vi "myRIO_BRig_RT_v0,61__PortC.vi"() -> ()   [LabVIEW 2014]
uses:
  myRIO_BRig_RT__Case_Exp_stateList.ctl
  myRIO_BRig_RT__Case_NonExp_stateList.ctl
  <vilib>/Platform/TimedLoop/XDataNode/timing_clust.ctl
  <vilib>/Platform/TimedLoop/XDataNode/nitl_modes.ctl
  <vilib>/Platform/TimedLoop/XDataNode/wakeup.ctl
  <vilib>/WebDAVClient/Advanced/SessionHandle.ctl
  <vilib>/myRIO/Common/Instrument Driver Framework/myRIO v1.0/UART/vis/myRIO v1.0 Close UART.vi
  <vilib>/FPGAPlugInAG/myRIO-1900/niLvFpga_Open_myRIO-1900.vi
  <vilib>/rvi/interface/common/dynamic/niFpgaDynamicAddResources.vi
  <vilib>/Utility/error.llb/Error Cluster From Error Code.vi
  <vilib>/rvi/errors/niLvFpgaAdjustHostInterfaceError.vi
  <vilib>/FPGAPlugInAG/Dynamic/niLvFpga_Close_Dynamic.vi
  <vilib>/myRIO/Common/Instrument Driver Framework/Utilities/vis/FPGA Ref Manager.vi
  <vilib>/myRIO/Common/Instrument Driver Framework/myRIO v1.0/myRIO v1.0 Reset FPGA.vi
  <vilib>/myRIO/Common/Instrument Driver Framework/myRIO v1.0/IRQ/vis/myRIO v1.0 IRQ Info FGV.vi
  <vilib>/myRIO/Common/Instrument Driver Framework/myRIO v1.0/IRQ/vis/myRIO v1.0 Timer IRQ Info FGV.vi
  <vilib>/myRIO/Common/Instrument Driver Framework/myRIO v1.0/IRQ/vis/myRIO v1.0 ISR Agent.vi
  <vilib>/rvi/interface/nirviOpenFPGA/nirviOpenFPGA.xnode
  FPGA Bitfiles/myRIOBRig_FPGATarget_myRIOBRigFPGAv3,_rBLkV1r30v0.lvbitx
  myRIO_BRig_FPGA_v3,51__PortC__testSinwave.vi
  <vilib>/rvi/interface/nirviReadWriteControl/nirviReadWriteControl.xnode
  <vilib>/Platform/TimedLoop/XDataNode/XDataNode.xnode
  <vilib>/rvi/interface/nirviCloseFPGA/nirviCloseFPGA.xnode
  <vilib>/Platform/TimedLoop/XDataNode/XDNodeRunTimeDep.lvlib
  <vilib>/rvi/interface/Simulation/niFpgaSimulationCallBeginRW.vi
  <vilib>/myRIO/Instrument Drivers/Utilities/Utilities.lvlib
  <vilib>/WebDAVClient/NI_WebDAV.lvlib
  NiFpgaLv.dll
panel:
  out "error out 5":errorcluster
  in  "get_countPerMS":bool
  in  "count_warmup_R_reset":bool
  in  "count_warmup_L_reset":bool
  out "count_warmup_R":u16
  out "count_warmup_L":u16
  out "SolenoidReward":bool
  in  "SolenoidProbability_L":u16=50 caption="Reward Time [ms]" min=1 max=1000 step=1
  in  "SolenoidProbability_R":u16=50 caption="Reward Time [ms]" min=1 max=1000 step=1
  out "output_PortA":dbl
  out "error out 4":errorcluster
  in  "laser_power_step":dbl
  in  "laser_power_max":dbl
  in  "Recording_p2":bool
  in  "Recording":bool
  out "error out 3":errorcluster
  out "error out 2":errorcluster
  in  "laser_power_min":dbl
  in  "f_millisec2count":dbl=159.0
  in  "laser_Tshutter":dbl=2.0
  in  "laser_Freq":dbl=10.0
  in  "laser_Tpeak":dbl=2.0
  in  "laser_duration":u16
  out "error out":errorcluster
  in  "LC_Cue1_All_Count":u16
  in  "LC_Cue1_First_Count":u16
  in  "LC_Cue1_All_delayOpt":bool
  in  "LC_ENL1_All_delayOpt":bool
  in  "LC_ENL1_All_Count":u16
  in  "LC_ENL1_First_Count":u16
  in  "LC_Cue1_First_delayOpt":bool
  in  "LC_ENL1_First_delayOpt":bool
  in  "Tcycle_Cue_max":u16=1000 caption="Max" min=5 max=5000 step=5
  in  "Tcycle_Cue_min":u16=1000 caption="Min" min=5 max=5000 step=5
  in  "SendData":bool
  out "cSpout":enum16{"Left", "Right"}(ring) caption="Left or Right Spout"
  out "A4":u32 caption="LickCounter_Right"
  out "A2":u32 caption="LickCounter_Left"
  in  "laserResponse_wrong_LED":bool
  out "error_initTrial":errorcluster
  out "error_Selection_pre":errorcluster
  out "error_Selection":errorcluster
  out "SelectWrong":bool
  out "SelectReward":bool
  in  "Left(F)_or_Right(T)":bool
  in  "ignoreWrong":bool
  in  "SelectionState":bool
  in  "laserResponse_wrong":bool
  in  "laserResponse_reward":bool
  in  "laserResponse_reward_LED":bool
  out "nRewards_Right":u16 caption="# Rewards Total (Right)"
  out "nRewards_Left":u16 caption="# Rewards Total (Left)"
  out "nRewards_cur":u16 caption="# Rewards in Current Block"
  out "TpB_target":u16 caption="Target Trials Per Block"
  out "cState_NonExp":T1 caption="WarmUp State"
  out "iBlock":u16 caption="Current Block"
  out "cState":T2 caption="Experimental State"
  out "iTrial":u16 caption="Current Trial"
  in  "warmupType":u8(slide) max=2 step=1 scale=0.0..2.0
  in  "TestConnection":bool
  in  "warmup":bool caption="WarmUp"
  in  "Data Set Prefix":string="Exp1_TM2"
  out "Connected To Host?":bool
  in  "Host Password":string="sabalab"
  in  "Host UserName":string="Test2"
  in  "sp_RightSpout":u16(slide)=2 max=2 step=1 scale=0.0..2.0
  in  "sp_LeftSpout":u16(slide)=2 max=2 step=1 scale=0.0..2.0
  in  "BUR_max":u16 caption="Count Reward Structure  (0 = off)"
  in  "LC_Wrong_Probability":u16
  in  "LC_Wrong_Trial":u16(slide) max=2 step=1 scale=0.0..2.0
  in  "LC_Wrong_Block":u16(slide) max=2 step=1 scale=0.0..2.0
  in  "LC_Wrong_OnOff":bool
  in  "LC_Reward_Probability":u16
  in  "LC_Reward_Trial":u16(slide) max=2 step=1 scale=0.0..2.0
  in  "LC_Reward_Block":u16(slide) max=2 step=1 scale=0.0..2.0
  in  "LC_Reward_OnOff":bool
  in  "LC_Cue1_All_Probability":u16
  in  "LC_Cue1_All_Block":u16(slide) max=2 step=1 scale=0.0..2.0
  in  "LC_Cue1_All_OnOff":bool
  in  "LC_Cue1_First_Probability":u16
  in  "LC_Cue1_First_Block":u16(slide) max=2 step=1 scale=0.0..2.0
  in  "LC_Cue1_First_OnOff":bool
  in  "LC_ENL1_All_Probability":u16 max=100 step=1
  in  "LC_ENL1_All_Block":u16(slide) max=2 step=1 scale=0.0..2.0
  in  "LC_ENL1_All_OnOff":bool
  in  "LC_ENL1_First_Probability":u16 max=100 step=1
  in  "LC_ENL1_First_Block":u16(slide) max=2 step=1 scale=0.0..2.0
  in  "Tcycle_Timeout":u16=1000 caption="Timeout Time [ms]" min=10 max=10000 step=1
  in  "Tcycle_Wrong":u16=1000 caption="Wrong Time [ms]" min=10 max=10000 step=1
  in  "Tcycle_Selection":u16=1000 caption="Answer Time [ms]" min=1 max=10000 step=1
  in  "Tcycle_RewardPost":u16=1000 caption="Consumption Time [ms]" min=250 max=10000 step=250
  in  "Tcycle_Reward_L":u16=500 caption="Reward Time [ms]" min=1 max=1000 step=1
  in  "Tcycle_Reward_R":u16=500 caption="Reward Time [ms]" min=1 max=1000 step=1
  in  "TpB_Max_R":u16=4 caption="Max TrialsPerBlock" min=1 max=12 step=1
  in  "TpB_Min_R":u16=4 caption="Min TrialsPerBlock" min=1 max=12 step=1
  in  "TpB_Max_L":u16=4 caption="Max TrialsPerBlock" min=1 max=12 step=1
  in  "TpB_Min_L":u16=4 caption="Min TrialsPerBlock" min=1 max=12 step=1
  in  "BUR_min":u16 caption="Count Reward Structure  (0 = off)"
  in  "TrialUntilReward":bool caption="Ignore Wrong Selection"
  in  "CueCycles":u16=1 caption="Cue Structure" min=1 max=1 step=1
  in  "MTrig_Laser_Tcycle":u16=10 caption="Time [ms]"
  in  "MTrig_Laser_trig":bool
  in  "MTrig_Audio_trig__R":bool caption="Trigger Audio"
  in  "MTrig_Audio_trig__L":bool caption="Trigger Audio"
  in  "RewCalib_Trig_R":bool caption="Calibrate_R"
  in  "RewCalib_Trig_L":bool caption="Calibrate_L"
  in  "MTrig_Solenoid_Tcycle__R":u16=300 caption="Time [ms]"
  in  "MTrig_Solenoid_Tcycle__L":u16=300 caption="Time [ms]"
  in  "MTrig_Solenoid_trig__R":bool caption="Solenoid"
  in  "MTrig_Solenoid_trig__L":bool caption="Solenoid"
  in  "STOP_abort":bool caption="Stop LabView\n(Stops myRio and FPGA)"
  in  "STOP_endBlock":bool caption="Stop Experiment\n@ End of Block"
  in  "STOP_endTrial":bool caption="Stop Experiment\n@ End of Trial"
  in  "START":bool caption="Start Experiment"
  in  "Tcycle_CuePenalty":u16=1000 caption="Penalty" min=1 max=10000 step=1
  in  "Audio_Amp__R":u16=100 caption="Amp"
  in  "Audio_Freq__R":u8=5 caption="Freq [kHz]" max=14 step=1
  in  "Audio_Amp__L":u16=100 caption="Amp"
  in  "Audio_Freq__L":u8=5 caption="Freq [kHz]" max=14 step=1
  in  "LC_Wrong_Tdelay":u16
  in  "LC_Cue1_All_Tdelay":u16
  in  "LC_ENL1_All_Tdelay":u16
  in  "LC_Reward_Tdelay":u16
  in  "LC_Cue1_First_Tdelay":u16
  in  "LC_ENL1_First_Tdelay":u16
  in  "LC_ENL1_First_OnOff":bool
  in  "Tcycle_ENLPenalty":u16=100 caption="Penalty" min=10 max=10000 step=10
  in  "Tcycle_ENL_max":u16=1000 caption="Max" min=250 max=10000 step=250
  in  "Tcycle_ENL_min":u16=1000 caption="Min" min=250 max=10000 step=250
  # "Communication (Host PC)"
  # "WarmUp"
  # "Experimental Run"
  # "Current State"
  # "Laser Control\n\n                               On/Off      Block        Probability [%]   Delay [ms]                              Count"
  # "Cue then reward (no lick)\n \nLeft                    Right"
  # "Recording Rig"
  # "FPGA Conv."
  # "Enforced\nNonLick\n      1"
  # "from end"
  # "Switch\nTrial"
  # "FPGA count per ms"
  # "from start"
  # "from end"
  # "NonSwitch\nTrials"
  # "from start"
  # "Manual Control"
  # "Cue 1"
  # "Solenoid\n \nLeft                    Right"
  # "Speaker\n \nLeft                    Right"
  # "Laser"
  # "from end"
  # "Switch\nTrial"
  # "from start"
  # "from end"
  # "NonSwitch\nTrials"
  # "from start"
  # "Time = Cue Min"
  # "Selection Reward"
  # "Task Timing [ms]"
  # "Speaker Settings"
  # "Laser Settings"
  # "Selection Wrong"
  # "Left                  Right"
  # "Enforced NonLick"
  # "Frequency\n[kHz]"
  # "Duration         Frequency       Peak Width           Shutter\n    [ms]                   [Hz]                    [ms]                    [ms]"
  # "Task Structure"
  # "Spout Selection Control"
  # "Amp\n(0 - 32,000)"
  # "Master Structure"
  # "Cue"
  # "Answer Time\n         [ms]\n\n  \nWrong Choice Penalty\n         [ms]\n \n \nChoice Timeout Penalty\n         [ms]"
  # "Min\n \n  \nMax"
  # "Laser Power [V]\n      Min                   Max                   Step                 Current"
  # "Speaker\nPattern\nDuring Cue"
  # "(1) = Switching\n(2) = Two Choice"
  # "Reward Control\n                 Left              Right"
  # "Min"
  # "Max"
  # "Trial Per Block Structure\n       Left                    Right"
  # "Reward Time\n         [ms]\n\nWater Prob"
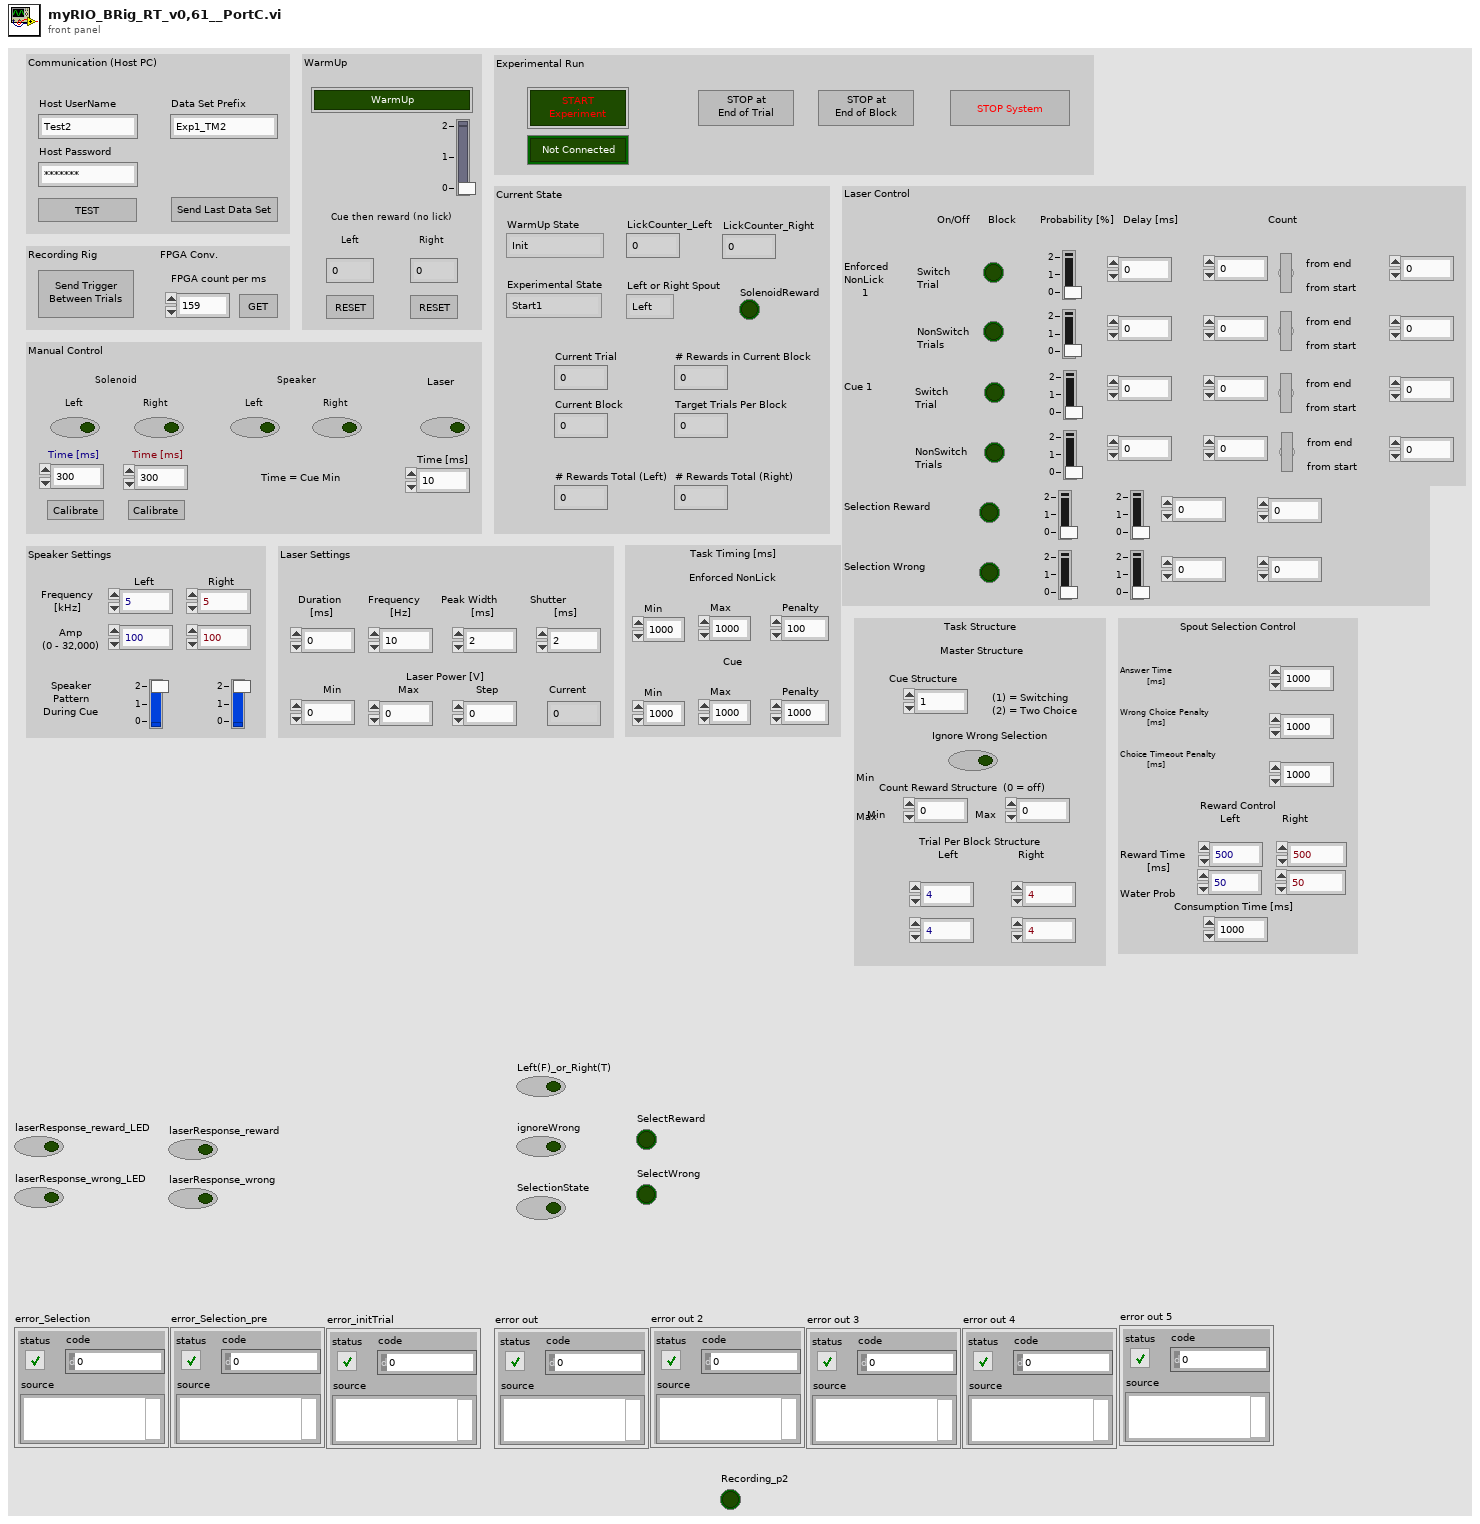
[diagram p1: front panel]
types:
  T1 = typedef "myRIO_BRig_RT__Case_NonExp_stateList.ctl" = enum16{"Init", "UploadSettings_pre", "UploadSettings_Read_dataExp", "UploadSettings_dataExp_1", "UploadSettings_Read_dataLC", "UploadSettings_dataLC_1", "UploadSettings_dataLC_2", "UploadSettings_Read_dataMTrig", "UploadSettings_dataMTrig_1", "UploadSettings_post", "Idle_pre", "IdleEmpty", "IdleEmpty2", "IdleEmpty3", "IdleEmpty4", "Idle", "Idle_2", "Idle_3", "Idle_4", "Idle_post", "Cue_pre__pre", "Cue_pre", "Cue", "Cue_post", "RewardCalibration_pre", "DispenseWater_pre__pre", "DispenseWater_pre", "DispenseWater", "DispenseWater_post", "TestConnection", "SendData", "Get_FPGA_count_per_ms", "End"}
  T2 = typedef "myRIO_BRig_RT__Case_Exp_stateList.ctl" = enum16{"Start1", "Start2", "Start3", "saveSettings1", "saveSettings2", "saveSettings3", "saveSettings4_LC_ENL", "saveSettings5_LC_Cue", "saveSettings6_LC_Other", "setSettings_Audio", "setSettings_Laser", "initBlock_pre", "initBlock", "initBlock2", "initBlock_post", "initTrial_pre", "initTrial", "initTrial2", "initTrial3", "initTrial4", "initTrial_LC_ENL1", "initTrial_LC_Cue1", "initTrial_post", "ENL1_pre", "ENL1", "ENL1_post", "ENL1Penalty_pre", "ENL1Penalty", "ENL2_pre", "ENL2", "ENL2Penalty_pre", "ENL2Penalty", "Cue1_pre", "Cue1", "Cue1_post", "Cue1Penalty_pre", "Cue1Penalty", "Cue2_pre", "Cue2", "Cue2Penalty_pre", "Cue2Penalty", "Selection_pre", "Selection", "Select_post", "SelectReward_pre", "SelectReward", "SelectRewardPost_pre", "SelectRewardPost", "SelectWrong_pre", "SelectWrong", "SelectWrong_post", "SelectTimeout_pre", "SelectTimeout", "SelectTimeout_post", "endTrial_pre", "endTrial1", "endTrial2", "endTrial3", "endTrial_post", "endBlock_pre", "endBlock", "endBlock_post", "endExp", "commConnect", "commUpload_pre", "commUpload_dataBlock", "commUpload_dataCurrent", "commUpload_dataExp", "commUpload_dataLC", "commUpload_dataTrial", "commUpload_post", "saveData_pre", "saveData_dataBlock", "saveData_dataCurrent", "saveData_dataExp", "saveData_dataLC", "saveData_dataTrial", "saveData_post", "empty_endBlock1", "empty_endBlock2", "empty_endTrial1", "empty_endTrial2", "empty_endTrial3", "empty_endTrial4", "empty_endTrial5"}
  T3 = typedef "XDNodeRunTimeDep.lvlib/timing_clust.ctl" = cluster{"Expected End [f-1]":u64, "Actual End [f-1]":u64, "Finished Late? [f-1]":bool, "Expected End [i-1]":u64, "Actual End [i-1]":u64, "Finished Late? [i-1]":bool, "Expected Start [i]":u64, "Actual Start [i]":u64, "Expected Start [f]":u64, "Actual Start [f]":u64, "Source Name":string, "Structure Name":string, "Period":i64, "Deadline":i64, "Offset":i64, "Start":i64, "Priority":i32, "Timeout":i32, "Mode":T4, "Wakeup Reason":T5, "Error":errorcluster, "Source Type":string, "Secondary Source Type":string, "Global End Time":u64, "Global Start Time":u64, "Frame Duration":u64, "Iteration Duration":u64, "Assigned CPU":i32, "I/O Scan Engine Mode":u32}
  T4 = typedef "XDNodeRunTimeDep.lvlib/nitl_modes.ctl" = enum32{"No Change", "Process missed periods, maintain original phase", "Discard missed periods, maintain original phase", "Process missed periods, ignore original phase", "Discard missed periods, ignore original phase"}
  T5 = typedef "XDNodeRunTimeDep.lvlib/wakeup.ctl" = enum32{"Normal", "Aborted", "Asynchronous wakeup", "Timing source error", "Timed loop error", "Timeout"}
  T6 = typedef "NI_WebDAV.lvlib/SessionHandle.ctl" = refnum<k1>
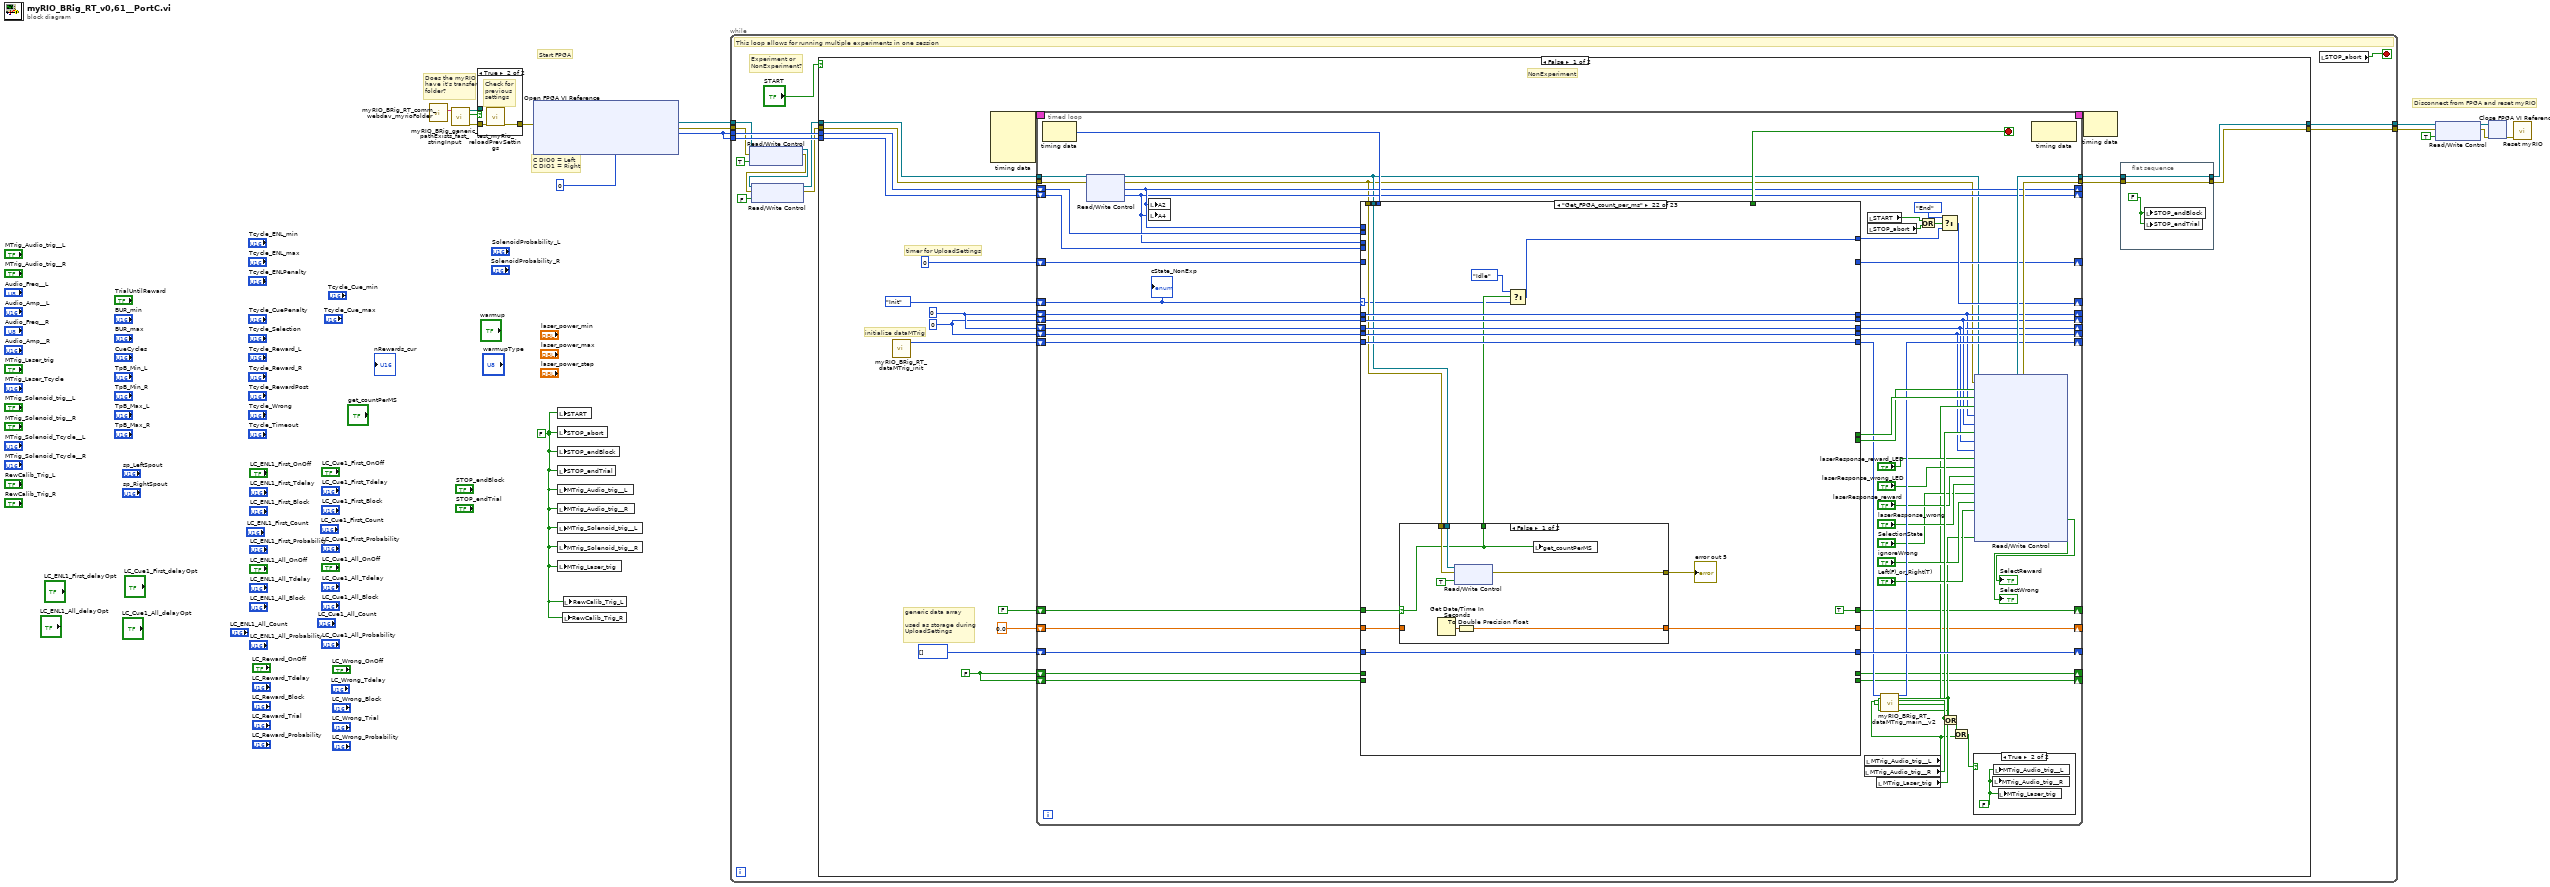
[diagram p0: block diagram]
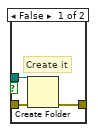
[diagram p2: hidden frame]
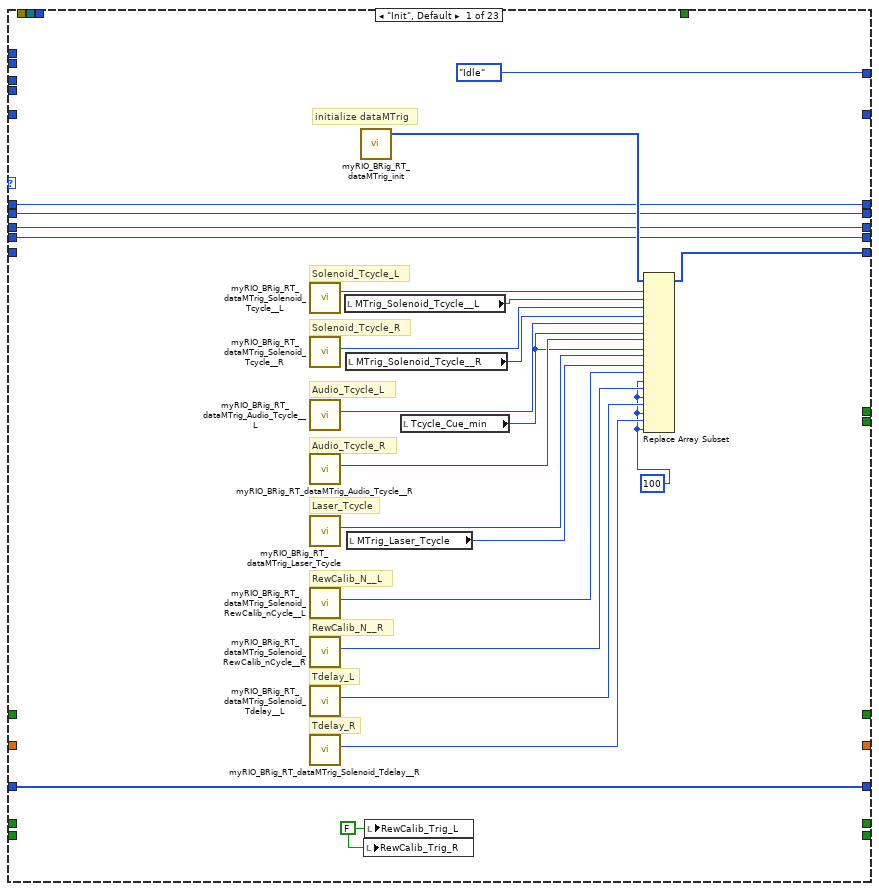
[diagram p4: hidden frame]
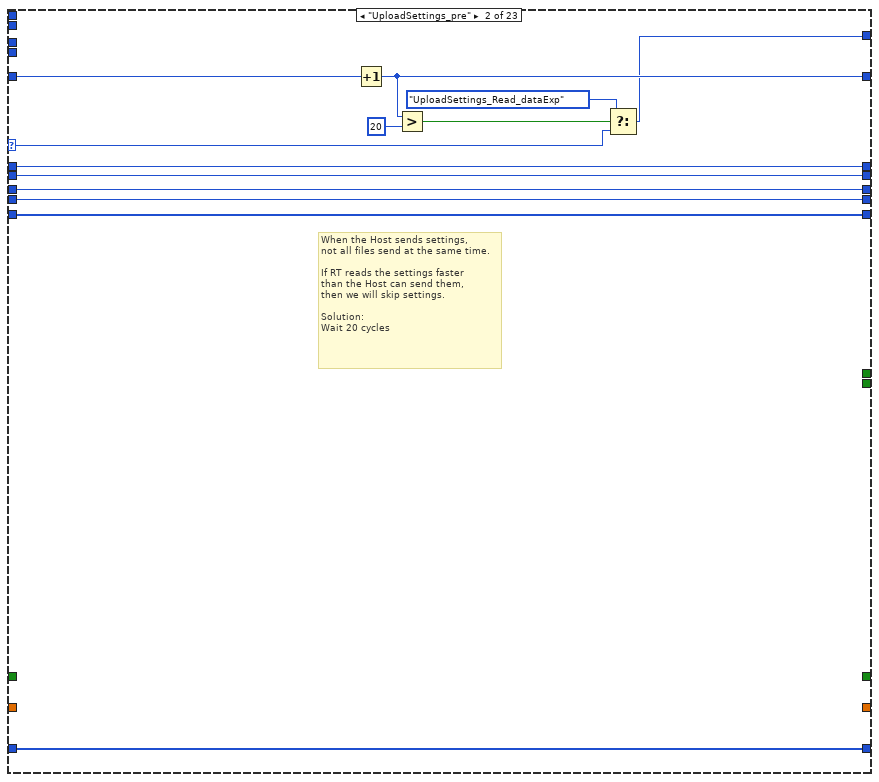
[diagram p5: hidden frame]
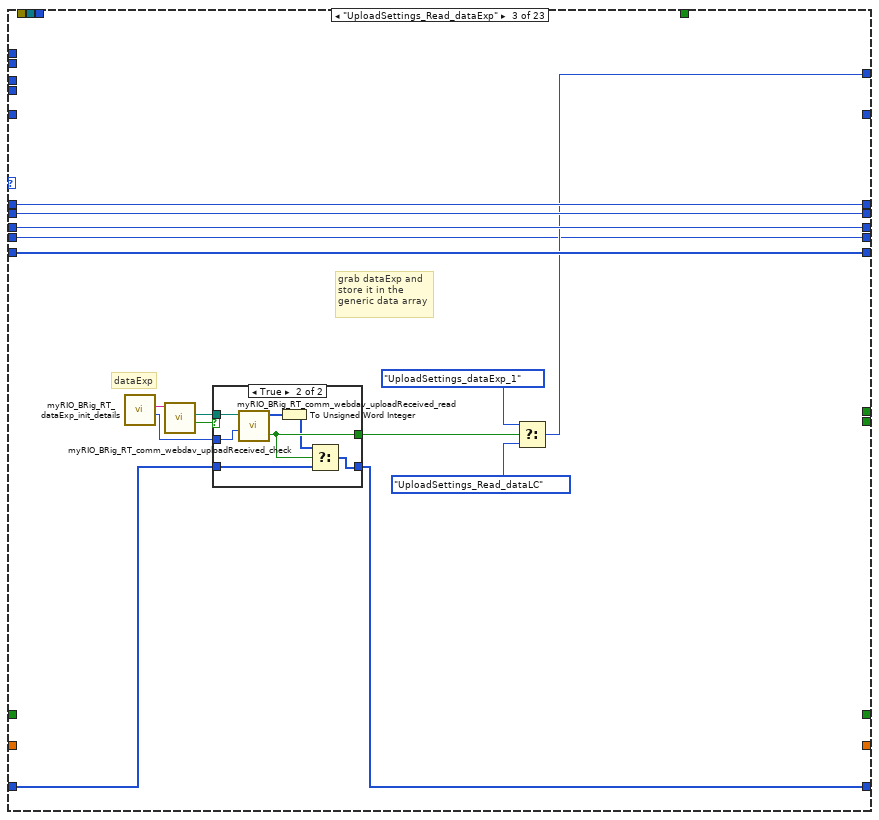
[diagram p6: hidden frame]
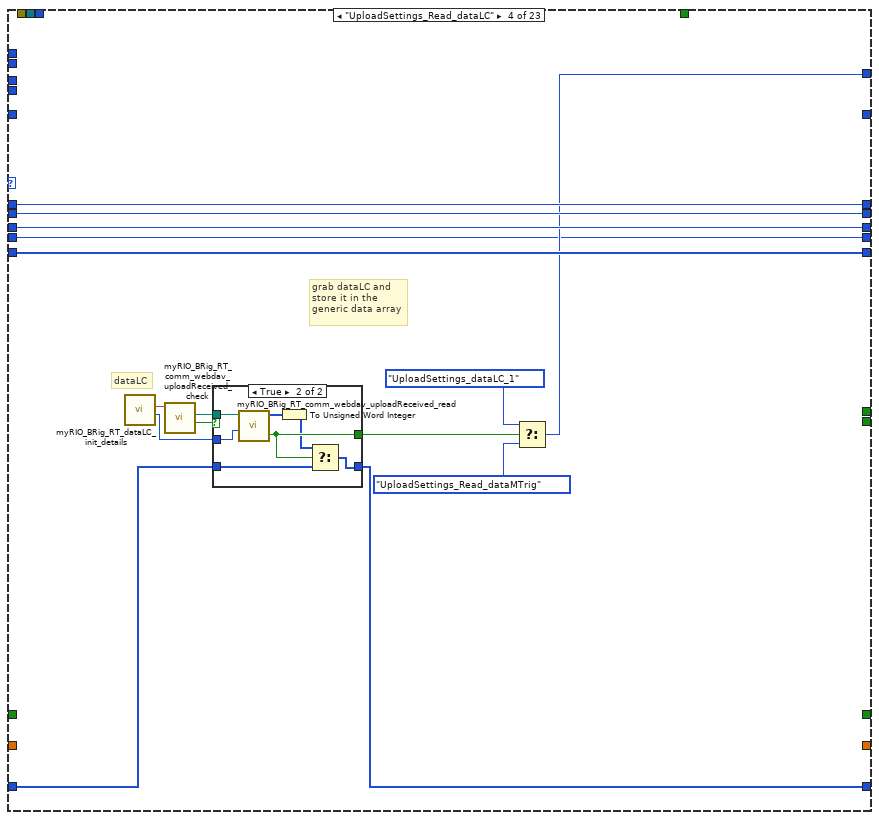
[diagram p8: hidden frame]
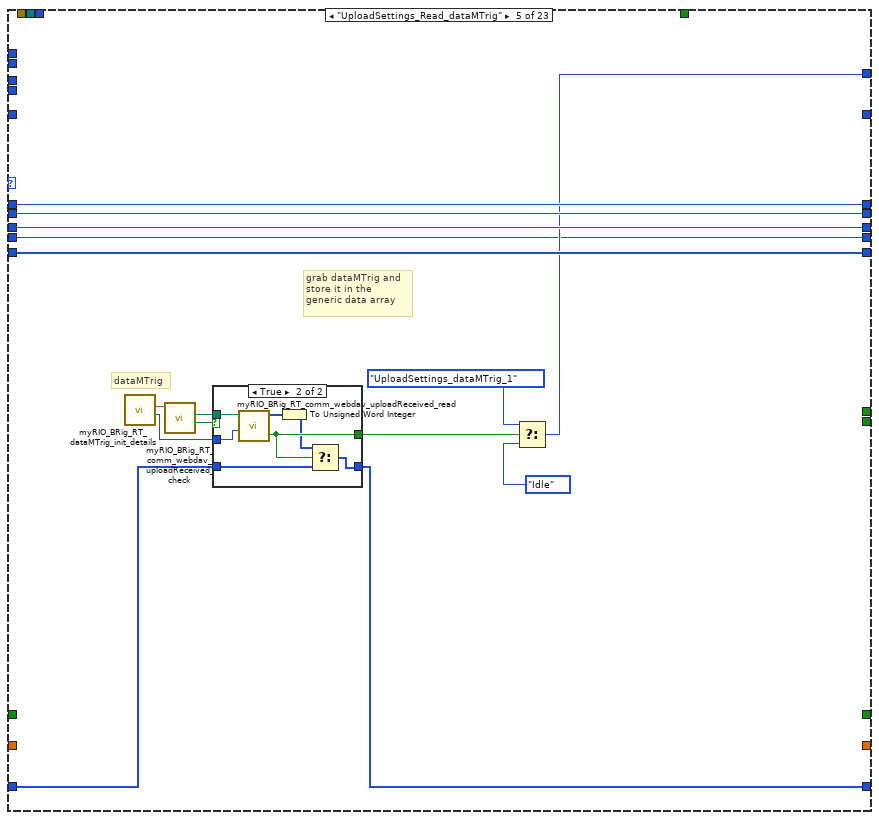
[diagram p10: hidden frame]
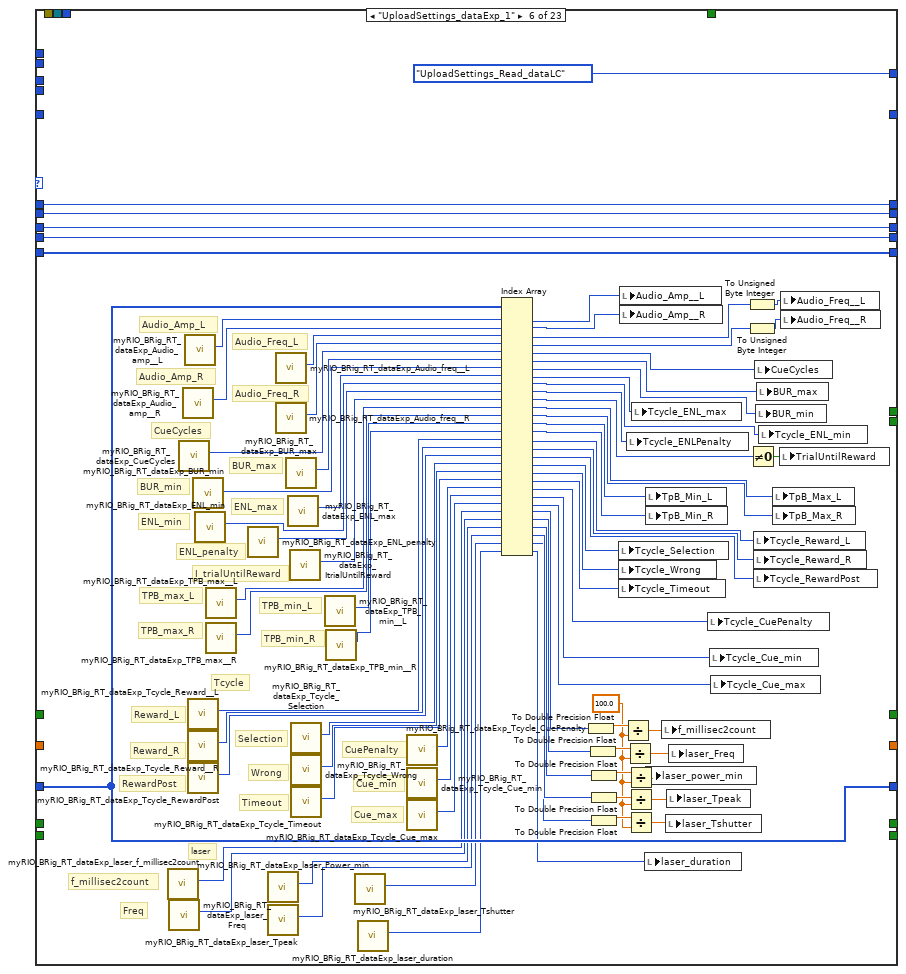
[diagram p12: hidden frame]
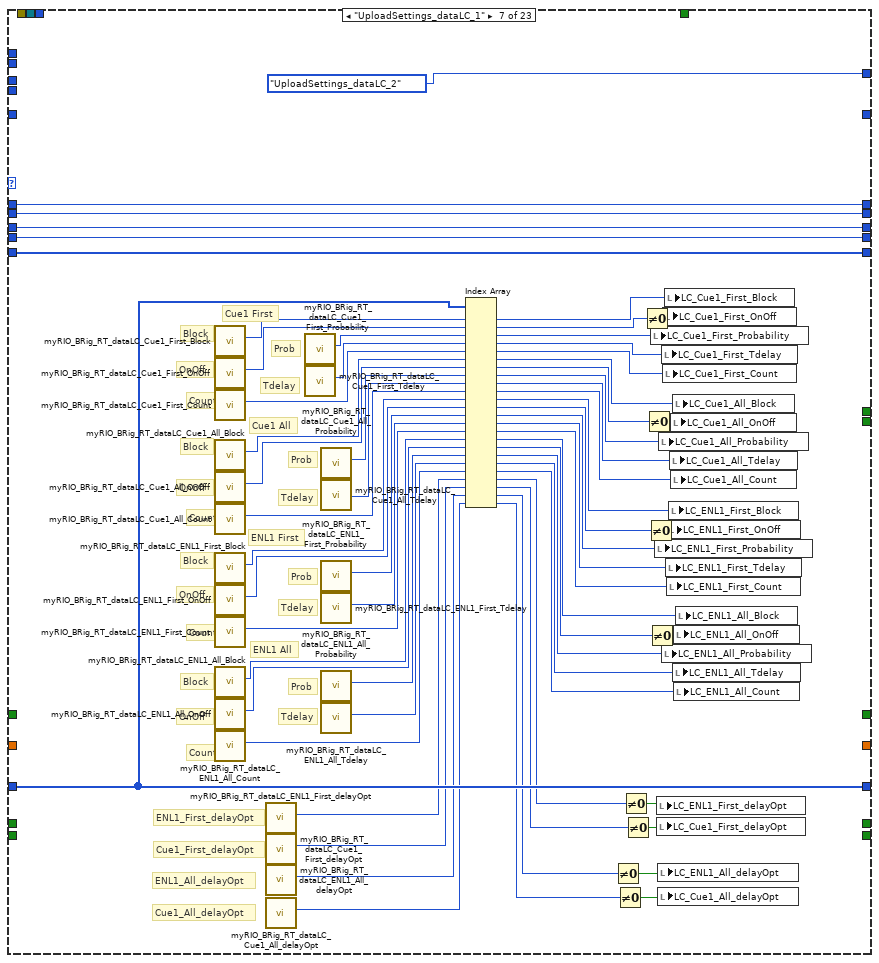
[diagram p13: hidden frame]
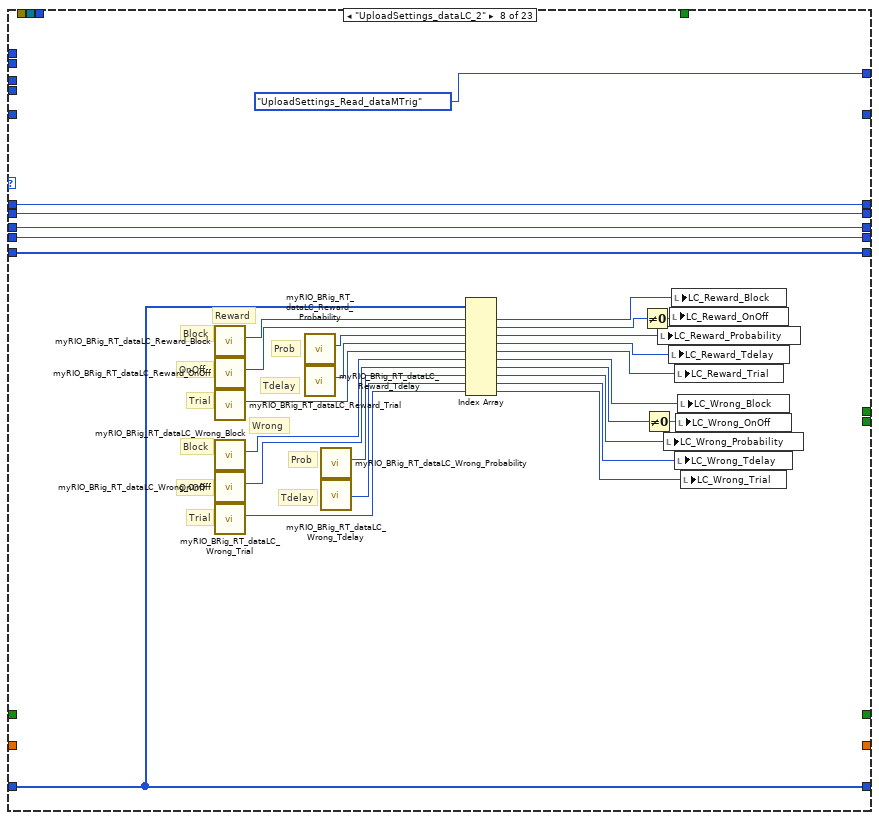
[diagram p14: hidden frame]
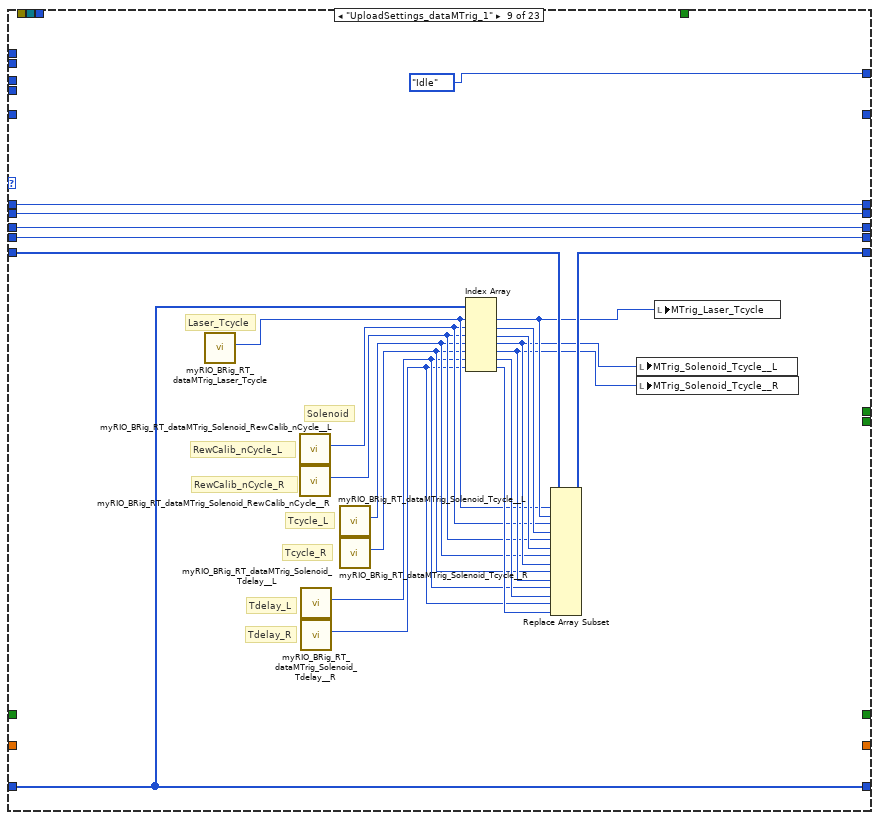
[diagram p15: hidden frame]
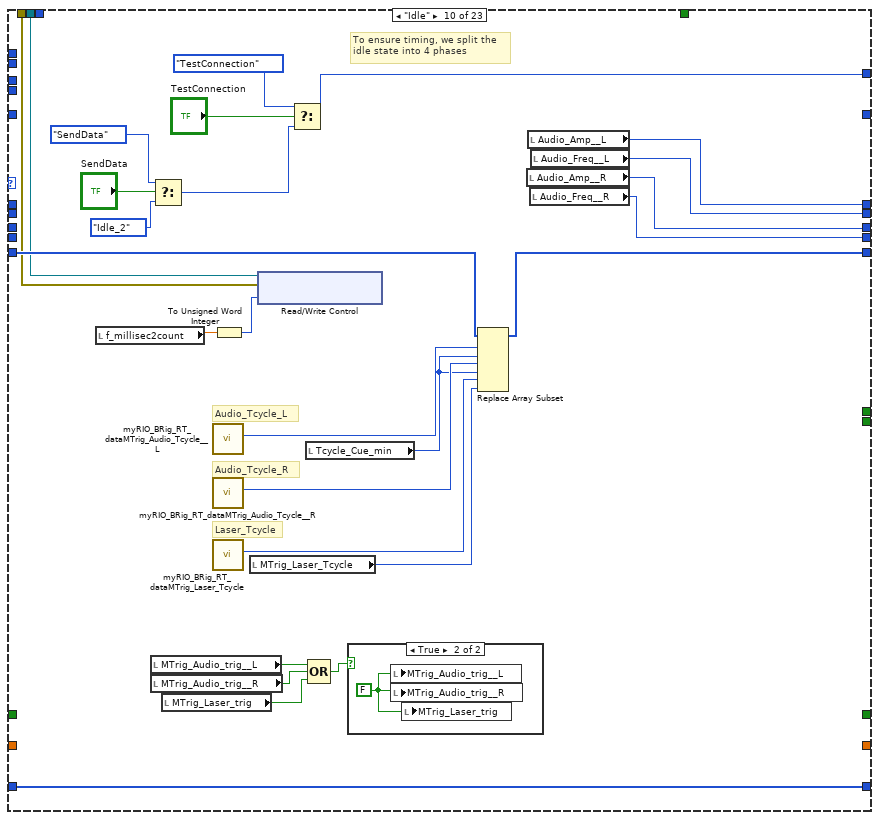
[diagram p16: hidden frame]
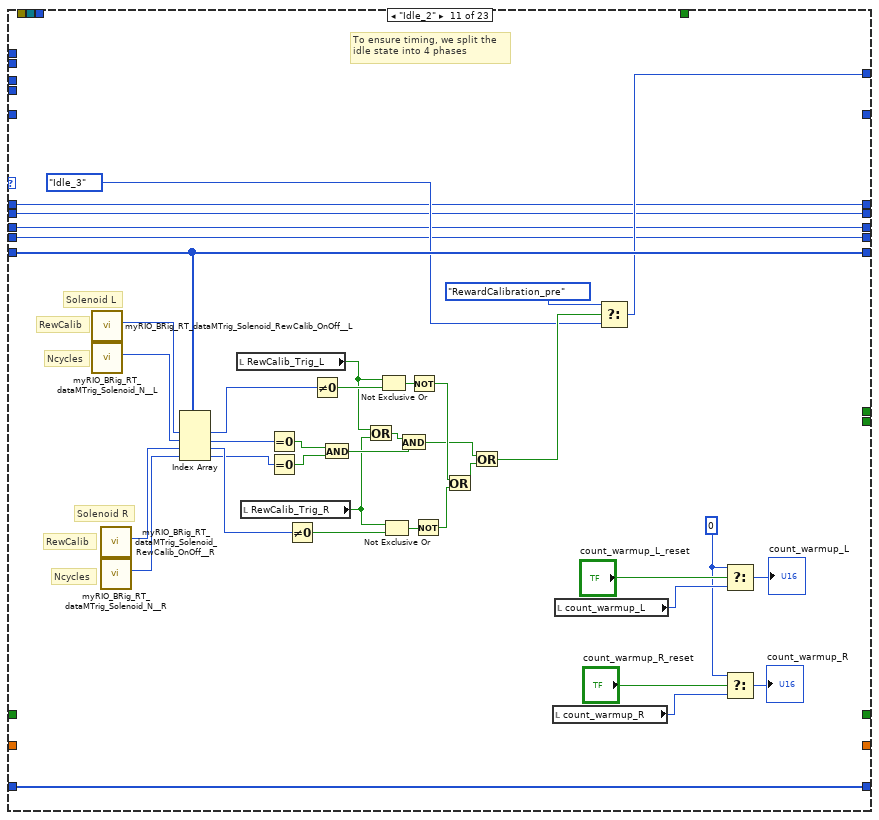
[diagram p18: hidden frame]
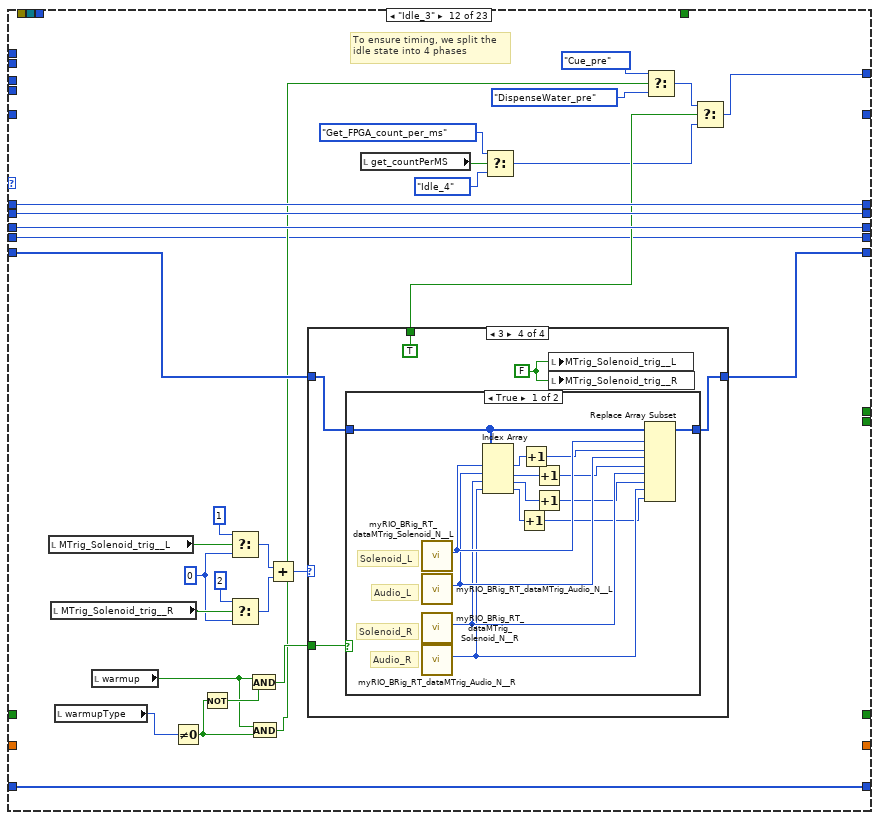
[diagram p19: hidden frame]
diagram:
  w9 = u32 0
  w6 = FALSE
  # "Does the myRIO\nhave it's transfer\nfolder?"
  # "C DIO0 = Left\nC DIO1 = Right"
  # "Start FPGA"
  # "Disconnect from FPGA and reset myRIO"
  n1 = call "myRIO_BRig_RT_comm_webdav_myrioFolder.vi"() -> ("output_myrioFolder"=w4:string)  [unwired: 11 in]
  n2 = call "myRIO_BRig_generic_pathExists_fast_stringInput.vi"("input_filePath"=w4) -> ("output_error"=w3:errorcluster, "output_Iexist"=w2:bool, "output_filePath"=w1:path)  [unwired: 8 in]
  n3 = case shown="True" w2 {
    tunnel: w1 -> [w18 _]
    tunnel: w3 -> [w17 w20]
    tunnel: [w16 w19] -> w5
    frame False {
      # "Create it"
      n4 = Create Folder(path (use dialog)=w18, error in=w17) -> (error out=w16:errorcluster)  [unwired: 1 in, 2 out]
    }
    frame True {
      # "Check for\nprevious\nsettings"
      n5 = call "test_myRio_reloadPrevSettings.vi"("input_error"=w20) -> ("output_error"=w19:errorcluster)  [unwired: 10 in]
    }
  }
  n6 = xnode "Open FPGA VI Reference"("error in"=w5) -> ("FPGA VI Reference Out"=w11:refnum<k20>, "error out"=w10:errorcluster)  [unwired: 1 in]
  n7 = local write "START"(w6) -> ()
  n8 = local write "STOP_abort"(w6) -> ()
  n9 = local write "STOP_endBlock"(w6) -> ()
  n10 = local write "STOP_endTrial"(w6) -> ()
  n11 = local write "MTrig_Audio_trig__L"(w6) -> ()
  n12 = local write "MTrig_Audio_trig__R"(w6) -> ()
  n13 = local write "MTrig_Solenoid_trig__L"(w6) -> ()
  n14 = local write "MTrig_Solenoid_trig__R"(w6) -> ()
  n15 = local write "MTrig_Laser_trig"(w6) -> ()
  n16 = local write "RewCalib_Trig_R"(w6) -> ()
  n17 = local write "RewCalib_Trig_L"(w6) -> ()
  n18 = while {
    tunnel: w11 -> [w24]
    tunnel: w10 -> [w29]
    tunnel: w9 -> [w32]
    tunnel: w9 -> [w31]
    tunnel: [w22] -> w8
    tunnel: [w21] -> w7
    stop <- w30 stop-if-true
    # "Experiment or\nNonExperiment?"
    # "This loop allows for running multiple experiments in one session"
    n19 = xnode "Read/Write Control"("FPGA VI Reference In"=w24, "error in"=w29, "Counts_Reset"=TRUE) -> ("FPGA VI Reference Out"=w26:refnum<k20>, "error out"=w27:errorcluster)
    n20 = xnode "Read/Write Control"("FPGA VI Reference In"=w26, "error in"=w27, "Counts_Reset"=FALSE) -> ("FPGA VI Reference Out"=w23:refnum<k20>, "error out"=w25:errorcluster)
    n21 = case shown="False" "START" {
      tunnel: w32 -> [w49 w1046]
      tunnel: w31 -> [w48 w1045]
      tunnel: w25 -> [w46 w996]
      tunnel: w23 -> [w47 w995]
      tunnel: [w44 w1042] -> w22
      tunnel: [w42 w1037] -> w21
      frame False {
        w37 = FALSE
        w38 = u8 0 ("Audio_Amp__L")
        w41 = u16 0 ("Audio_Amp__L")
        # "generic data array\n\nused as storage during\nUploadSettings"
        # "timer for UploadSettings"
        # "initialize dataMTrig"
        # "NonExperiment"
        n22 = call "myRIO_BRig_RT_dataMTrig_init.vi"() -> ("output_dataMTrig"=w50:u16[])  [unwired: 5 in]
        n23 = node-c288() -> (w53:T3)  [unwired: 4 in]
        n24 = timed-loop {
          timing: w53 -> [_]
          timing-out: [_] -> w52
          shift-right: [w101] -> _
          shift-left: w50 -> [w116]
          shift-right: [w90] -> _
          shift-left: myRIO_BRig_RT__Case_NonExp_stateList."Init" ("Enum") -> [w110]
          shift-right: [w69] -> _
          shift-left: w49 -> [w70]
          shift-right: [w67] -> _
          shift-left: w48 -> [w68]
          tunnel: [w112] -> w45
          tunnel: [w111] -> w43
          tunnel: w46 -> [w114]
          tunnel: w47 -> [w113]
          shift-right: [w109] -> _
          shift-left: u16[] [] ("output_data") -> [w108]
          shift-right: [w71] -> _
          shift-left: w41 -> [w107]
          shift-right: [w73] -> _
          shift-left: w38 -> [w106]
          shift-right: [w72] -> _
          shift-left: w41 -> [w105]
          shift-right: [w74] -> _
          shift-left: w38 -> [w75]
          shift-right: [w76] -> _
          shift-left: u16 0 ("Audio_Amp__L") -> [w77]
          shift-right: [w64] -> _
          shift-left: w37 -> [w66]
          shift-right: [w63] -> _
          shift-left: w37 -> [w65]
          shift-right: [w59] -> _
          shift-left: FALSE -> [w60]
          shift-right: [w57] -> _
          shift-left: 0.0 -> [w58]
          stop <- w117 stop-if-true
          n25 = node-c288() -> (w115:i64)  [unwired: 1 in]
          n26 = xnode "Read/Write Control"("FPGA VI Reference In"=w113, "error in"=w114) -> ("FPGA VI Reference Out"=w62:refnum<k20>, "error out"=w61:errorcluster, "A2_LickL"=w69:u32, "A4_LickR"=w67:u32)
          n27 = local write "A2"(w69) -> ()
          n28 = local write "A4"(w67) -> ()
          n29 = case shown="\"Get_FPGA_count_per_ms\"" w110 {
            selector: w110 -> [_ w150 _ _ _ _ _ _ _ _ _ _ _ _ w623 _ _ w844 _ _ _ w934 w986]
            tunnel: [myRIO_BRig_RT__Case_NonExp_stateList."Idle" ("Enum") w148 w156 w179 w202 myRIO_BRig_RT__Case_NonExp_stateList."UploadSettings_Read_dataLC" ("Enum") myRIO_BRig_RT__Case_NonExp_stateList."UploadSettings_dataLC_2" ("Enum") myRIO_BRig_RT__Case_NonExp_stateList."UploadSettings_Read_dataMTrig" ("f") myRIO_BRig_RT__Case_NonExp_stateList."Idle" ("Enum") w436 w459 w499 w587 myRIO_BRig_RT__Case_NonExp_stateList."Cue" ("t") w618 myRIO_BRig_RT__Case_NonExp_stateList."DispenseWater_pre" ("Enum") w785 w842 w869 myRIO_BRig_RT__Case_NonExp_stateList."Idle" ("Enum") myRIO_BRig_RT__Case_NonExp_stateList."Idle" ("Enum") w933 w986] -> w91
            tunnel: [w133 w144 w166 w189 w212 w304 w367 w396 w416 w442 w474 w507 w585 w604 w624 w694 w822 w849 w880 w922 w932 w949 w984] -> w102
            tunnel: [_ _ _ _ _ _ _ _ _ _ _ _ _ _ _ _ _ _ _ _ _ _ TRUE] -> w117
            tunnel: w116 -> [_ w144 w166 w189 w212 w304 w367 w396 w417 w441 w474 w508 w585 w605 w625 w680 w818 w850 w881 w922 w932 w949 w984]
            tunnel: w115 -> [_ _ _ _ _ _ _ _ _ _ _ _ _ _ _ _ _ w854 _ _ _ _ _]
            tunnel: [w123 w143 w157 w180 w203 w250 w320 w369 w398 w431 w455 w493 w581 w594 w633 w672 w770 w827 w862 w911 w927 w945 w980] -> w109
            tunnel: w108 -> [w123 w143 w158 w181 w204 w250 w320 w369 w398 w431 w455 w493 w581 w594 w633 w672 w770 w827 w862 w911 w927 w945 w980]
            tunnel: [w126 w146 w168 w191 w214 w301 w365 w371 w414 w424 w457 w502 w583 w611 w637 w674 w824 w859 w886 w913 w929 w947 w982] -> w73
            tunnel: [w127 w147 w169 w192 w215 w302 w366 w372 w415 w438 w458 w501 w582 w613 w636 w675 w825 w860 w887 w914 w930 w948 w983] -> w71
            tunnel: [w125 w145 w167 w190 w213 w300 w364 w370 w413 w437 w456 w503 w584 w610 w638 w673 w823 w858 w885 w912 w928 w946 w981] -> w72
            tunnel: w107 -> [w127 w147 w169 w192 w215 w302 w366 w372 w415 _ w458 w501 w582 w613 w636 w675 w825 w860 w887 w914 w930 w948 w983]
            tunnel: w106 -> [w126 w146 w168 w191 w214 w301 w365 w371 w414 _ w457 w502 w583 w611 w637 w674 w824 w859 w886 w913 w929 w947 w982]
            tunnel: w105 -> [w125 w145 w167 w190 w213 w300 w364 w370 w413 _ w456 w503 w584 w610 w638 w673 w823 w858 w885 w912 w928 w946 w981]
            tunnel: [_ _ _ _ _ _ _ _ _ _ _ _ _ _ _ _ _ w851 _ _ _ _ _] -> w104
            tunnel: [_ _ _ _ _ _ _ _ _ _ _ _ _ _ _ _ _ w833 _ _ _ _ _] -> w103
            tunnel: w77 -> [_ w154 _ _ _ _ _ _ _ _ _ _ _ _ _ _ _ _ _ _ _ _ _]
            tunnel: [_ w153 _ _ _ _ _ _ _ _ _ _ _ _ _ _ _ _ _ _ _ _ _] -> w76
            tunnel: w75 -> [w119 w142 w155 w178 w201 w224 w305 w368 w397 _ w454 w492 w580 w593 w632 w671 w769 w826 w861 w910 w923 w944 w979]
            tunnel: [w119 w142 w155 w178 w201 w224 w305 w368 w397 w423 w454 w492 w580 w593 w632 w671 w769 w826 w861 w910 w923 w944 w979] -> w74
            tunnel: w70 -> [_ _ _ _ _ _ _ _ _ _ _ _ _ _ w629 _ _ _ _ _ _ _ _]
            tunnel: w69 -> [_ _ _ _ _ _ _ _ _ _ _ _ _ _ w630 _ _ _ _ _ _ _ _]
            tunnel: w68 -> [_ _ _ _ _ _ _ _ _ _ _ _ _ _ w627 _ _ _ _ _ _ _ _]
            tunnel: w67 -> [_ _ _ _ _ _ _ _ _ _ _ _ _ _ w628 _ _ _ _ _ _ _ _]
            tunnel: w66 -> [_ _ _ _ _ _ _ _ _ _ _ _ _ _ w615 _ _ _ _ _ _ _ _]
            tunnel: w65 -> [_ _ _ _ _ _ _ _ _ _ _ _ _ _ w614 _ _ _ _ _ _ _ _]
            tunnel: [_ _ _ _ _ _ _ _ _ _ _ _ _ w592 w615 _ _ _ _ _ _ _ _] -> w64
            tunnel: [_ _ _ _ _ _ _ _ _ _ _ _ _ w591 w614 _ _ _ _ _ _ _ _] -> w63
            tunnel: w62 -> [_ _ _ _ _ _ _ _ _ w420 _ _ _ _ _ _ _ _ _ _ _ w939 _]
            tunnel: w61 -> [_ _ _ _ _ _ _ _ _ w419 _ _ _ _ _ _ _ _ _ _ _ w938 _]
            tunnel: w60 -> [_ _ _ _ _ _ _ _ _ _ _ _ _ _ _ _ _ _ _ _ _ w943 _]
            tunnel: [_ _ _ _ _ _ _ _ _ _ _ _ _ _ _ _ _ _ _ _ _ TRUE _] -> w59
            tunnel: w58 -> [_ _ _ _ _ _ _ _ _ _ _ _ _ _ _ _ _ _ _ _ _ w941 _]
            tunnel: [_ _ _ _ _ _ _ _ _ _ _ _ _ _ _ _ _ _ _ _ _ w940 _] -> w57
            frame "Init", Default {
              w124 = FALSE ("RewCalib_Trig_L")
              w120 = u16 100 ("new element/subarray")
              # "Tdelay_R"
              # "Tdelay_L"
              # "RewCalib_N__R"
              # "RewCalib_N__L"
              # "Solenoid_Tcycle_R"
              # "Solenoid_Tcycle_L"
              # "Laser_Tcycle"
              # "Audio_Tcycle_R"
              # "Audio_Tcycle_L"
              # "initialize dataMTrig"
              n30 = call "myRIO_BRig_RT_dataMTrig_Solenoid_Tcycle__L.vi"() -> ("output_Solenoid_Tcycle__L"=w135:i32)  [unwired: 11 in]
              n31 = call "myRIO_BRig_RT_dataMTrig_Solenoid_Tcycle__R.vi"() -> ("output_Solenoid_Tcycle__R"=w136:i32)  [unwired: 11 in]
              n32 = call "myRIO_BRig_RT_dataMTrig_Audio_Tcycle__L.vi"() -> ("output_Audio_Tcycle__L"=w137:i32)  [unwired: 11 in]
              n33 = call "myRIO_BRig_RT_dataMTrig_Audio_Tcycle__R.vi"() -> ("output_Audio_Tcycle__R"=w138:i32)  [unwired: 11 in]
              n34 = call "myRIO_BRig_RT_dataMTrig_Laser_Tcycle.vi"() -> ("output_Laser_Tcycle"=w139:i32)  [unwired: 11 in]
              n35 = call "myRIO_BRig_RT_dataMTrig_Solenoid_RewCalib_nCycle__L.vi"() -> ("output_Solenoid_RewCalib_nCycle__L"=w131:i32)  [unwired: 11 in]
              n36 = call "myRIO_BRig_RT_dataMTrig_Solenoid_RewCalib_nCycle__R.vi"() -> ("output_Solenoid_RewCalib_nCycle__R"=w130:i32)  [unwired: 11 in]
              n37 = call "myRIO_BRig_RT_dataMTrig_Solenoid_Tdelay__L.vi"() -> ("output_Solenoid_Tdelay__L"=w129:i32)  [unwired: 11 in]
              n38 = call "myRIO_BRig_RT_dataMTrig_Solenoid_Tdelay__R.vi"() -> ("output_Solenoid_Tdelay__R"=w128:i32)  [unwired: 11 in]
              n39 = local read "MTrig_Solenoid_Tcycle__L"() -> (w140:u16)
              n40 = local read "MTrig_Solenoid_Tcycle__R"() -> (w141:u16)
              n41 = local read "MTrig_Laser_Tcycle"() -> (w121:u16)
              n42 = call "myRIO_BRig_RT_dataMTrig_init.vi"() -> ("output_dataMTrig"=w134:u16[])  [unwired: 5 in]
              n43 = local write "RewCalib_Trig_R"(w124) -> ()
              n44 = local write "RewCalib_Trig_L"(w124) -> ()
              n45 = local read "Tcycle_Cue_min"() -> (w122:u16)
              n46 = Replace Array Subset(array=w134, new element #1=w140, index #1=w135, new element #2=w141, index #2=w136, new element #3=w122, index #3=w137, new element #4=w122, index #4=w138, new element #5=w121, index #5=w139, new element #6=w120, index #6=w131, new element #7=w120, index #7=w130, new element #8=w120, index #8=w129, new element #9=w120, index #9=w128) -> (w133:u16[])
            }
            frame "UploadSettings_pre" {
              # "When the Host sends settings,\nnot all files send at the same time.\n\nIf RT reads the settings faster\nthan the Host can send them,\nthen we will skip settings.\n\nSolution:\nWait 20 cycles"
              n47 = Increment(x=w154) -> (x+1=w153:u16)
              n48 = Greater?(x=w153, y=u16 20) -> (0:w151:bool)
              n49 = Select(t=myRIO_BRig_RT__Case_NonExp_stateList."UploadSettings_Read_dataExp", s=w151, f=w150) -> (s? t:f=w148:T1)
            }
            frame "UploadSettings_Read_dataExp" {
              # "grab dataExp and\nstore it in the\ngeneric data array"
              # "dataExp"
              n50 = call "myRIO_BRig_RT_dataExp_init_details.vi"() -> ("output_dataSize"=w162:i32, "output_dataName"=w165:string)  [unwired: 10 in]
              n51 = call "myRIO_BRig_RT_comm_webdav_uploadReceived_check.vi"("input_dataName"=w165) -> ("output_Iexist"=w164:bool, "output_dataPath"=w163:path)  [unwired: 9 in]
              n52 = case shown="True" w164 {
                tunnel: w163 -> [_ w177]
                tunnel: w162 -> [_ w176]
                tunnel: [_ w175] -> w161
                tunnel: w158 -> [w170 w174]
                tunnel: [w170 w171] -> w157
                frame False {
                }
                frame True {
                  n53 = call "myRIO_BRig_RT_comm_webdav_uploadReceived_read.vi"("input_dataSize"=w176, "input_filePath"=w177) -> ("output_Ivalid"=w175:bool, "output_data"=w173:i64[])  [unwired: 8 in]
                  n54 = To Unsigned Word Integer(number=w173) -> (unsigned 16bit integer=w172:u16[])
                  n55 = Select(t=w172, s=w175, f=w174) -> (s? t:f=w171:u16[])
                }
              }
              n56 = Select(t=myRIO_BRig_RT__Case_NonExp_stateList."UploadSettings_dataExp_1", s=w161, f=myRIO_BRig_RT__Case_NonExp_stateList."UploadSettings_Read_dataLC" ("t")) -> (s? t:f=w156:T1)
            }
            frame "UploadSettings_Read_dataLC" {
              # "grab dataLC and\nstore it in the\ngeneric data array"
              # "dataLC"
              n57 = call "myRIO_BRig_RT_dataLC_init_details.vi"() -> ("output_dataSize"=w185:i32, "output_dataName"=w188:string)  [unwired: 10 in]
              n58 = call "myRIO_BRig_RT_comm_webdav_uploadReceived_check.vi"("input_dataName"=w188) -> ("output_Iexist"=w187:bool, "output_dataPath"=w186:path)  [unwired: 9 in]
              n59 = case shown="True" w187 {
                tunnel: w186 -> [_ w200]
                tunnel: w185 -> [_ w199]
                tunnel: [_ w198] -> w184
                tunnel: w181 -> [w193 w197]
                tunnel: [w193 w194] -> w180
                frame False {
                }
                frame True {
                  n60 = call "myRIO_BRig_RT_comm_webdav_uploadReceived_read.vi"("input_dataSize"=w199, "input_filePath"=w200) -> ("output_Ivalid"=w198:bool, "output_data"=w196:i64[])  [unwired: 8 in]
                  n61 = To Unsigned Word Integer(number=w196) -> (unsigned 16bit integer=w195:u16[])
                  n62 = Select(t=w195, s=w198, f=w197) -> (s? t:f=w194:u16[])
                }
              }
              n63 = Select(t=myRIO_BRig_RT__Case_NonExp_stateList."UploadSettings_dataLC_1", s=w184, f=myRIO_BRig_RT__Case_NonExp_stateList."UploadSettings_Read_dataMTrig" ("t")) -> (s? t:f=w179:T1)
            }
            frame "UploadSettings_Read_dataMTrig" {
              # "grab dataMTrig and\nstore it in the\ngeneric data array"
              # "dataMTrig"
              n64 = call "myRIO_BRig_RT_dataMTrig_init_details.vi"() -> ("output_dataSize"=w208:i32, "output_dataName"=w211:string)  [unwired: 10 in]
              n65 = call "myRIO_BRig_RT_comm_webdav_uploadReceived_check.vi"("input_dataName"=w211) -> ("output_Iexist"=w210:bool, "output_dataPath"=w209:path)  [unwired: 9 in]
              n66 = case shown="True" w210 {
                tunnel: w209 -> [_ w223]
                tunnel: w208 -> [_ w222]
                tunnel: [_ w221] -> w207
                tunnel: w204 -> [w216 w220]
                tunnel: [w216 w217] -> w203
                frame False {
                }
                frame True {
                  n67 = call "myRIO_BRig_RT_comm_webdav_uploadReceived_read.vi"("input_dataSize"=w222, "input_filePath"=w223) -> ("output_Ivalid"=w221:bool, "output_data"=w219:i64[])  [unwired: 8 in]
                  n68 = To Unsigned Word Integer(number=w219) -> (unsigned 16bit integer=w218:u16[])
                  n69 = Select(t=w218, s=w221, f=w220) -> (s? t:f=w217:u16[])
                }
              }
              n70 = Select(t=myRIO_BRig_RT__Case_NonExp_stateList."UploadSettings_dataMTrig_1", s=w207, f=myRIO_BRig_RT__Case_NonExp_stateList."Idle" ("t")) -> (s? t:f=w202:T1)
            }
            frame "UploadSettings_dataExp_1" {
              w233 = 100.0 ("y")
              # "Freq"
              # "f_millisec2count"
              # "laser"
              # "Cue_max"
              # "Cue_min"
              # "CuePenalty"
              # "Timeout"
              # "Wrong"
              # "Selection"
              # "RewardPost"
              # "Reward_R"
              # "Reward_L"
              # "Tcycle"
              # "TPB_min_R"
              # "TPB_min_L"
              # "TPB_max_R"
              # "TPB_max_L"
              # "I_trialUntilReward"
              # "ENL_penalty"
              # "ENL_min"
              # "ENL_max"
              # "BUR_max"
              # "BUR_min"
              # "CueCycles"
              # "Audio_Freq_R"
              # "Audio_Freq_L"
              # "Audio_Amp_R"
              # "Audio_Amp_L"
              n71 = call "myRIO_BRig_RT_dataExp_laser_f_millisec2count.vi"() -> ("output_laser_f_millisec2count"=w247:i32)  [unwired: 11 in]
              n72 = call "myRIO_BRig_RT_dataExp_laser_Freq.vi"() -> ("output_laser_Freq"=w246:i32)  [unwired: 11 in]
              n73 = call "myRIO_BRig_RT_dataExp_CueCycles.vi"() -> ("output_CueCycles"=w293:i32)  [unwired: 11 in]
              n74 = call "myRIO_BRig_RT_dataExp_Audio_amp__R.vi"() -> ("output_Audio_amp__R"=w297:i32)  [unwired: 11 in]
              n75 = call "myRIO_BRig_RT_dataExp_Audio_amp__L.vi"() -> ("output_Audio_amp__L"=w299:i32)  [unwired: 11 in]
              n76 = call "myRIO_BRig_RT_dataExp_Tcycle_Reward__L.vi"() -> ("output_Tcycle_Reward__L"=w270:i32)  [unwired: 11 in]
              n77 = call "myRIO_BRig_RT_dataExp_Tcycle_Reward__R.vi"() -> ("output_Tcycle_Reward__R"=w269:i32)  [unwired: 11 in]
              n78 = call "myRIO_BRig_RT_dataExp_Tcycle_RewardPost.vi"() -> ("output_Tcycle_RewardPost"=w268:i32)  [unwired: 11 in]
              n79 = call "myRIO_BRig_RT_dataExp_BUR_min.vi"() -> ("output_BUR_min"=w290:i32)  [unwired: 11 in]
              n80 = call "myRIO_BRig_RT_dataExp_ENL_min.vi"() -> ("output_ENL_min"=w286:i32)  [unwired: 11 in]
              n81 = call "myRIO_BRig_RT_dataExp_TPB_max__L.vi"() -> ("output_TPB_max__L"=w278:i32)  [unwired: 11 in]
              n82 = call "myRIO_BRig_RT_dataExp_TPB_max__R.vi"() -> ("output_TPB_max__R"=w277:i32)  [unwired: 11 in]
              n83 = call "myRIO_BRig_RT_dataExp_ENL_penalty.vi"() -> ("output_ENL_penalty"=w285:i32)  [unwired: 11 in]
              n84 = call "myRIO_BRig_RT_dataExp_laser_Power_min.vi"() -> ("output_laser_Power_min"=w245:i32)  [unwired: 11 in]
              n85 = call "myRIO_BRig_RT_dataExp_laser_Tpeak.vi"() -> ("output_laser_Tpeak"=w244:i32)  [unwired: 11 in]
              n86 = call "myRIO_BRig_RT_dataExp_Audio_freq__L.vi"() -> ("output_Audio_freq__L"=w295:i32)  [unwired: 11 in]
              n87 = call "myRIO_BRig_RT_dataExp_Audio_freq__R.vi"() -> ("output_Audio_freq__R"=w294:i32)  [unwired: 11 in]
              n88 = call "myRIO_BRig_RT_dataExp_BUR_max.vi"() -> ("output_BUR_max"=w291:i32)  [unwired: 11 in]
              n89 = call "myRIO_BRig_RT_dataExp_ENL_max.vi"() -> ("output_ENL_max"=w287:i32)  [unwired: 11 in]
              n90 = call "myRIO_BRig_RT_dataExp_ItrialUntilReward.vi"() -> ("output_I_trialUntilReward"=w281:i32)  [unwired: 11 in]
              n91 = call "myRIO_BRig_RT_dataExp_Tcycle_Selection.vi"() -> ("output_Tcycle_Selection"=w267:i32)  [unwired: 11 in]
              n92 = call "myRIO_BRig_RT_dataExp_Tcycle_Wrong.vi"() -> ("output_Tcycle_Wrong"=w266:i32)  [unwired: 11 in]
              n93 = call "myRIO_BRig_RT_dataExp_Tcycle_Timeout.vi"() -> ("output_Tcycle_Timeout"=w265:i32)  [unwired: 11 in]
              n94 = call "myRIO_BRig_RT_dataExp_TPB_min__L.vi"() -> ("output_TPB_min__L"=w276:i32)  [unwired: 11 in]
              n95 = call "myRIO_BRig_RT_dataExp_TPB_min__R.vi"() -> ("output_TPB_min__R"=w275:i32)  [unwired: 11 in]
              n96 = call "myRIO_BRig_RT_dataExp_laser_Tshutter.vi"() -> ("output_laser_Tshutter"=w243:i32)  [unwired: 11 in]
              n97 = call "myRIO_BRig_RT_dataExp_laser_duration.vi"() -> ("output_laser_duration"=w242:i32)  [unwired: 11 in]
              n98 = call "myRIO_BRig_RT_dataExp_Tcycle_CuePenalty.vi"() -> ("output_Tcycle_CuePenalty"=w258:i32)  [unwired: 11 in]
              n99 = call "myRIO_BRig_RT_dataExp_Tcycle_Cue_min.vi"() -> ("output_Tcycle_Cue_min"=w257:i32)  [unwired: 11 in]
              n100 = call "myRIO_BRig_RT_dataExp_Tcycle_Cue_max.vi"() -> ("output_Tcycle_Cue_max"=w256:i32)  [unwired: 11 in]
              n101 = Index Array(array=w250, index #1=w299, index #2=w297, index #3=w295, index #4=w294, index #5=w293, index #6=w291, index #7=w290, index #8=w287, index #9=w286, index #10=w285, index #11=w281, index #12=w278, index #13=w277, index #14=w276, index #15=w275, index #16=w270, index #17=w269, index #18=w268, index #19=w267, index #20=w266, index #21=w265, index #22=w258, index #23=w257, index #24=w256, index #25=w247, index #26=w246, index #27=w245, index #28=w244, index #29=w243, index #30=w242) -> (element #1=w298:u16, element #2=w296:u16, element #3=w253:u16, element #4=w252:u16, element #5=w292:u16, element #6=w289:u16, element #7=w288:u16, element #8=w284:u16, element #9=w283:u16, element #10=w282:u16, element #11=w279:u16, element #12=w274:u16, element #13=w273:u16, element #14=w272:u16, element #15=w271:u16, element #16=w264:u16, element #17=w263:u16, element #18=w262:u16, element #19=w261:u16, element #20=w260:u16, element #21=w259:u16, element #22=w255:u16, element #23=w249:u16, element #24=w248:u16, element #25=w241:u16, element #26=w232:u16, element #27=w231:u16, element #28=w230:u16, element #29=w229:u16, element #30=w225:u16)
              n102 = To Double Precision Float(number=w241) -> (double precision float=w240:dbl)
              n103 = To Double Precision Float(number=w232) -> (double precision float=w238:dbl)
              n104 = To Double Precision Float(number=w231) -> (double precision float=w236:dbl)
              n105 = To Double Precision Float(number=w230) -> (double precision float=w235:dbl)
              n106 = To Double Precision Float(number=w229) -> (double precision float=w234:dbl)
              n107 = local write "Tcycle_Selection"(w261) -> ()
              n108 = local write "Tcycle_Wrong"(w260) -> ()
              n109 = local write "Tcycle_Timeout"(w259) -> ()
              n110 = local write "Audio_Amp__L"(w298) -> ()
              n111 = local write "Audio_Amp__R"(w296) -> ()
              n112 = Divide(x=w240, y=w233) -> (x/y=w239:dbl)
              n113 = Divide(x=w238, y=w233) -> (x/y=w237:dbl)
              n114 = Divide(x=w236, y=w233) -> (x/y=w228:dbl)
              n115 = Divide(x=w235, y=w233) -> (x/y=w227:dbl)
              n116 = Divide(x=w234, y=w233) -> (x/y=w226:dbl)
              n117 = local write "Tcycle_ENLPenalty"(w282) -> ()
              n118 = local write "Tcycle_ENL_max"(w284) -> ()
              n119 = local write "laser_duration"(w225) -> ()
              n120 = local write "TpB_Min_L"(w272) -> ()
              n121 = local write "TpB_Min_R"(w271) -> ()
              n122 = local write "laser_power_min"(w228) -> ()
              n123 = local write "f_millisec2count"(w239) -> ()
              n124 = local write "laser_Tshutter"(w226) -> ()
              n125 = local write "laser_Tpeak"(w227) -> ()
              n126 = local write "laser_Freq"(w237) -> ()
              n127 = local write "Tcycle_CuePenalty"(w255) -> ()
              n128 = local write "Tcycle_Cue_min"(w249) -> ()
              n129 = local write "Tcycle_Cue_max"(w248) -> ()
              n130 = To Unsigned Byte Integer(number=w253) -> (unsigned 8bit integer=w254:u8)
              n131 = To Unsigned Byte Integer(number=w252) -> (unsigned 8bit integer=w251:u8)
              n132 = Not Equal To 0?(x=w279) -> (x != 0?=w280:bool)
              n133 = local write "Tcycle_Reward_L"(w264) -> ()
              n134 = local write "Tcycle_Reward_R"(w263) -> ()
              n135 = local write "Tcycle_RewardPost"(w262) -> ()
              n136 = local write "CueCycles"(w292) -> ()
              n137 = local write "BUR_min"(w288) -> ()
              n138 = local write "BUR_max"(w289) -> ()
              n139 = local write "Tcycle_ENL_min"(w283) -> ()
              n140 = local write "TpB_Max_L"(w274) -> ()
              n141 = local write "TpB_Max_R"(w273) -> ()
              n142 = local write "TrialUntilReward"(w280) -> ()
              n143 = local write "Audio_Freq__L"(w254) -> ()
              n144 = local write "Audio_Freq__R"(w251) -> ()
            }
            frame "UploadSettings_dataLC_1" {
              # "Cue1_All_delayOpt"
              # "ENL1_All_delayOpt"
              # "Cue1_First_delayOpt"
              # "ENL1_First_delayOpt"
              # "ENL1 First"
              # "Cue1 All"
              # "Cue1 First"
              # "Count"
              # "Tdelay"
              # "Prob"
              # "OnOff"
              # "Block"
              # "ENL1 All"
              # "Count"
              # "Tdelay"
              # "Prob"
              # "OnOff"
              # "Block"
              # "Count"
              # "Tdelay"
              # "Prob"
              # "Block"
              # "OnOff"
              # "Count"
              # "Tdelay"
              # "Prob"
              # "OnOff"
              # "Block"
              n145 = call "myRIO_BRig_RT_dataLC_Cue1_First_Block.vi"() -> ("output_Cue1_First_Block"=w362:i32)  [unwired: 11 in]
              n146 = call "myRIO_BRig_RT_dataLC_Cue1_First_OnOff.vi"() -> ("output_Cue1_First_OnOff"=w360:i32)  [unwired: 11 in]
              n147 = call "myRIO_BRig_RT_dataLC_Cue1_First_Count.vi"() -> ("output_Cue1_First_Count"=w357:i32)  [unwired: 11 in]
              n148 = call "myRIO_BRig_RT_dataLC_Cue1_All_Block.vi"() -> ("output_Cue1_All_Block"=w344:i32)  [unwired: 11 in]
              n149 = call "myRIO_BRig_RT_dataLC_Cue1_All_OnOff.vi"() -> ("output_Cue1_All_OnOff"=w343:i32)  [unwired: 11 in]
              n150 = call "myRIO_BRig_RT_dataLC_Cue1_All_Count.vi"() -> ("output_Cue1_All_Count"=w354:i32)  [unwired: 11 in]
              n151 = call "myRIO_BRig_RT_dataLC_ENL1_First_Block.vi"() -> ("output_ENL1_First_Block"=w342:i32)  [unwired: 11 in]
              n152 = call "myRIO_BRig_RT_dataLC_ENL1_First_OnOff.vi"() -> ("output_ENL1_First_OnOff"=w353:i32)  [unwired: 11 in]
              n153 = call "myRIO_BRig_RT_dataLC_ENL1_First_Count.vi"() -> ("output_ENL1_First_Count"=w350:i32)  [unwired: 11 in]
              n154 = call "myRIO_BRig_RT_dataLC_ENL1_All_Block.vi"() -> ("output_ENL1_All_Block"=w349:i32)  [unwired: 11 in]
              n155 = call "myRIO_BRig_RT_dataLC_ENL1_All_OnOff.vi"() -> ("output_ENL1_All_OnOff"=w348:i32)  [unwired: 11 in]
              n156 = call "myRIO_BRig_RT_dataLC_ENL1_All_Count.vi"() -> ("output_ENL1_All_Count"=w345:i32)  [unwired: 11 in]
              n157 = call "myRIO_BRig_RT_dataLC_ENL1_First_delayOpt.vi"() -> ("output_ENL1_First_delayOpt"=w319:i32)  [unwired: 11 in]
              n158 = call "myRIO_BRig_RT_dataLC_Cue1_First_delayOpt.vi"() -> ("output_Cue1_First_delayOpt"=w318:i32)  [unwired: 11 in]
              n159 = call "myRIO_BRig_RT_dataLC_ENL1_All_delayOpt.vi"() -> ("output_ENL1_All_delayOpt"=w311:i32)  [unwired: 11 in]
              n160 = call "myRIO_BRig_RT_dataLC_Cue1_All_delayOpt.vi"() -> ("output_Cue1_All_delayOpt"=w310:i32)  [unwired: 11 in]
              n161 = call "myRIO_BRig_RT_dataLC_Cue1_First_Probability.vi"() -> ("output_Cue1_First_Probability"=w359:i32)  [unwired: 11 in]
              n162 = call "myRIO_BRig_RT_dataLC_Cue1_First_Tdelay.vi"() -> ("output_Cue1_First_Tdelay"=w358:i32)  [unwired: 11 in]
              n163 = call "myRIO_BRig_RT_dataLC_Cue1_All_Probability.vi"() -> ("output_Cue1_All_Probability"=w356:i32)  [unwired: 11 in]
              n164 = call "myRIO_BRig_RT_dataLC_Cue1_All_Tdelay.vi"() -> ("output_Cue1_All_Tdelay"=w355:i32)  [unwired: 11 in]
              n165 = call "myRIO_BRig_RT_dataLC_ENL1_First_Probability.vi"() -> ("output_ENL1_First_Probability"=w352:i32)  [unwired: 11 in]
              n166 = call "myRIO_BRig_RT_dataLC_ENL1_First_Tdelay.vi"() -> ("output_ENL1_First_Tdelay"=w351:i32)  [unwired: 11 in]
              n167 = call "myRIO_BRig_RT_dataLC_ENL1_All_Probability.vi"() -> ("output_ENL1_All_Probability"=w347:i32)  [unwired: 11 in]
              n168 = call "myRIO_BRig_RT_dataLC_ENL1_All_Tdelay.vi"() -> ("output_ENL1_All_Tdelay"=w346:i32)  [unwired: 11 in]
              n169 = Index Array(array=w320, index #1=w362, index #2=w360, index #3=w359, index #4=w358, index #5=w357, index #6=w344, index #7=w343, index #8=w356, index #9=w355, index #10=w354, index #11=w342, index #12=w353, index #13=w352, index #14=w351, index #15=w350, index #16=w349, index #17=w348, index #18=w347, index #19=w346, index #20=w345, index #21=w319, index #22=w318, index #23=w311, index #24=w310) -> (element #1=w361:u16, element #2=w340:u16, element #3=w339:u16, element #4=w338:u16, element #5=w337:u16, element #6=w333:u16, element #7=w332:u16, element #8=w331:u16, element #9=w330:u16, element #10=w329:u16, element #11=w328:u16, element #12=w327:u16, element #13=w326:u16, element #14=w325:u16, element #15=w312:u16, element #16=w324:u16, element #17=w323:u16, element #18=w322:u16, element #19=w321:u16, element #20=w313:u16, element #21=w316:u16, element #22=w314:u16, element #23=w307:u16, element #24=w306:u16)
              n170 = Not Equal To 0?(x=w307) -> (x != 0?=w309:bool)
              n171 = Not Equal To 0?(x=w306) -> (x != 0?=w308:bool)
              n172 = Not Equal To 0?(x=w316) -> (x != 0?=w317:bool)
              n173 = Not Equal To 0?(x=w314) -> (x != 0?=w315:bool)
              n174 = Not Equal To 0?(x=w340) -> (x != 0?=w341:bool)
              n175 = Not Equal To 0?(x=w332) -> (x != 0?=w336:bool)
              n176 = Not Equal To 0?(x=w327) -> (x != 0?=w335:bool)
              n177 = Not Equal To 0?(x=w323) -> (x != 0?=w334:bool)
              n178 = local write "LC_Cue1_First_Probability"(w339) -> ()
              n179 = local write "LC_ENL1_First_Probability"(w326) -> ()
              n180 = local write "LC_ENL1_First_delayOpt"(w317) -> ()
              n181 = local write "LC_Cue1_First_delayOpt"(w315) -> ()
              n182 = local write "LC_ENL1_All_delayOpt"(w309) -> ()
              n183 = local write "LC_Cue1_All_delayOpt"(w308) -> ()
              n184 = local write "LC_Cue1_All_Probability"(w331) -> ()
              n185 = local write "LC_Cue1_First_Tdelay"(w338) -> ()
              n186 = local write "LC_ENL1_All_Probability"(w322) -> ()
              n187 = local write "LC_Cue1_First_OnOff"(w341) -> ()
              n188 = local write "LC_Cue1_First_Count"(w337) -> ()
              n189 = local write "LC_Cue1_First_Block"(w361) -> ()
              n190 = local write "LC_ENL1_First_Tdelay"(w325) -> ()
              n191 = local write "LC_ENL1_First_OnOff"(w335) -> ()
              n192 = local write "LC_ENL1_First_Count"(w312) -> ()
              n193 = local write "LC_ENL1_First_Block"(w328) -> ()
              n194 = local write "LC_Cue1_All_Tdelay"(w330) -> ()
              n195 = local write "LC_Cue1_All_OnOff"(w336) -> ()
              n196 = local write "LC_Cue1_All_Count"(w329) -> ()
              n197 = local write "LC_Cue1_All_Block"(w333) -> ()
              n198 = local write "LC_ENL1_All_Tdelay"(w321) -> ()
              n199 = local write "LC_ENL1_All_OnOff"(w334) -> ()
              n200 = local write "LC_ENL1_All_Count"(w313) -> ()
              n201 = local write "LC_ENL1_All_Block"(w324) -> ()
            }
            frame "UploadSettings_dataLC_2" {
              # "Wrong"
              # "Reward"
              # "Trial"
              # "Tdelay"
              # "Prob"
              # "Block"
              # "OnOff"
              # "Trial"
              # "Tdelay"
              # "Prob"
              # "OnOff"
              # "Block"
              n202 = call "myRIO_BRig_RT_dataLC_Reward_Block.vi"() -> ("output_Reward_Block"=w394:i32)  [unwired: 11 in]
              n203 = call "myRIO_BRig_RT_dataLC_Reward_OnOff.vi"() -> ("output_Reward_OnOff"=w392:i32)  [unwired: 11 in]
              n204 = call "myRIO_BRig_RT_dataLC_Reward_Trial.vi"() -> ("output_Reward_Trial"=w389:i32)  [unwired: 11 in]
              n205 = call "myRIO_BRig_RT_dataLC_Wrong_Block.vi"() -> ("output_Wrong_Block"=w385:i32)  [unwired: 11 in]
              n206 = call "myRIO_BRig_RT_dataLC_Wrong_OnOff.vi"() -> ("output_Wrong_OnOff"=w384:i32)  [unwired: 11 in]
              n207 = call "myRIO_BRig_RT_dataLC_Wrong_Trial.vi"() -> ("output_Wrong_Trial"=w386:i32)  [unwired: 11 in]
              n208 = call "myRIO_BRig_RT_dataLC_Reward_Probability.vi"() -> ("output_Reward_Probability"=w391:i32)  [unwired: 11 in]
              n209 = call "myRIO_BRig_RT_dataLC_Reward_Tdelay.vi"() -> ("output_Reward_Tdelay"=w390:i32)  [unwired: 11 in]
              n210 = call "myRIO_BRig_RT_dataLC_Wrong_Probability.vi"() -> ("output_Wrong_Probability"=w388:i32)  [unwired: 11 in]
              n211 = call "myRIO_BRig_RT_dataLC_Wrong_Tdelay.vi"() -> ("output_Wrong_Tdelay"=w387:i32)  [unwired: 11 in]
              n212 = Index Array(array=w369, index #1=w394, index #2=w392, index #3=w391, index #4=w390, index #5=w389, index #6=w385, index #7=w384, index #8=w388, index #9=w387, index #10=w386) -> (element #1=w393:u16, element #2=w382:u16, element #3=w381:u16, element #4=w380:u16, element #5=w379:u16, element #6=w377:u16, element #7=w376:u16, element #8=w375:u16, element #9=w374:u16, element #10=w373:u16)
              n213 = Not Equal To 0?(x=w382) -> (x != 0?=w383:bool)
              n214 = Not Equal To 0?(x=w376) -> (x != 0?=w378:bool)
              n215 = local write "LC_Reward_Probability"(w381) -> ()
              n216 = local write "LC_Wrong_Probability"(w375) -> ()
              n217 = local write "LC_Reward_Tdelay"(w380) -> ()
              n218 = local write "LC_Reward_OnOff"(w383) -> ()
              n219 = local write "LC_Reward_Block"(w393) -> ()
              n220 = local write "LC_Reward_Trial"(w379) -> ()
              n221 = local write "LC_Wrong_Tdelay"(w374) -> ()
              n222 = local write "LC_Wrong_OnOff"(w378) -> ()
              n223 = local write "LC_Wrong_Block"(w377) -> ()
              n224 = local write "LC_Wrong_Trial"(w373) -> ()
            }
            frame "UploadSettings_dataMTrig_1" {
              # "Tdelay_R"
              # "Tdelay_L"
              # "Tcycle_R"
              # "Tcycle_L"
              # "RewCalib_nCycle_R"
              # "RewCalib_nCycle_L"
              # "Solenoid"
              # "Laser_Tcycle"
              n225 = call "myRIO_BRig_RT_dataMTrig_Laser_Tcycle.vi"() -> ("output_Laser_Tcycle"=w405:i32)  [unwired: 11 in]
              n226 = call "myRIO_BRig_RT_dataMTrig_Solenoid_RewCalib_nCycle__L.vi"() -> ("output_Solenoid_RewCalib_nCycle__L"=w404:i32)  [unwired: 11 in]
              n227 = call "myRIO_BRig_RT_dataMTrig_Solenoid_RewCalib_nCycle__R.vi"() -> ("output_Solenoid_RewCalib_nCycle__R"=w403:i32)  [unwired: 11 in]
              n228 = call "myRIO_BRig_RT_dataMTrig_Solenoid_Tdelay__L.vi"() -> ("output_Solenoid_Tdelay__L"=w400:i32)  [unwired: 11 in]
              n229 = call "myRIO_BRig_RT_dataMTrig_Solenoid_Tdelay__R.vi"() -> ("output_Solenoid_Tdelay__R"=w399:i32)  [unwired: 11 in]
              n230 = call "myRIO_BRig_RT_dataMTrig_Solenoid_Tcycle__L.vi"() -> ("output_Solenoid_Tcycle__L"=w402:i32)  [unwired: 11 in]
              n231 = call "myRIO_BRig_RT_dataMTrig_Solenoid_Tcycle__R.vi"() -> ("output_Solenoid_Tcycle__R"=w401:i32)  [unwired: 11 in]
              n232 = Index Array(array=w398, index #1=w405, index #2=w404, index #3=w403, index #4=w402, index #5=w401, index #6=w400, index #7=w399) -> (element #1=w412:u16, element #2=w411:u16, element #3=w410:u16, element #4=w409:u16, element #5=w408:u16, element #6=w407:u16, element #7=w406:u16)
              n233 = Replace Array Subset(array=w417, new element #1=w412, index #1=w405, new element #2=w411, index #2=w404, new element #3=w410, index #3=w403, new element #4=w409, index #4=w402, new element #5=w408, index #5=w401, new element #6=w407, index #6=w400, new element #7=w406, index #7=w399) -> (w416:u16[])
              n234 = local write "MTrig_Solenoid_Tcycle__L"(w409) -> ()
              n235 = local write "MTrig_Solenoid_Tcycle__R"(w408) -> ()
              n236 = local write "MTrig_Laser_Tcycle"(w412) -> ()
            }
            frame "Idle" {
              # "To ensure timing, we split the\nidle state into 4 phases"
              # "Laser_Tcycle"
              # "Audio_Tcycle_R"
              # "Audio_Tcycle_L"
              n237 = local read "f_millisec2count"() -> (w422:dbl)
              n238 = local read "MTrig_Audio_trig__L"() -> (w432:bool)
              n239 = local read "MTrig_Audio_trig__R"() -> (w434:bool)
              n240 = Select(t=myRIO_BRig_RT__Case_NonExp_stateList."SendData" ("Enum"), s="SendData", f=myRIO_BRig_RT__Case_NonExp_stateList."Idle_2" ("Enum")) -> (s? t:f=w427:T1)
              n241 = local read "MTrig_Laser_trig"() -> (w433:bool)
              n242 = call "myRIO_BRig_RT_dataMTrig_Audio_Tcycle__L.vi"() -> ("output_Audio_Tcycle__L"=w445:i32)  [unwired: 11 in]
              n243 = call "myRIO_BRig_RT_dataMTrig_Audio_Tcycle__R.vi"() -> ("output_Audio_Tcycle__R"=w444:i32)  [unwired: 11 in]
              n244 = call "myRIO_BRig_RT_dataMTrig_Laser_Tcycle.vi"() -> ("output_Laser_Tcycle"=w443:i32)  [unwired: 11 in]
              n245 = To Unsigned Word Integer(number=w422) -> (unsigned 16bit integer=w421:u16)
              n246 = local read "MTrig_Laser_Tcycle"() -> (w425:u16)
              n247 = xnode "Read/Write Control"("FPGA VI Reference In"=w420, "error in"=w419, "k1__counter_per_ms"=w421) -> ()  [unwired: 2 out]
              n248 = Select(t=myRIO_BRig_RT__Case_NonExp_stateList."TestConnection" ("Enum"), s="TestConnection", f=w427) -> (s? t:f=w436:T1)
              n249 = local read "Tcycle_Cue_min"() -> (w426:u16)
              n250 = Compound Arithmetic op=OR(w432, w434, w433) -> (w435:bool)
              n251 = case shown="True" w435 {
                frame False {
                }
                frame True {
                  w446 = FALSE
                  n252 = local write "MTrig_Audio_trig__L"(w446) -> ()
                  n253 = local write "MTrig_Audio_trig__R"(w446) -> ()
                  n254 = local write "MTrig_Laser_trig"(w446) -> ()
                }
              }
              n255 = Replace Array Subset(array=w441, new element #1=w426, index #1=w445, new element #2=w426, index #2=w444, new element #3=w425, index #3=w443) -> (w442:u16[])
              n256 = local read "Audio_Amp__R"() -> (w437:u16)
              n257 = local read "Audio_Amp__L"() -> (w438:u16)
              n258 = local read "Audio_Freq__R"() -> (w423:u8)
              n259 = local read "Audio_Freq__L"() -> (w424:u8)
            }
            frame "Idle_2" {
              w448 = u16 0 ("t")
              # "To ensure timing, we split the\nidle state into 4 phases"
              # "Ncycles"
              # "Ncycles"
              # "RewCalib"
              # "RewCalib"
              # "Solenoid R"
              # "Solenoid L"
              n260 = call "myRIO_BRig_RT_dataMTrig_Solenoid_RewCalib_OnOff__L.vi"() -> ("output_Solenoid_RewCalib_OnOff__L"=w483:i32)  [unwired: 11 in]
              n261 = call "myRIO_BRig_RT_dataMTrig_Solenoid_N__L.vi"() -> ("output_Solenoid_N__L"=w471:i32)  [unwired: 11 in]
              n262 = call "myRIO_BRig_RT_dataMTrig_Solenoid_RewCalib_OnOff__R.vi"() -> ("output_Solenoid_RewCalib_OnOff__R"=w468:i32)  [unwired: 11 in]
              n263 = call "myRIO_BRig_RT_dataMTrig_Solenoid_N__R.vi"() -> ("output_Solenoid_N__R"=w467:i32)  [unwired: 11 in]
              n264 = Index Array(array=w474, index #1=w483, index #2=w471, index #3=w468, index #4=w467) -> (element #1=w470:u16, element #2=w465:u16, element #3=w466:u16, element #4=w464:u16)
              n265 = local read "RewCalib_Trig_L"() -> (w463:bool)
              n266 = local read "RewCalib_Trig_R"() -> (w462:bool)
              n267 = Equal To 0?(x=w465) -> (x = 0?=w473:bool)
              n268 = Equal To 0?(x=w464) -> (x = 0?=w472:bool)
              n269 = Not Equal To 0?(x=w466) -> (x != 0?=w484:bool)
              n270 = Not Equal To 0?(x=w470) -> (x != 0?=w485:bool)
              n271 = And(x=w473, y=w472) -> (x .and. y?=w477:bool)
              n272 = Or(x=w463, y=w462) -> (x .or. y?=w478:bool)
              n273 = Not Exclusive Or(1:w485, 2:w463) -> (0:w480:bool)
              n274 = Not Exclusive Or(1:w484, 2:w462) -> (0:w482:bool)
              n275 = And(x=w478, y=w477) -> (x .and. y?=w460:bool)
              n276 = Not(x=w480) -> (.not. x?=w479:bool)
              n277 = Not(x=w482) -> (.not. x?=w481:bool)
              n278 = Or(x=w479, y=w481) -> (x .or. y?=w461:bool)
              n279 = Or(x=w460, y=w461) -> (x .or. y?=w476:bool)
              n280 = local read "count_warmup_R"() -> (w447:u16)
              n281 = local read "count_warmup_L"() -> (w452:u16)
              n282 = Select(t=myRIO_BRig_RT__Case_NonExp_stateList."RewardCalibration_pre" ("Enum"), s=w476, f=myRIO_BRig_RT__Case_NonExp_stateList."Idle_3" ("Enum")) -> (s? t:f=w459:T1)
              n283 = Select(t=w448, s="count_warmup_L_reset", f=w452) -> (s? t:f=→"count_warmup_L":u16)
              n284 = Select(t=w448, s="count_warmup_R_reset", f=w447) -> (s? t:f=→"count_warmup_R":u16)
            }
            frame "Idle_3" {
              w512 = u8 0 ("f")
              # "To ensure timing, we split the\nidle state into 4 phases"
              n285 = local read "MTrig_Solenoid_trig__L"() -> (w500:bool)
              n286 = local read "MTrig_Solenoid_trig__R"() -> (w513:bool)
              n287 = local read "warmupType"() -> (w491:u8)
              n288 = local read "warmup"() -> (w505:bool)
              n289 = Not Equal To 0?(x=w491) -> (x != 0?=w490:bool)
              n290 = Not(x=w490) -> (.not. x?=w506:bool)
              n291 = Select(t=u8 1, s=w500, f=w512) -> (s? t:f=w511:u8)
              n292 = Select(t=u8 2, s=w513, f=w512) -> (s? t:f=w510:u8)
              n293 = And(x=w505, y=w506) -> (x .and. y?=w504:bool)
              n294 = And(x=w505, y=w490) -> (x .and. y?=w496:bool)
              n295 = Add(x=w511, y=w510) -> (x+y=w509:u8)
              n296 = case shown="3" w509 {
                tunnel: w508 -> [w516 w520 w538 w556]
                tunnel: [w516 w519 w537 w555] -> w507
                tunnel: w504 -> [_ w518 w536 w554]
                tunnel: [_ TRUE TRUE TRUE] -> w498
                frame 0, Default {
                }
                frame 1 {
                  n297 = case shown="True" w518 {
                    tunnel: w520 -> [w529 w534]
                    tunnel: [w528 w533] -> w519
                    frame True {
                      # "Audio_L"
                      # "Solenoid_L"
                      n298 = call "myRIO_BRig_RT_dataMTrig_Solenoid_N__L.vi"() -> ("output_Solenoid_N__L"=w525:i32)  [unwired: 11 in]
                      n299 = call "myRIO_BRig_RT_dataMTrig_Audio_N__L.vi"() -> ("output_Audio_N__L"=w523:i32)  [unwired: 11 in]
                      n300 = Index Array(array=w529, index #1=w525, index #2=w523) -> (element #1=w527:u16, element #2=w526:u16)
                      n301 = Increment(x=w527) -> (x+1=w524:u16)
                      n302 = Increment(x=w526) -> (x+1=w522:u16)
                      n303 = Replace Array Subset(array=w529, new element #1=w524, index #1=w525, new element #2=w522, index #2=w523) -> (w528:u16[])
                    }
                    frame False {
                      # "Solenoid_L"
                      n304 = call "myRIO_BRig_RT_dataMTrig_Solenoid_N__L.vi"() -> ("output_Solenoid_N__L"=w531:i32)  [unwired: 11 in]
                      n305 = Index Array(array=w534, index=w531) -> (element=w532:u16)
                      n306 = Increment(x=w532) -> (x+1=w530:u16)
                      n307 = Replace Array Subset(array=w534, new element=w530, index=w531) -> (w533:u16[])
                    }
                  }
                  n308 = local write "MTrig_Solenoid_trig__L"(FALSE) -> ()
                }
                frame 2 {
                  n309 = case shown="True" w536 {
                    tunnel: w538 -> [w547 w552]
                    tunnel: [w546 w551] -> w537
                    frame True {
                      # "Audio_R"
                      # "Solenoid_R"
                      n310 = call "myRIO_BRig_RT_dataMTrig_Solenoid_N__R.vi"() -> ("output_Solenoid_N__R"=w543:i32)  [unwired: 11 in]
                      n311 = call "myRIO_BRig_RT_dataMTrig_Audio_N__R.vi"() -> ("output_Audio_N__R"=w542:i32)  [unwired: 11 in]
                      n312 = Index Array(array=w547, index #1=w543, index #2=w542) -> (element #1=w545:u16, element #2=w544:u16)
                      n313 = Increment(x=w544) -> (x+1=w540:u16)
                      n314 = Increment(x=w545) -> (x+1=w541:u16)
                      n315 = Replace Array Subset(array=w547, new element #1=w541, index #1=w543, new element #2=w540, index #2=w542) -> (w546:u16[])
                    }
                    frame False {
                      # "Solenoid_R"
                      n316 = call "myRIO_BRig_RT_dataMTrig_Solenoid_N__R.vi"() -> ("output_Solenoid_N__R"=w548:i32)  [unwired: 11 in]
                      n317 = Index Array(array=w552, index=w548) -> (element=w550:u16)
                      n318 = Increment(x=w550) -> (x+1=w549:u16)
                      n319 = Replace Array Subset(array=w552, new element=w549, index=w548) -> (w551:u16[])
                    }
                  }
                  n320 = local write "MTrig_Solenoid_trig__R"(FALSE) -> ()
                }
                frame 3 {
                  w557 = FALSE
                  n321 = case shown="True" w554 {
                    tunnel: w556 -> [w571 w579]
                    tunnel: [w570 w578] -> w555
                    frame True {
                      # "Audio_R"
                      # "Solenoid_R"
                      # "Audio_L"
                      # "Solenoid_L"
                      n322 = call "myRIO_BRig_RT_dataMTrig_Solenoid_N__L.vi"() -> ("output_Solenoid_N__L"=w565:i32)  [unwired: 11 in]
                      n323 = call "myRIO_BRig_RT_dataMTrig_Audio_N__L.vi"() -> ("output_Audio_N__L"=w563:i32)  [unwired: 11 in]
                      n324 = call "myRIO_BRig_RT_dataMTrig_Solenoid_N__R.vi"() -> ("output_Solenoid_N__R"=w561:i32)  [unwired: 11 in]
                      n325 = call "myRIO_BRig_RT_dataMTrig_Audio_N__R.vi"() -> ("output_Audio_N__R"=w560:i32)  [unwired: 11 in]
                      n326 = Index Array(array=w571, index #1=w565, index #2=w563, index #3=w561, index #4=w560) -> (element #1=w569:u16, element #2=w568:u16, element #3=w567:u16, element #4=w566:u16)
                      n327 = Increment(x=w566) -> (x+1=w558:u16)
                      n328 = Increment(x=w569) -> (x+1=w564:u16)
                      n329 = Increment(x=w568) -> (x+1=w562:u16)
                      n330 = Increment(x=w567) -> (x+1=w559:u16)
                      n331 = Replace Array Subset(array=w571, new element #1=w564, index #1=w565, new element #2=w562, index #2=w563, new element #3=w559, index #3=w561, new element #4=w558, index #4=w560) -> (w570:u16[])
                    }
                    frame False {
                      # "Solenoid_R"
                      # "Solenoid_L"
                      n332 = call "myRIO_BRig_RT_dataMTrig_Solenoid_N__L.vi"() -> ("output_Solenoid_N__L"=w575:i32)  [unwired: 11 in]
                      n333 = call "myRIO_BRig_RT_dataMTrig_Solenoid_N__R.vi"() -> ("output_Solenoid_N__R"=w572:i32)  [unwired: 11 in]
                      n334 = Index Array(array=w579, index #1=w575, index #2=w572) -> (element #1=w577:u16, element #2=w576:u16)
                      n335 = Increment(x=w577) -> (x+1=w574:u16)
                      n336 = Increment(x=w576) -> (x+1=w573:u16)
                      n337 = Replace Array Subset(array=w579, new element #1=w574, index #1=w575, new element #2=w573, index #2=w572) -> (w578:u16[])
                    }
                  }
                  n338 = local write "MTrig_Solenoid_trig__L"(w557) -> ()
                  n339 = local write "MTrig_Solenoid_trig__R"(w557) -> ()
                }
              }
              n340 = local read "get_countPerMS"() -> (w489:bool)
              n341 = Select(t=myRIO_BRig_RT__Case_NonExp_stateList."Get_FPGA_count_per_ms" ("Enum"), s=w489, f=myRIO_BRig_RT__Case_NonExp_stateList."Idle_4" ("Enum")) -> (s? t:f=w487:T1)
              n342 = Select(t=myRIO_BRig_RT__Case_NonExp_stateList."Cue_pre", s=w496, f=myRIO_BRig_RT__Case_NonExp_stateList."DispenseWater_pre" ("Enum")) -> (s? t:f=w494:T1)
              n343 = Select(t=w494, s=w498, f=w487) -> (s? t:f=w499:T1)
            }
            frame "Idle_4" {
              # "use dataMTrig as it is one of the last to transfer"
              # "To ensure timing, we split the\nidle state into 4 phases"
              n344 = call "myRIO_BRig_RT_comm_webdav_uploadReceived_check_v2,0.vi"("input_dataName"="dataMTrig") -> ("output_Iexist"=w589:bool)  [unwired: 9 in, 1 out]
              n345 = Select(t=myRIO_BRig_RT__Case_NonExp_stateList."UploadSettings_pre" ("Enum"), s=w589, f=myRIO_BRig_RT__Case_NonExp_stateList."Idle") -> (s? t:f=w587:T1)
            }
            frame "Cue_pre" {
              w600 = u16 1 ("t")
              w599 = u16 0 ("new element/subarray")
              w596 = u16 0 ("new element/subarray")
              # "Ncycle"
              # "count"
              # "Audio_R"
              # "Solenoid_R"
              # "Solenoid_L"
              # "Ncycle"
              # "count"
              # "Audio_L"
              n346 = call "myRIO_BRig_RT_dataMTrig_Solenoid_N__L.vi"() -> ("output_Solenoid_N__L"=w609:i32)  [unwired: 11 in]
              n347 = call "myRIO_BRig_RT_dataMTrig_Solenoid_N__R.vi"() -> ("output_Solenoid_N__R"=w608:i32)  [unwired: 11 in]
              n348 = Index Array(array=w605, index #1=w609, index #2=w608) -> (element #1=w607:u16, element #2=w606:u16)
              n349 = Not Equal To 0?(x=w606) -> (x != 0?=w591:bool)
              n350 = Not Equal To 0?(x=w607) -> (x != 0?=w592:bool)
              n351 = Select(t=w600, s=w592, f=w599) -> (s? t:f=w601:u16)
              n352 = Select(t=w600, s=w591, f=w599) -> (s? t:f=w595:u16)
              n353 = call "myRIO_BRig_RT_dataMTrig_Audio_c__L.vi"() -> ("output_Audio_c__L"=w603:i32)  [unwired: 11 in]
              n354 = call "myRIO_BRig_RT_dataMTrig_Audio_N__L.vi"() -> ("output_Audio_N__L"=w602:i32)  [unwired: 11 in]
              n355 = call "myRIO_BRig_RT_dataMTrig_Audio_c__R.vi"() -> ("output_Audio_c__R"=w598:i32)  [unwired: 11 in]
              n356 = call "myRIO_BRig_RT_dataMTrig_Audio_N__R.vi"() -> ("output_Audio_N__R"=w597:i32)  [unwired: 11 in]
              n357 = Replace Array Subset(array=w605, new element #1=w596, index #1=w603, new element #2=w601, index #2=w602, new element #3=w596, index #3=w598, new element #4=w595, index #4=w597) -> (w604:u16[])
            }
            frame "Cue" {
              # "lick did not occur or warmupType==1"
              # "lick occurred?"
              # "Ncycle"
              # "Audio_R"
              # "Ncycle"
              # "Audio_L"
              n358 = local read "warmupType"() -> (w622:u8)
              n359 = Greater?(x=w628, y=w627) -> (0:w631:bool)
              n360 = Greater?(x=w630, y=w629) -> (0:w626:bool)
              n361 = Or(x=w626, y=w631) -> (x .or. y?=w620:bool)
              n362 = Equal?(x=w622, y=u8 1) -> (x = y?=w616:bool)
              n363 = Not(x=w620) -> (.not. x?=w619:bool)
              n364 = call "myRIO_BRig_RT_dataMTrig_Audio_N__L.vi"() -> ("output_Audio_N__L"=w635:i32)  [unwired: 11 in]
              n365 = call "myRIO_BRig_RT_dataMTrig_Audio_N__R.vi"() -> ("output_Audio_N__R"=w634:i32)  [unwired: 11 in]
              n366 = Or(x=w619, y=w616) -> (x .or. y?=w617:bool)
              n367 = case shown="True" w617 {
                tunnel: w635 -> [w644 w662]
                tunnel: w634 -> [w643 w661]
                tunnel: w625 -> [w646 w656]
                tunnel: [w645 w656] -> w624
                tunnel: w623 -> [_ w654]
                tunnel: [myRIO_BRig_RT__Case_NonExp_stateList."Idle" ("t") w653] -> w618
                tunnel: w616 -> [_ w652]
                tunnel: w615 -> [_ w648]
                tunnel: w614 -> [_ w647]
                frame False {
                  w639 = u16 0 ("new element/subarray")
                  # "lick occurred and warmupType==2"
                  n368 = call "myRIO_BRig_RT_dataMTrig_Solenoid_N__R.vi"() -> ("output_Solenoid_N__R"=w640:i32)  [unwired: 11 in]
                  n369 = call "myRIO_BRig_RT_dataMTrig_Solenoid_N__L.vi"() -> ("output_Solenoid_N__L"=w641:i32)  [unwired: 11 in]
                  n370 = Replace Array Subset(array=w646, new element #1=w639, index #1=w644, new element #2=w639, index #2=w643, new element #3=w639, index #3=w641, new element #4=w639, index #4=w640) -> (w645:u16[])
                }
                frame True {
                  n371 = Not(x=w652) -> (.not. x?=w651:bool)
                  n372 = Index Array(array=w656, index #1=w662, index #2=w661) -> (element #1=w660:u16, element #2=w659:u16)
                  n373 = Equal To 0?(x=w660) -> (x = 0?=w658:bool)
                  n374 = Equal To 0?(x=w659) -> (x = 0?=w657:bool)
                  n375 = And(x=w658, y=w657) -> (x .and. y?=w650:bool)
                  n376 = And(x=w650, y=w651) -> (x .and. y?=w649:bool)
                  n377 = case shown="True" w649 {
                    tunnel: w648 -> [_ w670]
                    tunnel: w647 -> [_ w665]
                    frame False {
                    }
                    frame True {
                      n378 = local read "count_warmup_R"() -> (w663:u16)
                      n379 = local read "count_warmup_L"() -> (w668:u16)
                      n380 = Increment(x=w663) -> (x+1=w666:u16)
                      n381 = Increment(x=w668) -> (x+1=w669:u16)
                      n382 = Select(t=w666, s=w665, f=w663) -> (s? t:f=w664:u16)
                      n383 = Select(t=w669, s=w670, f=w668) -> (s? t:f=w667:u16)
                      n384 = local write "count_warmup_R"(w664) -> ()
                      n385 = local write "count_warmup_L"(w667) -> ()
                    }
                  }
                  n386 = Select(t=myRIO_BRig_RT__Case_NonExp_stateList."DispenseWater_pre", s=w650, f=w654) -> (s? t:f=w653:T1)
                }
              }
            }
            frame "RewardCalibration_pre" {
              (unwired) FALSE
              w676 = FALSE
              w687 = u8 0
              w703 = u8 0
              # "Are we starting a RewardCalibration?\nOr are we stopping a RewardCalibration?\nOr is a RewardCalibration over?"
              # "RewCalib\nOnOff"
              # "N"
              # "Solenoid R"
              # "RewCalib\nOnOff"
              # "N"
              # "Solenoid L"
              n387 = local read "RewCalib_Trig_L"() -> (w710:bool)
              n388 = local read "RewCalib_Trig_R"() -> (w679:bool)
              n389 = call "myRIO_BRig_RT_dataMTrig_Solenoid_N__R.vi"() -> ("output_Solenoid_N__R"=w681:i32)  [unwired: 11 in]
              n390 = call "myRIO_BRig_RT_dataMTrig_Solenoid_RewCalib_OnOff__R.vi"() -> ("output_Solenoid_RewCalib_OnOff__R"=w678:i32)  [unwired: 11 in]
              n391 = call "myRIO_BRig_RT_dataMTrig_Solenoid_N__L.vi"() -> ("output_Solenoid_N__L"=w696:i32)  [unwired: 11 in]
              n392 = call "myRIO_BRig_RT_dataMTrig_Solenoid_RewCalib_OnOff__L.vi"() -> ("output_Solenoid_RewCalib_OnOff__L"=w697:i32)  [unwired: 11 in]
              n393 = Index Array(array=w680, index #1=w681, index #2=w678) -> (element #1=w691:u16, element #2=w686:u16)
              n394 = Index Array(array=w680, index #1=w696, index #2=w697) -> (element #1=w707:u16, element #2=w702:u16)
              n395 = Equal To 0?(x=w691) -> (x = 0?=w692:bool)
              n396 = Not Equal To 0?(x=w686) -> (x != 0?=w689:bool)
              n397 = Equal To 0?(x=w707) -> (x = 0?=w708:bool)
              n398 = Not Equal To 0?(x=w702) -> (x != 0?=w705:bool)
              n399 = local write "MTrig_Solenoid_trig__L"(w676) -> ()
              n400 = local write "MTrig_Solenoid_trig__R"(w676) -> ()
              n401 = Select(t=u8 1, s=w679, f=w687) -> (s? t:f=w683:u8)
              n402 = Select(t=u8 1, s=w710, f=w703) -> (s? t:f=w699:u8)
              n403 = Select(t=u8 2, s=w692, f=w687) -> (s? t:f=w684:u8)
              n404 = Select(t=u8 4, s=w689, f=w687) -> (s? t:f=w685:u8)
              n405 = Select(t=u8 2, s=w708, f=w703) -> (s? t:f=w700:u8)
              n406 = Select(t=u8 4, s=w705, f=w703) -> (s? t:f=w701:u8)
              n407 = Compound Arithmetic op=ADD(w683, w684, w685) -> (w682:u8)
              n408 = Compound Arithmetic op=ADD(w699, w700, w701) -> (w698:u8)
              n409 = case shown="7" w698 {
                tunnel: w680 -> [w740 w745 w747 w752 w757 w759 w762 w767]
                tunnel: [w740 w746 w747 w753 w758 w759 w763 w768] -> w695
                tunnel: w697 -> [_ w743 _ w750 w755 _ w761 w766]
                tunnel: w696 -> [_ w744 _ w751 w756 _ _ _]
                frame 0, Default {
                }
                frame 1 {
                  n410 = Replace Array Subset(array=w745, new element #1=u16 100 ("new element/subarray"), index #1=w744, new element #2=u16 1 ("new element/subarray"), index #2=w743) -> (w746:u16[])
                }
                frame 2 {
                }
                frame 3 {
                  n411 = Replace Array Subset(array=w752, new element #1=u16 100 ("new element/subarray"), index #1=w751, new element #2=u16 1 ("new element/subarray"), index #2=w750) -> (w753:u16[])
                }
                frame 4 {
                  w754 = u16 0 ("new element/subarray")
                  n412 = Replace Array Subset(array=w757, new element #1=w754, index #1=w756, new element #2=w754, index #2=w755) -> (w758:u16[])
                }
                frame 5 {
                }
                frame 6 {
                  n413 = Replace Array Subset(array=w762, new element=u16 0 ("new element/subarray"), index=w761) -> (w763:u16[])
                }
                frame 7 {
                  n414 = local write "RewCalib_Trig_L"(FALSE ("RewCalib_Trig_L")) -> ()
                  n415 = Replace Array Subset(array=w767, new element=u16 0 ("new element/subarray"), index=w766) -> (w768:u16[])
                }
              }
              n416 = case shown="7" w682 {
                tunnel: w695 -> [w711 w716 w718 w723 w728 w730 w733 w738]
                tunnel: [w711 w717 w718 w724 w729 w730 w734 w739] -> w694
                tunnel: w678 -> [_ w714 _ w721 w726 _ w732 w737]
                tunnel: w681 -> [_ w715 _ w722 w727 _ _ _]
                frame 0, Default {
                }
                frame 1 {
                  n417 = Replace Array Subset(array=w716, new element #1=u16 100 ("new element/subarray"), index #1=w715, new element #2=u16 1 ("new element/subarray"), index #2=w714) -> (w717:u16[])
                }
                frame 2 {
                }
                frame 3 {
                  n418 = Replace Array Subset(array=w723, new element #1=u16 100 ("new element/subarray"), index #1=w722, new element #2=u16 1 ("new element/subarray"), index #2=w721) -> (w724:u16[])
                }
                frame 4 {
                  w725 = u16 0 ("new element/subarray")
                  n419 = Replace Array Subset(array=w728, new element #1=w725, index #1=w727, new element #2=w725, index #2=w726) -> (w729:u16[])
                }
                frame 5 {
                }
                frame 6 {
                  n420 = Replace Array Subset(array=w733, new element=u16 0 ("new element/subarray"), index=w732) -> (w734:u16[])
                }
                frame 7 {
                  n421 = local write "RewCalib_Trig_R"(FALSE ("RewCalib_Trig_L")) -> ()
                  n422 = Replace Array Subset(array=w738, new element=u16 0 ("new element/subarray"), index=w737) -> (w739:u16[])
                }
              }
            }
            frame "DispenseWater_pre" {
              w776 = u16 0 ("t")
              w819 = u16 0 ("new element/subarray")
              # "just trust me on this one"
              # "RewCalib\nOnOff"
              # "RewCalib\nOnOff"
              # "nCycle"
              # "Solenoid__R"
              # "Tdelay"
              # "delay"
              # "nCycle"
              # "Solenoid__L"
              # "Tdelay"
              # "delay"
              # "Solenoid__R"
              # "count"
              # "Solenoid_Tcycle_R"
              # "Solenoid_Tcycle_L"
              # "Solenoid__L"
              # "count"
              n423 = call "myRIO_BRig_RT_dataMTrig_Solenoid_RewCalib_OnOff__L.vi"() -> ("output_Solenoid_RewCalib_OnOff__L"=w783:i32)  [unwired: 11 in]
              n424 = call "myRIO_BRig_RT_dataMTrig_Solenoid_N__L.vi"() -> ("output_Solenoid_N__L"=w774:i32)  [unwired: 11 in]
              n425 = call "myRIO_BRig_RT_dataMTrig_Solenoid_delay__L.vi"() -> ("output_Solenoid_delay__L"=w817:i32)  [unwired: 11 in]
              n426 = call "myRIO_BRig_RT_dataMTrig_Solenoid_Tdelay__L.vi"() -> ("output_Solenoid_Tdelay__L"=w816:i32)  [unwired: 11 in]
              n427 = call "myRIO_BRig_RT_dataMTrig_Solenoid_N__R.vi"() -> ("output_Solenoid_N__R"=w772:i32)  [unwired: 11 in]
              n428 = call "myRIO_BRig_RT_dataMTrig_Solenoid_delay__R.vi"() -> ("output_Solenoid_delay__R"=w806:i32)  [unwired: 11 in]
              n429 = call "myRIO_BRig_RT_dataMTrig_Solenoid_Tdelay__R.vi"() -> ("output_Solenoid_Tdelay__R"=w805:i32)  [unwired: 11 in]
              n430 = call "myRIO_BRig_RT_dataMTrig_Solenoid_RewCalib_OnOff__R.vi"() -> ("output_Solenoid_RewCalib_OnOff__R"=w779:i32)  [unwired: 11 in]
              n431 = Index Array(array=w818, index #1=w774, index #2=w817, index #3=w816, index #4=w772, index #5=w806, index #6=w805, index #7=w783, index #8=w779) -> (element #1=w775:u16, element #2=w815:u16, element #3=w810:u16, element #4=w778:u16, element #5=w800:u16, element #6=w799:u16, element #7=w784:u16, element #8=w781:u16)
              n432 = Equal To 0?(x=w815) -> (x = 0?=w814:bool)
              n433 = Equal To 0?(x=w800) -> (x = 0?=w804:bool)
              n434 = local read "RewCalib_Trig_L"() -> (w795:bool)
              n435 = local read "RewCalib_Trig_R"() -> (w790:bool)
              n436 = Not Equal To 0?(x=w775) -> (x != 0?=w813:bool)
              n437 = Not Equal To 0?(x=w778) -> (x != 0?=w803:bool)
              n438 = local read "MTrig_Solenoid_Tcycle__L"() -> (w812:u16)
              n439 = local read "MTrig_Solenoid_Tcycle__R"() -> (w798:u16)
              n440 = Not Equal To 0?(x=w784) -> (x != 0?=w794:bool)
              n441 = Not Equal To 0?(x=w781) -> (x != 0?=w792:bool)
              n442 = Not(x=w795) -> (.not. x?=w793:bool)
              n443 = Not(x=w790) -> (.not. x?=w791:bool)
              n444 = And(x=w794, y=w793) -> (x .and. y?=w789:bool)
              n445 = And(x=w792, y=w791) -> (x .and. y?=w788:bool)
              n446 = call "myRIO_BRig_RT_dataMTrig_Solenoid_c__L.vi"() -> ("output_Solenoid_c__L"=w821:i32)  [unwired: 11 in]
              n447 = call "myRIO_BRig_RT_dataMTrig_Solenoid_c__R.vi"() -> ("output_Solenoid_c__R"=w820:i32)  [unwired: 11 in]
              n448 = Select(t=w812, s=w813, f=u16 0) -> (s? t:f=w809:u16)
              n449 = Or(x=w789, y=w788) -> (x .or. y?=w777:bool)
              n450 = Select(t=w798, s=w803, f=u16 0) -> (s? t:f=w801:u16)
              n451 = Select(t=w809, s=w814, f=w810) -> (s? t:f=w807:u16)
              n452 = Select(t=w801, s=w804, f=w799) -> (s? t:f=w796:u16)
              n453 = call "myRIO_BRig_RT_dataMTrig_Solenoid_Tcycle__L.vi"() -> ("output_Solenoid_Tcycle__L"=w808:i32)  [unwired: 11 in]
              n454 = call "myRIO_BRig_RT_dataMTrig_Solenoid_Tcycle__R.vi"() -> ("output_Solenoid_Tcycle__R"=w797:i32)  [unwired: 11 in]
              n455 = Select(t=w776, s=w777, f=w775) -> (s? t:f=w773:u16)
              n456 = Select(t=w776, s=w777, f=w778) -> (s? t:f=w771:u16)
              n457 = Select(t=myRIO_BRig_RT__Case_NonExp_stateList."Idle" ("Enum"), s=w777, f=myRIO_BRig_RT__Case_NonExp_stateList."DispenseWater" ("Enum")) -> (s? t:f=w785:T1)
              n458 = Select(t=w776, s=w777, f=w784) -> (s? t:f=w782:u16)
              n459 = Select(t=w776, s=w777, f=w781) -> (s? t:f=w780:u16)
              n460 = Replace Array Subset(array=w818, new element #1=w819, index #1=w821, new element #2=w819, index #2=w820, new element #3=w807, index #3=w808, new element #4=w796, index #4=w797, new element #5=w782, index #5=w783, new element #6=w780, index #6=w779, new element #7=w773, index #7=w774, new element #8=w771, index #8=w772) -> (w822:u16[])
            }
            frame "DispenseWater" {
              # "D"
              # "C"
              # "B"
              # "A"
              # "(A) Add COUNT and INCREMENT\n(B) Is (A) smaller than Tcycle?\n(C) Are we dispensing water or in the delay phase?\n(D) If (A) is smaller than Tcycle   AND   if we are dispensing water\n      then send TRUE to solenoid"
              # "delay"
              # "Tcycle"
              # "Solenoid__R"
              # "count"
              # "delay"
              # "Tcycle"
              # "Solenoid__L"
              # "count"
              n461 = To Unsigned Word Integer(number=w854) -> (unsigned 16bit integer=w836:u16)
              n462 = call "myRIO_BRig_RT_dataMTrig_Solenoid_delay__R.vi"() -> ("output_Solenoid_delay__R"=w840:i32)  [unwired: 11 in]
              n463 = call "myRIO_BRig_RT_dataMTrig_Solenoid_c__R.vi"() -> ("output_Solenoid_c__R"=w839:i32)  [unwired: 11 in]
              n464 = call "myRIO_BRig_RT_dataMTrig_Solenoid_Tcycle__R.vi"() -> ("output_Solenoid_Tcycle__R"=w841:i32)  [unwired: 11 in]
              n465 = call "myRIO_BRig_RT_dataMTrig_Solenoid_delay__L.vi"() -> ("output_Solenoid_delay__L"=w856:i32)  [unwired: 11 in]
              n466 = call "myRIO_BRig_RT_dataMTrig_Solenoid_c__L.vi"() -> ("output_Solenoid_c__L"=w848:i32)  [unwired: 11 in]
              n467 = call "myRIO_BRig_RT_dataMTrig_Solenoid_Tcycle__L.vi"() -> ("output_Solenoid_Tcycle__L"=w857:i32)  [unwired: 11 in]
              n468 = Index Array(array=w850, index #1=w848, index #2=w857, index #3=w856, index #4=w839, index #5=w841, index #6=w840) -> (element #1=w855:u16, element #2=w845:u16, element #3=w853:u16, element #4=w835:u16, element #5=w832:u16, element #6=w831:u16)
              n469 = Add(x=w855, y=w836) -> (x+y=w846:u16)
              n470 = Add(x=w835, y=w836) -> (x+y=w837:u16)
              n471 = Less?(x=w846, y=w845) -> (x < y?=w829:bool)
              n472 = Equal To 0?(x=w853) -> (x = 0?=w852:bool)
              n473 = Less?(x=w837, y=w832) -> (x < y?=w830:bool)
              n474 = Equal To 0?(x=w831) -> (x = 0?=w838:bool)
              n475 = And(x=w829, y=w852) -> (x .and. y?=w851:bool)
              n476 = Or(x=w829, y=w830) -> (x .or. y?=w828:bool)
              n477 = And(x=w830, y=w838) -> (x .and. y?=w833:bool)
              n478 = Select(t=w846, s=w829, f=w845) -> (s? t:f=w847:u16)
              n479 = Select(t=w837, s=w830, f=w832) -> (s? t:f=w834:u16)
              n480 = Replace Array Subset(array=w850, new element #1=w847, index #1=w848, new element #2=w834, index #2=w839) -> (w849:u16[])
              n481 = Select(t=w844, s=w828, f=myRIO_BRig_RT__Case_NonExp_stateList."DispenseWater_post" ("Enum")) -> (s? t:f=w842:T1)
            }
            frame "DispenseWater_post" {
              # "nCycle"
              # "delay"
              # "Solenoid__R"
              # "nCycle"
              # "delay"
              # "Solenoid__L"
              n482 = call "myRIO_BRig_RT_dataMTrig_Solenoid_N__L.vi"() -> ("output_Solenoid_N__L"=w879:i32)  [unwired: 11 in]
              n483 = call "myRIO_BRig_RT_dataMTrig_Solenoid_delay__L.vi"() -> ("output_Solenoid_delay__L"=w878:i32)  [unwired: 11 in]
              n484 = call "myRIO_BRig_RT_dataMTrig_Solenoid_N__R.vi"() -> ("output_Solenoid_N__R"=w875:i32)  [unwired: 11 in]
              n485 = call "myRIO_BRig_RT_dataMTrig_Solenoid_delay__R.vi"() -> ("output_Solenoid_delay__R"=w874:i32)  [unwired: 11 in]
              n486 = Index Array(array=w881, index #1=w879, index #2=w878, index #3=w875, index #4=w874) -> (element #1=w883:u16, element #2=w882:u16, element #3=w866:u16, element #4=w868:u16)
              n487 = Not Equal To 0?(x=w883) -> (x != 0?=w884:bool)
              n488 = Not Equal To 0?(x=w866) -> (x != 0?=w867:bool)
              n489 = case shown="True" w867 {
                selector: w867 -> [_ w891]
                tunnel: w866 -> [w889 w897]
                tunnel: w868 -> [_ w898]
                tunnel: [w889 w895] -> w865
                tunnel: [u16 0 w894] -> w864
                tunnel: [_ w891] -> w863
                frame False {
                }
                frame True {
                  n490 = Equal To 0?(x=w898) -> (x = 0?=w890:bool)
                  n491 = Decrement(x=w897) -> (x-1=w896:u16)
                  n492 = Select(t=w896, s=w890, f=w897) -> (s? t:f=w895:u16)
                  n493 = Select(t=u16 1, s=w890, f=u16 0) -> (s? t:f=w894:u16)
                }
              }
              n494 = case shown="True" w884 {
                selector: w884 -> [_ w902]
                tunnel: w883 -> [w900 w908]
                tunnel: w882 -> [_ w909]
                tunnel: [w900 w906] -> w877
                tunnel: [u16 0 w905] -> w876
                tunnel: [_ w902] -> w873
                frame False {
                }
                frame True {
                  n495 = Equal To 0?(x=w909) -> (x = 0?=w901:bool)
                  n496 = Decrement(x=w908) -> (x-1=w907:u16)
                  n497 = Select(t=w907, s=w901, f=w908) -> (s? t:f=w906:u16)
                  n498 = Select(t=u16 1, s=w901, f=u16 0) -> (s? t:f=w905:u16)
                }
              }
              n499 = Or(x=w873, y=w863) -> (x .or. y?=w872:bool)
              n500 = Replace Array Subset(array=w881, new element #1=w877, index #1=w879, new element #2=w876, index #2=w878, new element #3=w865, index #3=w875, new element #4=w864, index #4=w874) -> (w880:u16[])
              n501 = Select(t=myRIO_BRig_RT__Case_NonExp_stateList."DispenseWater_pre" ("Enum"), s=w872, f=myRIO_BRig_RT__Case_NonExp_stateList."Idle" ("Enum")) -> (s? t:f=w869:T1)
            }
            frame "TestConnection" {
              n502 = local read "Host Password"() -> (w920:string)
              n503 = local read "Host UserName"() -> (w921:string)
              n504 = call "myRIO_BRig_RT_comm_webdav_testConnect.vi"("input_password"=w920, "input_username"=w921) -> ("output_Iconnected"=w918:bool)  [unwired: 9 in]
              n505 = Select(t="Connection accepted!" ("message"), s=w918, f="Error!") -> (s? t:f=w916:string)
              n506 = One Button Dialog(message=w916) -> ()  [unwired: 1 in, 1 out]
            }
            frame "SendData" {
              n507 = local read "Data Set Prefix"() -> (w924:string)
              n508 = local read "Host Password"() -> (w925:string)
              n509 = local read "Host UserName"() -> (w926:string)
              n510 = call "myRIO_BRig_RT_comm_webdav_sendData_all.vi"("Host Filename Prefix"=w924, "Host Password"=w925, "Host UserName"=w926) -> ()  [unwired: 9 in]
            }
            frame "Get_FPGA_count_per_ms" {
              n511 = case shown="False" w943 {
                selector: w943 -> [w950 _]
                tunnel: w941 -> [_ w963]
                tunnel: [w954 w963] -> w940
                tunnel: w939 -> [w953 w961]
                tunnel: w938 -> [w952 w960]
                tunnel: [w951 w958] -> w937
                tunnel: [w950 w957] -> w936
                frame False {
                  n512 = Get Date/Time In Seconds() -> (seconds since 1Jan1904=w955:timestamp)
                  n513 = xnode "Read/Write Control"("FPGA VI Reference In"=w953, "error in"=w952, "timeTrial"=TRUE) -> ("error out"=w951:errorcluster)  [unwired: 1 out]
                  n514 = To Double Precision Float(number=w955) -> (double precision float=w954:dbl)
                  n515 = local write "get_countPerMS"(w950) -> ()
                }
                frame True {
                  w959 = 1.0
                  n516 = Get Date/Time In Seconds() -> (seconds since 1Jan1904=w964:timestamp)
                  n517 = To Double Precision Float(number=w964) -> (double precision float=w965:dbl)
                  n518 = Subtract(x=w965, y=w963) -> (x-y=w962:dbl)
                  n519 = Less Or Equal?(x=w959, y=w962) -> (x <= y?=w957:bool)
                  n520 = case shown="True" w957 {
                    tunnel: w961 -> [_ w978]
                    tunnel: w960 -> [w966 w977]
                    tunnel: w959 -> [_ w968]
                    tunnel: [w966 w967] -> w958
                    frame False {
                    }
                    frame True {
                      n521 = xnode "Read/Write Control"("FPGA VI Reference In"=w978, "error in"=w977) -> ("FPGA VI Reference Out"=w975:refnum<k20>, "error out"=w974:errorcluster, "count_timeTrial"=w969:u32)
                      n522 = Multiply(x=w968, y=1000.0) -> (x*y=w972:dbl)
                      n523 = To Double Precision Float(number=w969) -> (double precision float=w971:dbl)
                      n524 = Divide(x=w971, y=w972) -> (x/y=w973:dbl)
                      n525 = local write "f_millisec2count"(w973) -> ()
                      n526 = xnode "Read/Write Control"("FPGA VI Reference In"=w975, "error in"=w974, "timeTrial"=FALSE) -> ("error out"=w967:errorcluster)  [unwired: 1 out]
                    }
                  }
                }
              }
              "error out 5" <- w937
              n527 = Select(t=myRIO_BRig_RT__Case_NonExp_stateList."Idle" ("Enum"), s=w936, f=w934) -> (s? t:f=w933:T1)
            }
            frame "End" {
            }
          }
          n528 = local read "MTrig_Audio_trig__R"() -> (w99:bool)
          n529 = local read "MTrig_Audio_trig__L"() -> (w98:bool)
          n530 = local read "START"() -> (w94:bool)
          n531 = local read "STOP_abort"() -> (w93:bool)
          n532 = local read "MTrig_Laser_trig"() -> (w100:bool)
          n533 = call "myRIO_BRig_RT_dataMTrig_main__v2.vi"("input_dataMTrig"=w102, "input_Audio_trig_L"=w98, "input_Audio_trig_R"=w99, "input_Laser_trig"=w100) -> ("output_dataMTrig"=w101:u16[], "output_Audio_L"=w78:bool, "output_Audio_R"=w89:bool, "output_Laser"=w81:bool)  [unwired: 12 in]
          n534 = Or(x=w94, y=w93) -> (x .or. y?=w92:bool)
          n535 = Select(t=myRIO_BRig_RT__Case_NonExp_stateList."End" ("Enum"), s=w92, f=w91) -> (s? t:f=w90:T1)
          n536 = Or(x=w99, y=w100) -> (x .or. y?=w97:bool)
          n537 = Or(x=w97, y=w98) -> (x .or. y?=w96:bool)
          n538 = case shown="True" w96 {
            frame False {
            }
            frame True {
              w118 = FALSE
              n539 = local write "MTrig_Audio_trig__R"(w118) -> ()
              n540 = local write "MTrig_Audio_trig__L"(w118) -> ()
              n541 = local write "MTrig_Laser_trig"(w118) -> ()
            }
          }
          n542 = xnode "Read/Write Control"("FPGA VI Reference In"=w62, "error in"=w61, "A1_SR"=w103, "A3_SL"=w104, "audioTrigger_L"=w78, "audioAmp_L"=w71, "audioFreq_L_kHz"=w73, "audioTrigger_R"=w89, "audioAmp_R"=w72, "audioFreq_R_kHz"=w74, "laserResponse_reward_LED"="laserResponse_reward_LED", "laserResponse_wrong_LED"="laserResponse_wrong_LED", "laserResponse_reward"="laserResponse_reward", "laserResponse_wrong"="laserResponse_wrong", "SelectionState"="SelectionState", "ignoreWrong"="ignoreWrong", "Left(F)_or_Right(T)"="Left(F)_or_Right(T)", "laserMTrig"=w81) -> ("FPGA VI Reference Out"=w112:refnum<k20>, "error out"=w111:errorcluster, "SelectReward"=→"SelectReward":bool, "SelectWrong"=→"SelectWrong":bool)
          n543 = node-c288() -> ()  [unwired: 1 in, 1 out]
          "cState_NonExp" <- w110
        }
        n544 = node-c288(w52) -> ()  [unwired: 1 out]
        n545 = flat-sequence {
          tunnel: w45 -> [w56]
          tunnel: [w56] -> w44
          tunnel: w43 -> [w55]
          tunnel: [w55] -> w42
          frame #0 {
            w54 = FALSE
            n546 = local write "STOP_endBlock"(w54) -> ()
            n547 = local write "STOP_endTrial"(w54) -> ()
          }
        }
      }
      frame True {
        w992 = u8 0
        w994 = FALSE ("SelectionState")
        w999 = u16 0 ("idxDataBlock")
        w1001 = u16 100 ("new element/subarray")
        w1002 = u16 100 ("new element/subarray")
        w1022 = T6 refnum items=["Session NI_WebDAV"] ("output_hSession")
        w1031 = FALSE
        w1032 = u16 0
        w993 = FALSE
        # "audio__L\naudio__R"
        # "Audio params"
        # "nRewards"
        # "idxDataBlock"
        # "Solenoid_Tdelay_R"
        # "Solenoid_Tdelay_L"
        # "RewCalib_N__R"
        # "RewCalib_N__L"
        # "Save dataLick to file\nSend file to Host\nSave dataMTrig\nSend file to Host\nDisconnect"
        # "dataTrial"
        # "dataTrial"
        # "Solenoid_Tcycle_R"
        # "Solenoid_Tcycle_L"
        # "Laser_Tcycle"
        # "Audio_Tcycle_R"
        # "Audio_Tcycle_L"
        # "dataLick"
        # "dataLC"
        # "dataLC"
        # "dataBlock"
        # "dataBlock"
        # "dataMTrig"
        # "dataMTrig"
        # "dataExp"
        # "dataCurrent"
        # "dataExp"
        # "dataCurrent"
        # "spout"
        # "state"
        n548 = call "myRIO_BRig_RT_dataMTrig_Solenoid_Tcycle__L.vi"() -> ("output_Solenoid_Tcycle__L"=w1028:i32)  [unwired: 11 in]
        n549 = call "myRIO_BRig_RT_dataMTrig_Solenoid_Tcycle__R.vi"() -> ("output_Solenoid_Tcycle__R"=w1027:i32)  [unwired: 11 in]
        n550 = call "myRIO_BRig_RT_dataMTrig_Audio_Tcycle__L.vi"() -> ("output_Audio_Tcycle__L"=w1026:i32)  [unwired: 11 in]
        n551 = call "myRIO_BRig_RT_dataMTrig_Audio_Tcycle__R.vi"() -> ("output_Audio_Tcycle__R"=w1025:i32)  [unwired: 11 in]
        n552 = call "myRIO_BRig_RT_dataMTrig_Laser_Tcycle.vi"() -> ("output_Laser_Tcycle"=w1024:i32)  [unwired: 11 in]
        n553 = local read "MTrig_Solenoid_Tcycle__L"() -> (w1007:u16)
        n554 = local read "MTrig_Solenoid_Tcycle__R"() -> (w1006:u16)
        n555 = local read "Tcycle_Reward_L"() -> (w1003:u16)
        n556 = local read "Tcycle_Reward_R"() -> (w1004:u16)
        n557 = local read "MTrig_Laser_Tcycle"() -> (w1005:u16)
        n558 = call "myRIO_BRig_RT_dataMTrig_Solenoid_RewCalib_nCycle__L.vi"() -> ("output_Solenoid_RewCalib_nCycle__L"=w1010:i32)  [unwired: 11 in]
        n559 = call "myRIO_BRig_RT_dataMTrig_Solenoid_Tdelay__L.vi"() -> ("output_Solenoid_Tdelay__L"=w1012:i32)  [unwired: 11 in]
        n560 = call "myRIO_BRig_RT_dataMTrig_Solenoid_RewCalib_nCycle__R.vi"() -> ("output_Solenoid_RewCalib_nCycle__R"=w1011:i32)  [unwired: 11 in]
        n561 = call "myRIO_BRig_RT_dataMTrig_Solenoid_Tdelay__R.vi"() -> ("output_Solenoid_Tdelay__R"=w1013:i32)  [unwired: 11 in]
        n562 = call "myRIO_BRig_RT_dataLick_init.vi"() -> ("output_dataLick"=w1034:u16[][])  [unwired: 11 in]
        n563 = call "myRIO_BRig_RT_dataCurrent_init.vi"() -> ("output_dataCurrent"=w1041:u16[])  [unwired: 11 in]
        n564 = call "myRIO_BRig_RT_dataExp_init.vi"() -> ("output_dataExp"=w1040:u16[])  [unwired: 11 in]
        n565 = call "myRIO_BRig_RT_dataMTrig_init.vi"() -> ("output_dataMTrig"=w1030:u16[])  [unwired: 5 in]
        n566 = call "myRIO_BRig_RT_dataLC_init.vi"() -> ("output_dataLC"=w1038:u16[])  [unwired: 11 in]
        n567 = call "myRIO_BRig_RT_dataBlock_init.vi"() -> ("output_dataBlock"=w1039:u16[][])  [unwired: 11 in]
        n568 = call "myRIO_BRig_RT_dataTrial_init.vi"() -> ("output_dataTrial"=w1023:u16[][])  [unwired: 11 in]
        n569 = xnode "Read/Write Control"("FPGA VI Reference In"=w995, "error in"=w996, "SelectionState"=w994, "laserResponse_reward"=w994, "laserResponse_wrong"=w994, "laserResponse_reward_LED"=w994, "laserResponse_wrong_LED"=w994, "Left(F)_or_Right(T)"=w994, "ignoreWrong"=w994, "SelectionState"=w994) -> ("FPGA VI Reference Out"=w997:refnum<k20>, "error out"=w998:errorcluster)
        n570 = Replace Array Subset(array=w1030, new element #1=w1002, index #1=w1010, new element #2=w1002, index #2=w1011, new element #3=w1001, index #3=w1012, new element #4=w1001, index #4=w1013, new element #5=w1007, index #5=w1028, new element #6=w1006, index #6=w1027, new element #7=w1003, index #7=w1026, new element #8=w1004, index #8=w1025, new element #9=w1005, index #9=w1024) -> (w1029:u16[])
        n571 = Get Date/Time In Seconds() -> (seconds since 1Jan1904=w1009:timestamp)
        n572 = To Double Precision Float(number=w1009) -> (double precision float=w1008:dbl)
        n573 = node-c288() -> (w1049:T3)  [unwired: 4 in]
        n574 = timed-loop {
          timing: w1049 -> [_]
          timing-out: [_] -> w1048
          shift-right: [w1128] -> _
          shift-left: myRIO_BRig_RT__Case_Exp_stateList."Start1" ("Enum") -> [w1159]
          shift-right: [w1180] -> _
          shift-left: enum16{"Left", "Right"}."Left" -> [w1182]
          tunnel: w997 -> [w1179]
          tunnel: w998 -> [w1178]
          shift-right: [w1173] -> _
          shift-left: w1046 -> [w1177]
          shift-right: [w1172] -> _
          shift-left: w1045 -> [w1176]
          tunnel: [w1153] -> w1043
          tunnel: [w1154] -> w1044
          shift-right: [w1155] -> w1014
          shift-left: w1041 -> [w1120]
          shift-right: [w1171] -> _
          shift-left: w1040 -> [w1115]
          shift-right: [w1142] -> w1018
          shift-left: w1029 -> [w1143]
          shift-right: [w1169] -> _
          shift-left: w1039 -> [w1170]
          shift-right: [w1167] -> _
          shift-left: w1038 -> [w1168]
          shift-right: [w1101] -> _
          shift-left: w993 -> [w1166]
          shift-right: [w1157] -> w1020
          shift-left: w1034 -> [w1158]
          shift-right: [w1144] -> _
          shift-left: w1032 -> [w1152]
          shift-right: [w1112] -> _
          shift-left: w992 -> [w1151]
          shift-right: [w1145] -> _
          shift-left: w1032 -> [w1150]
          shift-right: [w1146] -> _
          shift-left: w992 -> [w1149]
          shift-right: [w1113] -> _
          shift-left: w1031 -> [w1147]
          shift-right: [w1114] -> _
          shift-left: w1031 -> [w1148]
          shift-right: [w1126] -> _
          shift-left: w1023 -> [w1127]
          shift-right: [w1125] -> w1016
          shift-left: w1022 -> [w1123]
          shift-right: [w1124] -> w1017
          shift-left: FALSE ("output_Iconnected") -> [w1122]
          tunnel: "Data Set Prefix" -> [w1121]
          tunnel: [w1121] -> w1015
          shift-right: [w1096] -> _
          shift-left: w993 -> [w1119]
          tunnel: w1008 -> [w1116]
          shift-right: [w1110] -> _
          shift-left: 0 ("idxDataBlock") -> [w1111]
          shift-right: [w1107] -> _
          shift-left: w999 -> [w1109]
          shift-right: [w1106] -> _
          shift-left: w999 -> [w1108]
          shift-right: [w1095] -> _
          shift-left: w993 -> [w1102]
          shift-right: [w1098] -> _
          shift-left: w993 -> [w1100]
          shift-right: [w1097] -> _
          shift-left: w993 -> [w1099]
          shift-right: [w1088] -> _
          shift-left: w993 -> [w1089]
          stop <- w1165 stop-if-true
          # "Laser"
          # "Audio R"
          # "Audio L"
          # "Solenoid R"
          # "Solenoid L"
          # "manual triggering"
          # "dataTrial"
          # "dataBlock"
          # "nRewards"
          # "laserOccurred"
          # "dataExp"
          # "dataCurrent"
          # "audio__L\naudio__R"
          # "time stamp"
          # "Audio params"
          # "nRewards"
          # "idxDataBlock"
          # "idxDataBlock"
          # "activate"
          # "audio__L\naudio__R"
          # "amp__R\nfreq__R"
          # "amp__L\nfreq__L"
          # "dataLC"
          # "solenoid__R"
          # "solenoid__L"
          # "Did a lick occur?"
          # "Update lick counter"
          # "spout"
          # "spout"
          # "state"
          # "state"
          n575 = node-c288() -> ()  [unwired: 1 in, 1 out]
          n576 = local read "MTrig_Solenoid_trig__L"() -> (w1140:bool)
          n577 = local read "MTrig_Solenoid_trig__R"() -> (w1139:bool)
          n578 = local read "MTrig_Audio_trig__L"() -> (w1138:bool)
          n579 = local read "MTrig_Audio_trig__R"() -> (w1137:bool)
          n580 = xnode "Read/Write Control"("FPGA VI Reference In"=w1179, "error in"=w1178) -> ("FPGA VI Reference Out"=w1105:refnum<k20>, "error out"=w1104:errorcluster, "A2_LickL"=w1173:u32, "A4_LickR"=w1172:u32)
          "A2" <- w1173
          "A4" <- w1172
          n581 = local read "MTrig_Laser_trig"() -> (w1136:bool)
          n582 = Greater?(x=w1173, y=w1177) -> (0:w1175:bool)
          n583 = Greater?(x=w1172, y=w1176) -> (0:w1174:bool)
          n584 = Or(x=w1175, y=w1174) -> (x .or. y?=w1181:bool)
          n585 = call "myRIO_BRig_RT_dataMTrig_main.vi"("input_dataMTrig"=w1143, "input_Solenoid_trig_L"=w1140, "input_Solenoid_trig_R"=w1139, "input_Audio_trig_L"=w1138, "input_Audio_trig_R"=w1137, "input_Laser_trig"=w1136) -> ("output_Laser"=w1093:bool, "output_dataMTrig"=w1142:u16[], "output_Solenoid_L"=w1130:bool, "output_Solenoid_R"=w1132:bool, "output_Audio_L"=w1134:bool, "output_Audio_R"=w1135:bool)  [unwired: 8 in]
          n586 = Compound Arithmetic op=OR(w1140, w1139, w1138, w1137, w1136) -> (w1141:bool)
          n587 = case shown="True" w1141 {
            frame False {
            }
            frame True {
              w1183 = FALSE
              n588 = local write "MTrig_Solenoid_trig__L"(w1183) -> ()
              n589 = local write "MTrig_Solenoid_trig__R"(w1183) -> ()
              n590 = local write "MTrig_Audio_trig__L"(w1183) -> ()
              n591 = local write "MTrig_Audio_trig__R"(w1183) -> ()
              n592 = local write "MTrig_Laser_trig"(w1183) -> ()
            }
          }
          n593 = case shown="\"setSettings_Laser\"" w1159 {
            selector: w1159 -> [_ _ _ _ _ _ _ _ _ _ _ _ _ _ _ _ _ _ _ _ w1920 _ w1985 _ _ _ _ _ w2127 _ w2202 _ _ _ _ _ w2331 _ w2407 _ w2471 _ w2515 _ _ w2585 _ _ _ _ _ w2757 _ _ _ _ _ _ _ _ _ _ _ _ _ _ _ _ _ _ _]
            tunnel: [myRIO_BRig_RT__Case_Exp_stateList."Start2" ("Enum") myRIO_BRig_RT__Case_Exp_stateList."Start3" ("Enum") myRIO_BRig_RT__Case_Exp_stateList."saveSettings1" ("Enum") myRIO_BRig_RT__Case_Exp_stateList."saveSettings2" ("Enum") myRIO_BRig_RT__Case_Exp_stateList."saveSettings3" ("Enum") myRIO_BRig_RT__Case_Exp_stateList."saveSettings4_LC_ENL" ("Enum") myRIO_BRig_RT__Case_Exp_stateList."saveSettings5_LC_Cue" ("Enum") myRIO_BRig_RT__Case_Exp_stateList."saveSettings6_LC_Other" ("Enum") myRIO_BRig_RT__Case_Exp_stateList."setSettings_Audio" ("Enum") myRIO_BRig_RT__Case_Exp_stateList."setSettings_Laser" ("Enum") myRIO_BRig_RT__Case_Exp_stateList."commConnect" ("Enum") w1681 myRIO_BRig_RT__Case_Exp_stateList."initTrial" ("Enum") w1725 myRIO_BRig_RT__Case_Exp_stateList."initTrial3" ("Enum") myRIO_BRig_RT__Case_Exp_stateList."initTrial_LC_ENL1" ("Enum") myRIO_BRig_RT__Case_Exp_stateList."ENL1_pre" ("Enum") myRIO_BRig_RT__Case_Exp_stateList."initTrial_LC_Cue1" ("Enum") myRIO_BRig_RT__Case_Exp_stateList."initTrial4" ("Enum") w1879 w1917 myRIO_BRig_RT__Case_Exp_stateList."ENL1Penalty" ("Enum") w1986 myRIO_BRig_RT__Case_Exp_stateList."endExp" ("Enum") myRIO_BRig_RT__Case_Exp_stateList."endExp" ("Enum") myRIO_BRig_RT__Case_Exp_stateList."endExp" ("Enum") myRIO_BRig_RT__Case_Exp_stateList."endExp" ("Enum") w2081 w2126 myRIO_BRig_RT__Case_Exp_stateList."Cue1Penalty" ("Enum") w2200 myRIO_BRig_RT__Case_Exp_stateList."endExp" ("Enum") myRIO_BRig_RT__Case_Exp_stateList."endExp" ("Enum") myRIO_BRig_RT__Case_Exp_stateList."endExp" ("Enum") myRIO_BRig_RT__Case_Exp_stateList."endExp" ("Enum") w2288 w2339 myRIO_BRig_RT__Case_Exp_stateList."SelectReward" ("Enum") w2408 myRIO_BRig_RT__Case_Exp_stateList."SelectRewardPost" ("Enum") w2472 myRIO_BRig_RT__Case_Exp_stateList."SelectWrong" ("Enum") w2511 myRIO_BRig_RT__Case_Exp_stateList."endTrial1" ("Enum") myRIO_BRig_RT__Case_Exp_stateList."SelectTimeout" ("Enum") w2587 myRIO_BRig_RT__Case_Exp_stateList."endTrial1" ("Enum") myRIO_BRig_RT__Case_Exp_stateList."endTrial2" ("Enum") myRIO_BRig_RT__Case_Exp_stateList."saveData_dataBlock" ("Enum") w2670 w2740 w2757 myRIO_BRig_RT__Case_Exp_stateList."initBlock" ("Enum") w2784 myRIO_BRig_RT__Case_Exp_stateList."commUpload_dataCurrent" ("Enum") myRIO_BRig_RT__Case_Exp_stateList."commUpload_dataExp" ("Enum") myRIO_BRig_RT__Case_Exp_stateList."commUpload_dataLC" ("Enum") myRIO_BRig_RT__Case_Exp_stateList."commUpload_dataTrial" ("Enum") myRIO_BRig_RT__Case_Exp_stateList."endTrial3" ("Enum") myRIO_BRig_RT__Case_Exp_stateList."saveData_dataCurrent" ("Enum") myRIO_BRig_RT__Case_Exp_stateList."saveData_dataExp" ("Enum") myRIO_BRig_RT__Case_Exp_stateList."saveData_dataLC" ("Enum") myRIO_BRig_RT__Case_Exp_stateList."saveData_dataTrial" ("Enum") myRIO_BRig_RT__Case_Exp_stateList."commUpload_pre" ("Enum") myRIO_BRig_RT__Case_Exp_stateList."empty_endBlock2" ("Enum") myRIO_BRig_RT__Case_Exp_stateList."initBlock" ("Enum") myRIO_BRig_RT__Case_Exp_stateList."empty_endTrial2" ("Enum") myRIO_BRig_RT__Case_Exp_stateList."empty_endTrial3" ("Enum") myRIO_BRig_RT__Case_Exp_stateList."empty_endTrial4" ("Enum") myRIO_BRig_RT__Case_Exp_stateList."empty_endTrial5" ("Enum") myRIO_BRig_RT__Case_Exp_stateList."initTrial" ("Enum")] -> w1128
            tunnel: [w1209 w1228 w1250 w1305 w1353 w1420 w1472 w1524 w1568 w1594 w1653 w1657 w1689 w1706 w1741 w1771 w1804 w1828 w1854 w1895 w1933 w1963 w1990 w2006 w2028 w2047 w2066 w2100 w2148 w2173 w2199 w2220 w2241 w2260 w2279 w2299 w2357 w2382 w2405 w2419 w2469 w2493 w2525 w2546 w2566 w2598 w2621 w2633 w2652 w2694 w2713 w2756 w2773 w2787 w2821 w2842 w2863 w2884 w2905 w2933 w2953 w2980 w3000 w3025 w3044 w3063 w3082 w3101 w3120 w3139 w3158] -> w1180
            tunnel: w1182 -> [w1209 w1228 w1250 w1305 w1353 w1420 w1472 w1524 w1568 w1594 w1653 w1680 w1689 w1706 w1741 w1771 w1804 w1828 w1854 w1895 w1933 w1963 w1990 w2006 w2028 w2047 w2066 w2100 w2148 w2173 w2199 w2220 w2241 w2260 w2279 w2299 w2357 w2382 w2405 w2419 w2469 w2493 w2525 w2546 w2566 w2598 w2621 w2633 w2652 w2694 w2713 w2756 w2773 w2787 w2821 w2842 w2863 w2884 w2905 w2933 w2953 w2980 w3000 w3025 w3044 w3063 w3082 w3101 w3120 w3139 w3158]
            tunnel: w1181 -> [w1212 w1231 w1247 w1308 w1356 w1423 w1475 w1527 w1571 w1597 w1656 w1674 w1700 w1726 w1759 w1787 w1818 w1841 w1867 w1882 w1914 w1966 w1993 w2012 w2031 w2050 w2069 w2080 w2125 w2181 w2206 w2225 w2244 w2263 w2282 w2297 w2355 w2392 w2415 w2450 w2477 w2504 w2528 w2545 w2578 w2603 w2618 w2641 w2651 w2705 w2739 w2760 w2770 w2796 w2824 w2845 w2866 w2887 w2908 w2936 w2956 w2983 w3003 w3028 w3047 w3066 w3085 w3104 w3123 w3142 w3161]
            tunnel: w1175 -> [w1211 w1230 w1248 w1307 w1355 w1422 w1474 w1526 w1570 w1596 w1655 w1673 w1699 w1727 w1758 w1788 w1819 w1842 w1868 w1905 w1935 w1965 w1992 w2011 w2030 w2049 w2068 w2114 w2149 w2180 w2205 w2224 w2243 w2262 w2281 w2298 w2354 w2391 w2414 w2449 w2476 w2503 w2527 w2544 w2577 w2602 w2619 w2642 w2650 w2704 w2738 w2759 w2771 w2797 w2823 w2844 w2865 w2886 w2907 w2935 w2955 w2982 w3002 w3027 w3046 w3065 w3084 w3103 w3122 w3141 w3160]
            tunnel: w1174 -> [w1210 w1229 w1249 w1306 w1354 w1421 w1473 w1525 w1569 w1595 w1654 w1672 w1698 w1728 w1757 w1789 w1820 w1843 w1869 w1904 w1934 w1964 w1991 w2010 w2029 w2048 w2067 w2113 w2150 w2179 w2204 w2223 w2242 w2261 w2280 w2317 w2358 w2390 w2413 w2448 w2475 w2502 w2526 w2543 w2576 w2601 w2620 w2643 w2649 w2703 w2737 w2758 w2772 w2798 w2822 w2843 w2864 w2885 w2906 w2934 w2954 w2981 w3001 w3026 w3045 w3064 w3083 w3102 w3121 w3140 w3159]
            tunnel: [w1212 w1231 w1247 w1308 w1356 w1423 w1475 w1527 w1571 w1597 w1656 w1674 w1700 w1726 w1759 w1787 w1818 w1841 w1867 w1882 w1914 w1966 w1993 w2012 w2031 w2050 w2069 w2080 w2125 w2181 w2206 w2225 w2244 w2263 w2282 w2297 w2355 w2392 w2415 w2450 w2477 w2504 w2528 w2545 w2578 w2603 w2618 w2641 w2651 w2705 w2739 w2760 w2770 w2796 w2824 w2845 w2866 w2887 w2908 w2936 w2956 w2983 w3003 w3028 w3047 w3066 w3085 w3104 w3123 w3142 w3161] -> w1162
            tunnel: [w1211 w1230 w1248 w1307 w1355 w1422 w1474 w1526 w1570 w1596 w1655 w1673 w1699 w1727 w1758 w1788 w1819 w1842 w1868 w1905 w1935 w1965 w1992 w2011 w2030 w2049 w2068 w2114 w2149 w2180 w2205 w2224 w2243 w2262 w2281 w2298 w2354 w2391 w2414 w2449 w2476 w2503 w2527 w2544 w2577 w2602 w2619 w2642 w2650 w2704 w2738 w2759 w2771 w2797 w2823 w2844 w2865 w2886 w2907 w2935 w2955 w2982 w3002 w3027 w3046 w3065 w3084 w3103 w3122 w3141 w3160] -> w1161
            tunnel: [w1210 w1229 w1249 w1306 w1354 w1421 w1473 w1525 w1569 w1595 w1654 w1672 w1698 w1728 w1757 w1789 w1820 w1843 w1869 w1904 w1934 w1964 w1991 w2010 w2029 w2048 w2067 w2113 w2150 w2179 w2204 w2223 w2242 w2261 w2280 w2317 w2358 w2390 w2413 w2448 w2475 w2502 w2526 w2543 w2576 w2601 w2620 w2643 w2649 w2703 w2737 w2758 w2772 w2798 w2822 w2843 w2864 w2885 w2906 w2934 w2954 w2981 w3001 w3026 w3045 w3064 w3083 w3102 w3121 w3140 w3159] -> w1160
            tunnel: w1120 -> [w1208 w1227 w1246 w1272 w1329 w1397 w1471 w1523 w1567 w1592 w1613 w1679 w1688 w1724 w1730 w1772 w1799 w1825 w1853 w1894 w1919 w1957 w1989 w2007 w2027 w2046 w2065 w2084 w2145 w2172 w2203 w2221 w2240 w2259 w2278 w2308 w2335 w2374 w2410 w2421 w2474 w2494 w2524 w2542 w2567 w2600 w2617 w2630 w2654 w2674 w2711 w2755 w2774 w2799 w2818 w2839 w2860 w2881 w2892 w2922 w2941 w2965 w2997 w3014 w3034 w3053 w3072 w3091 w3110 w3129 w3148]
            tunnel: w1115 -> [w1207 w1226 w1245 w1303 w1351 w1417 w1469 w1521 w1565 w1585 w1649 w1678 w1697 w1723 w1738 w1770 w1806 w1831 w1857 w1897 w1932 w1956 w1987 w2009 w2026 w2045 w2064 w2102 w2147 w2170 w2198 w2222 w2239 w2258 w2277 w2310 w2356 w2388 w2412 w2442 w2470 w2495 w2522 w2541 w2569 w2597 w2616 w2640 w2657 w2673 w2730 w2754 w2775 w2800 w2817 w2838 w2859 w2880 w2893 w2930 w2950 w2961 w2996 w3022 w3041 w3060 w3079 w3098 w3117 w3136 w3155]
            tunnel: [w1208 w1227 w1246 w1272 w1329 w1396 w1471 w1523 w1567 w1592 w1635 w1663 w1688 w1712 w1730 w1772 w1799 w1824 w1852 w1898 w1918 w1958 w1988 w2007 w2027 w2046 w2065 w2109 w2144 w2171 w2201 w2221 w2240 w2259 w2278 w2311 w2330 w2389 w2409 w2443 w2473 w2496 w2523 w2542 w2570 w2599 w2617 w2629 w2653 w2674 w2709 w2755 w2774 w2799 w2818 w2839 w2860 w2881 w2892 w2922 w2941 w2965 w2997 w3014 w3034 w3053 w3072 w3091 w3110 w3129 w3148] -> w1156
            tunnel: [w1207 w1226 w1245 w1302 w1350 w1412 w1469 w1521 w1565 w1585 w1649 w1677 w1697 w1722 w1738 w1770 w1806 w1831 w1857 w1897 w1932 w1956 w1987 w2009 w2026 w2045 w2064 w2102 w2147 w2170 w2198 w2222 w2239 w2258 w2277 w2310 w2356 w2388 w2412 w2442 w2470 w2495 w2522 w2541 w2569 w2597 w2616 w2640 w2657 w2673 w2730 w2754 w2775 w2800 w2817 w2838 w2859 w2880 w2893 w2930 w2950 w2964 w2996 w3022 w3041 w3060 w3079 w3098 w3117 w3136 w3155] -> w1171
            tunnel: [_ _ _ _ _ _ _ _ _ _ _ _ _ _ _ _ _ _ _ _ _ _ _ _ _ _ _ _ _ _ _ _ _ _ _ _ _ _ w2403 _ _ _ _ _ _ _ _ _ _ _ _ _ _ _ _ _ _ _ _ _ _ _ _ _ _ _ _ _ _ _ _] -> w1131
            tunnel: [_ _ _ _ _ _ _ _ _ _ _ _ _ _ _ _ _ _ _ _ _ _ _ _ _ _ _ _ _ _ _ _ _ _ _ _ _ _ w2404 _ _ _ _ _ _ _ _ _ _ _ _ _ _ _ _ _ _ _ _ _ _ _ _ _ _ _ _ _ _ _ _] -> w1133
            tunnel: w1170 -> [w1205 w1224 w1243 w1274 w1331 w1418 w1470 w1522 w1566 w1590 w1650 w1675 w1690 w1720 w1750 w1785 w1816 w1821 w1849 w1896 w1931 w1953 w1983 w2008 w2024 w2043 w2062 w2108 w2146 w2169 w2196 w2218 w2237 w2256 w2275 w2309 w2352 w2380 w2411 w2423 w2467 w2492 w2520 w2539 w2568 w2596 w2614 w2632 w2659 w2701 w2722 w2752 w2777 w2802 w2815 w2836 w2857 w2878 w2902 w2916 w2943 w2971 w2990 w3016 w3035 w3054 w3073 w3092 w3111 w3130 w3149]
            tunnel: [w1205 w1224 w1243 w1274 w1331 w1418 w1470 w1522 w1566 w1590 w1650 w1675 w1687 w1720 w1750 w1785 w1816 w1821 w1849 w1896 w1931 w1953 w1983 w2008 w2024 w2043 w2062 w2108 w2146 w2169 w2196 w2218 w2237 w2256 w2275 w2309 w2352 w2380 w2411 w2422 w2467 w2492 w2520 w2539 w2568 w2596 w2614 w2631 w2659 w2701 w2722 w2752 w2777 w2802 w2815 w2836 w2857 w2878 w2902 w2916 w2943 w2971 w2990 w3016 w3035 w3054 w3073 w3092 w3111 w3130 w3149] -> w1169
            tunnel: w1168 -> [w1206 w1225 w1244 w1273 w1330 w1419 w1467 w1519 w1563 w1591 w1651 w1676 w1696 w1721 w1729 w1786 w1817 w1829 w1855 w1893 w1913 w1954 w1984 w2005 w2025 w2044 w2063 w2107 w2124 w2168 w2197 w2219 w2238 w2257 w2276 w2307 w2353 w2381 w2406 w2440 w2468 w2491 w2521 w2540 w2565 w2594 w2615 w2639 w2658 w2702 w2729 w2753 w2776 w2801 w2816 w2837 w2858 w2879 w2903 w2929 w2949 w2977 w2988 w3021 w3040 w3059 w3078 w3097 w3116 w3135 w3154]
            tunnel: [w1206 w1225 w1244 w1273 w1330 w1419 w1468 w1520 w1564 w1591 w1651 w1676 w1696 w1721 w1729 w1786 w1817 w1829 w1855 w1893 w1913 w1954 w1984 w2005 w2025 w2044 w2063 w2107 w2124 w2168 w2197 w2219 w2238 w2257 w2276 w2307 w2353 w2381 w2406 w2440 w2468 w2491 w2521 w2540 w2565 w2594 w2615 w2639 w2658 w2702 w2729 w2753 w2776 w2801 w2816 w2837 w2858 w2879 w2903 w2929 w2949 w2977 w2988 w3021 w3040 w3059 w3078 w3097 w3116 w3135 w3154] -> w1167
            tunnel: w1166 -> [_ _ _ _ _ _ _ _ _ _ _ _ _ _ _ _ _ _ _ w1878 w1906 w1939 w1972 _ _ _ _ _ w2118 w2155 _ _ _ _ _ _ _ _ _ _ _ _ _ _ _ w2595 _ _ _ _ _ _ _ _ _ _ _ _ _ _ _ _ _ _ _ _ _ _ _ _ _]
            tunnel: [_ _ _ _ _ _ _ _ _ _ _ _ _ _ _ _ _ _ _ _ _ _ _ _ _ _ _ _ _ _ _ _ _ _ _ _ _ _ _ _ _ _ _ _ _ _ _ _ _ _ _ TRUE _ _ _ _ _ _ _ _ _ _ _ _ _ _ _ _ _ _ _] -> w1163
            tunnel: w1152 -> [w1203 w1222 w1241 w1264 w1324 w1407 w1454 w1506 w1535 _ w1641 w1671 w1695 w1719 w1749 w1784 w1815 w1840 w1866 w1892 w1930 w1951 w1982 w2003 w2022 w2041 w2060 w2106 w2141 w2166 w2195 w2216 w2235 w2254 w2273 w2306 w2351 w2370 w2402 w2438 w2466 w2489 w2519 w2538 w2563 w2593 w2613 w2637 w2663 w2700 w2726 w2750 w2768 w2795 w2813 w2834 w2855 w2876 w2900 w2927 w2947 w2975 w2994 w3020 w3039 w3058 w3077 w3096 w3115 w3134 w3153]
            tunnel: w1151 -> [w1202 w1221 w1240 w1263 w1323 w1406 w1453 w1505 w1536 _ w1640 w1670 w1694 w1718 w1748 w1783 w1814 w1839 w1865 w1891 w1929 w1950 w1981 w2002 w2021 w2040 w2059 w2105 w2140 w2165 w2194 w2215 w2234 w2253 w2272 w2305 w2350 w2369 w2401 w2437 w2465 w2488 w2518 w2537 w2562 w2592 w2612 w2636 w2662 w2699 w2725 w2749 w2767 w2794 w2812 w2833 w2854 w2875 w2899 w2926 w2946 w2974 w2993 w3019 w3038 w3057 w3076 w3095 w3114 w3133 w3152]
            tunnel: w1150 -> [w1201 w1220 w1239 w1262 w1322 w1405 w1452 w1504 w1537 _ w1639 w1669 w1693 w1717 w1747 w1782 w1813 w1838 w1864 w1890 w1928 w1949 w1980 w2001 w2020 w2039 w2058 w2104 w2139 w2164 w2193 w2214 w2233 w2252 w2271 w2304 w2349 w2368 w2400 w2436 w2464 w2487 w2517 w2536 w2561 w2591 w2611 w2635 w2661 w2698 w2724 w2748 w2766 w2793 w2811 w2832 w2853 w2874 w2898 w2925 w2945 w2973 w2992 w3018 w3037 w3056 w3075 w3094 w3113 w3132 w3151]
            tunnel: w1149 -> [w1200 w1219 w1238 w1261 w1321 w1404 w1451 w1503 w1538 _ w1638 w1668 w1692 w1716 w1746 w1781 w1812 w1837 w1863 w1889 w1927 w1948 w1979 w2000 w2019 w2038 w2057 w2103 w2138 w2163 w2192 w2213 w2232 w2251 w2270 w2303 w2348 w2367 w2399 w2435 w2463 w2486 w2516 w2535 w2560 w2590 w2610 w2634 w2660 w2697 w2723 w2747 w2765 w2792 w2810 w2831 w2852 w2873 w2897 w2924 w2944 w2972 w2991 w3017 w3036 w3055 w3074 w3093 w3112 w3131 w3150]
            tunnel: w1148 -> [_ _ _ _ _ _ _ _ _ _ _ _ _ _ _ _ _ _ _ _ _ _ _ _ _ _ _ _ w2143 _ _ _ _ _ _ _ _ _ _ _ _ _ _ _ _ _ _ _ _ _ _ _ _ _ _ _ _ _ _ _ _ _ _ _ _ _ _ _ _ _ _]
            tunnel: w1147 -> [_ _ _ _ _ _ _ _ _ _ _ _ _ _ _ _ _ _ _ _ _ _ _ _ _ _ _ _ w2142 _ _ _ _ _ _ _ _ _ _ _ _ _ _ _ _ _ _ _ _ _ _ _ _ _ _ _ _ _ _ _ _ _ _ _ _ _ _ _ _ _ _]
            tunnel: [w1203 w1222 w1241 w1264 w1324 w1407 w1454 w1506 w1535 w1584 w1641 w1671 w1695 w1719 w1749 w1784 w1815 w1840 w1866 w1892 w1930 w1951 w1982 w2003 w2022 w2041 w2060 w2106 w2141 w2166 w2195 w2216 w2235 w2254 w2273 w2306 w2351 w2370 w2402 w2438 w2466 w2489 w2519 w2538 w2563 w2593 w2613 w2637 w2663 w2700 w2726 w2750 w2768 w2795 w2813 w2834 w2855 w2876 w2900 w2927 w2947 w2975 w2994 w3020 w3039 w3058 w3077 w3096 w3115 w3134 w3153] -> w1144
            tunnel: [w1202 w1221 w1240 w1263 w1323 w1406 w1453 w1505 w1536 w1575 w1640 w1670 w1694 w1718 w1748 w1783 w1814 w1839 w1865 w1891 w1929 w1950 w1981 w2002 w2021 w2040 w2059 w2105 w2140 w2165 w2194 w2215 w2234 w2253 w2272 w2305 w2350 w2369 w2401 w2437 w2465 w2488 w2518 w2537 w2562 w2592 w2612 w2636 w2662 w2699 w2725 w2749 w2767 w2794 w2812 w2833 w2854 w2875 w2899 w2926 w2946 w2974 w2993 w3019 w3038 w3057 w3076 w3095 w3114 w3133 w3152] -> w1112
            tunnel: [w1201 w1220 w1239 w1262 w1322 w1405 w1452 w1504 w1537 w1583 w1639 w1669 w1693 w1717 w1747 w1782 w1813 w1838 w1864 w1890 w1928 w1949 w1980 w2001 w2020 w2039 w2058 w2104 w2139 w2164 w2193 w2214 w2233 w2252 w2271 w2304 w2349 w2368 w2400 w2436 w2464 w2487 w2517 w2536 w2561 w2591 w2611 w2635 w2661 w2698 w2724 w2748 w2766 w2793 w2811 w2832 w2853 w2874 w2898 w2925 w2945 w2973 w2992 w3018 w3037 w3056 w3075 w3094 w3113 w3132 w3151] -> w1145
            tunnel: [w1200 w1219 w1238 w1261 w1321 w1404 w1451 w1503 w1538 w1573 w1638 w1668 w1692 w1716 w1746 w1781 w1812 w1837 w1863 w1889 w1927 w1948 w1979 w2000 w2019 w2038 w2057 w2103 w2138 w2163 w2192 w2213 w2232 w2251 w2270 w2303 w2348 w2367 w2399 w2435 w2463 w2486 w2516 w2535 w2560 w2590 w2610 w2634 w2660 w2697 w2723 w2747 w2765 w2792 w2810 w2831 w2852 w2873 w2897 w2924 w2944 w2972 w2991 w3017 w3036 w3055 w3074 w3093 w3112 w3131 w3150] -> w1146
            tunnel: [_ _ _ _ _ _ _ _ _ _ _ _ _ _ _ _ _ _ _ _ _ _ _ _ _ _ _ w2093 w2143 _ _ _ _ _ _ _ _ _ _ _ _ _ _ _ _ _ _ _ _ _ _ _ _ _ _ _ _ _ _ _ _ _ _ _ _ _ _ _ _ _ _] -> w1114
            tunnel: [_ _ _ _ _ _ _ _ _ _ _ _ _ _ _ _ _ _ _ _ _ _ _ _ _ _ _ w2092 w2142 _ _ _ _ _ _ _ _ _ _ _ _ _ _ _ _ _ _ _ _ _ _ _ _ _ _ _ _ _ _ _ _ _ _ _ _ _ _ _ _ _ _] -> w1113
            tunnel: w1127 -> [w1199 w1218 w1237 w1260 w1320 w1403 w1450 w1502 w1534 w1582 w1648 w1667 w1691 w1715 w1732 w1774 w1798 w1823 w1851 w1888 w1926 w1947 w1978 w1999 w2018 w2037 w2056 w2091 w2137 w2162 w2191 w2212 w2231 w2250 w2269 w2302 w2347 w2364 w2398 w2434 w2462 w2483 w2510 w2534 w2557 w2584 w2609 w2628 w2656 w2690 w2721 w2746 w2778 w2803 w2814 w2835 w2856 w2877 w2901 w2928 w2948 w2976 w2995 w3011 w3033 w3052 w3071 w3090 w3109 w3128 w3147]
            tunnel: [w1199 w1218 w1237 w1260 w1320 w1403 w1450 w1502 w1534 w1582 w1648 w1667 w1691 w1715 w1731 w1773 w1791 w1822 w1850 w1888 w1926 w1947 w1978 w1999 w2018 w2037 w2056 w2091 w2137 w2162 w2191 w2212 w2231 w2250 w2269 w2302 w2347 w2364 w2398 w2434 w2462 w2483 w2510 w2534 w2557 w2584 w2609 w2628 w2655 w2690 w2721 w2746 w2778 w2803 w2814 w2835 w2856 w2877 w2901 w2928 w2948 w2976 w2995 w3011 w3033 w3052 w3071 w3090 w3109 w3128 w3147] -> w1126
            tunnel: [w1198 w1217 w1236 w1259 w1319 w1402 w1449 w1501 w1533 w1581 w1647 w1666 w1702 w1714 w1752 w1780 w1811 w1836 w1862 w1887 w1925 w1946 w1977 w1998 w2017 w2036 w2055 w2090 w2136 w2161 w2190 w2211 w2230 w2249 w2268 w2301 w2346 w2363 w2397 w2433 w2461 w2482 w2509 w2533 w2556 w2583 w2608 w2627 w2648 w2696 w2720 w2744 w2779 w2789 w2809 w2830 w2851 w2872 w2896 w2932 w2952 w2979 w2999 w3024 w3043 w3062 w3081 w3100 w3119 w3138 w3157] -> w1125
            tunnel: [w1197 w1216 w1235 w1258 w1318 w1401 w1448 w1500 w1532 w1580 w1646 w1665 w1701 w1713 w1751 w1779 w1810 w1835 w1861 w1886 w1924 w1945 w1976 w1997 w2016 w2035 w2054 w2089 w2135 w2160 w2189 w2210 w2229 w2248 w2267 w2300 w2345 w2362 w2396 w2432 w2460 w2481 w2508 w2532 w2555 w2582 w2607 w2626 w2647 w2695 w2719 w2745 w2761 w2786 w2819 w2840 w2861 w2882 w2904 w2931 w2951 w2978 w2998 w3023 w3042 w3061 w3080 w3099 w3118 w3137 w3156] -> w1124
            tunnel: w1123 -> [w1198 w1217 w1236 w1259 w1319 w1402 w1449 w1501 w1533 w1581 w1647 w1666 w1702 w1714 w1752 w1780 w1811 w1836 w1862 w1887 w1925 w1946 w1977 w1998 w2017 w2036 w2055 w2090 w2136 w2161 w2190 w2211 w2230 w2249 w2268 w2301 w2346 w2363 w2397 w2433 w2461 w2482 w2509 w2533 w2556 w2583 w2608 w2627 w2648 w2696 w2720 w2744 _ w2789 w2809 w2830 w2851 w2872 w2896 w2932 w2952 w2979 w2999 w3024 w3043 w3062 w3081 w3100 w3119 w3138 w3157]
            tunnel: w1122 -> [w1197 w1216 w1235 w1258 w1318 w1401 w1448 w1500 w1532 w1580 w1646 w1665 w1701 w1713 w1751 w1779 w1810 w1835 w1861 w1886 w1924 w1945 w1976 w1997 w2016 w2035 w2054 w2089 w2135 w2160 w2189 w2210 w2229 w2248 w2267 w2300 w2345 w2362 w2396 w2432 w2460 w2481 w2508 w2532 w2555 w2582 w2607 w2626 w2647 w2695 w2719 w2745 _ w2786 w2819 w2840 w2861 w2882 w2904 w2931 w2951 w2978 w2998 w3023 w3042 w3061 w3080 w3099 w3118 w3137 w3156]
            tunnel: w1121 -> [_ _ _ _ _ _ _ _ _ _ _ _ _ _ _ _ _ _ _ _ _ _ _ _ _ _ _ _ _ _ _ _ _ _ _ _ _ _ _ _ _ _ _ _ _ _ _ _ _ _ _ _ _ _ w2807 w2828 w2849 w2870 w2894 _ _ _ _ _ _ _ _ _ _ _ _]
            tunnel: w1119 -> [_ _ _ _ _ _ _ _ _ _ _ _ _ _ _ _ w1803 _ w1846 w1875 w1911 w1937 w1968 _ _ _ _ w2071 w2116 w2154 w2183 _ _ _ _ _ _ _ _ _ _ _ _ _ _ _ _ _ _ _ _ _ _ _ _ _ _ _ _ _ _ _ _ _ _ _ _ _ _ _ _]
            tunnel: w1116 -> [_ _ _ _ _ _ _ _ _ _ _ _ _ _ _ _ _ _ _ _ _ _ _ _ _ _ _ _ _ _ _ _ _ _ _ _ _ _ _ _ _ _ _ _ _ _ _ _ _ _ _ _ _ _ _ _ _ _ _ _ _ w2966 _ _ _ _ _ _ _ _ _]
            tunnel: [w1196 w1215 w1234 w1257 w1317 w1400 w1447 w1499 w1531 w1579 w1645 w1660 w1685 w1709 w1753 w1778 w1809 w1834 w1860 w1885 w1923 w1944 w1975 w1996 w2015 w2034 w2053 w2088 w2134 w2159 w2188 w2209 w2228 w2247 w2266 w2296 w2344 w2361 w2395 w2417 w2459 w2480 w2507 w2531 w2554 w2581 w2606 w2625 w2646 w2693 w2706 w2743 w2764 w2788 w2806 w2827 w2848 w2869 w2891 w2911 w2940 w2960 w2987 w3007 w3032 w3051 w3070 w3089 w3108 w3127 w3146] -> w1110
            tunnel: w1111 -> [w1196 w1215 w1234 w1257 w1317 w1400 w1447 w1499 w1531 w1579 w1645 w1660 _ w1709 w1753 w1778 w1809 w1834 w1860 w1885 w1923 w1944 w1975 w1996 w2015 w2034 w2053 w2088 w2134 w2159 w2188 w2209 w2228 w2247 w2266 w2296 w2344 w2361 w2395 w2417 w2459 w2480 w2507 w2531 w2554 w2581 w2606 w2625 w2646 w2693 w2707 w2743 w2764 w2788 w2806 w2827 w2848 w2869 w2891 w2911 w2940 w2960 w2987 w3007 w3032 w3051 w3070 w3089 w3108 w3127 w3146]
            tunnel: w1109 -> [w1195 w1214 w1233 w1256 w1316 w1399 w1446 w1498 w1530 w1578 w1644 w1659 w1684 w1708 w1745 w1777 w1808 w1833 w1859 w1884 w1922 w1943 w1974 w1995 w2014 w2033 w2052 w2087 w2133 w2158 w2187 w2208 w2227 w2246 w2265 w2295 w2343 w2360 w2394 w2431 w2458 w2479 w2506 w2530 w2553 w2580 w2605 w2624 w2645 w2692 w2718 w2742 w2763 w2791 w2805 w2826 w2847 w2868 w2890 w2910 w2939 w2959 w2986 w3006 w3031 w3050 w3069 w3088 w3107 w3126 w3145]
            tunnel: w1108 -> [w1194 w1213 w1232 w1255 w1315 w1398 w1445 w1497 w1529 w1577 w1643 w1658 w1683 w1707 w1744 w1776 w1807 w1832 w1858 w1883 w1921 w1942 w1973 w1994 w2013 w2032 w2051 w2086 w2132 w2157 w2186 w2207 w2226 w2245 w2264 w2294 w2342 w2359 w2393 w2428 w2457 w2478 w2505 w2529 w2552 w2579 w2604 w2623 w2644 w2691 w2717 w2741 w2762 w2790 w2804 w2825 w2846 w2867 w2889 w2909 w2938 w2958 w2985 w3005 w3030 w3049 w3068 w3087 w3106 w3125 w3144]
            tunnel: [w1195 w1214 w1233 w1256 w1316 w1399 w1446 w1498 w1530 w1578 w1644 w1659 w1684 w1708 w1745 w1777 w1808 w1833 w1859 w1884 w1922 w1943 w1974 w1995 w2014 w2033 w2052 w2087 w2133 w2158 w2187 w2208 w2227 w2246 w2265 w2295 w2343 w2360 w2394 w2430 w2458 w2479 w2506 w2530 w2553 w2580 w2605 w2624 w2645 w2692 w2718 w2742 w2763 w2791 w2805 w2826 w2847 w2868 w2890 w2910 w2939 w2959 w2986 w3006 w3031 w3050 w3069 w3088 w3107 w3126 w3145] -> w1107
            tunnel: [w1194 w1213 w1232 w1255 w1315 w1398 w1445 w1497 w1529 w1577 w1643 w1658 w1683 w1707 w1744 w1776 w1807 w1832 w1858 w1883 w1921 w1942 w1973 w1994 w2013 w2032 w2051 w2086 w2132 w2157 w2186 w2207 w2226 w2245 w2264 w2294 w2342 w2359 w2393 w2429 w2457 w2478 w2505 w2529 w2552 w2579 w2604 w2623 w2644 w2691 w2717 w2741 w2762 w2790 w2804 w2825 w2846 w2867 w2889 w2909 w2938 w2958 w2985 w3005 w3030 w3049 w3068 w3087 w3106 w3125 w3144] -> w1106
            tunnel: w1105 -> [_ _ _ _ _ _ _ _ _ _ w1636 _ _ _ w1756 w1766 _ _ _ _ _ _ _ _ _ _ _ _ w2129 _ _ _ _ _ _ w2292 w2341 _ _ _ _ _ _ _ w2551 _ _ _ _ w2668 _ _ _ _ _ _ _ _ _ _ _ _ _ _ _ _ _ _ _ _ _]
            tunnel: w1104 -> [_ _ _ _ _ _ _ _ _ _ w1637 _ _ _ w1755 w1765 _ _ _ _ _ _ _ _ _ _ _ _ w2128 _ _ _ _ _ _ w2293 w2340 _ _ _ _ _ _ _ w2550 _ _ _ _ w2667 _ _ _ _ _ _ _ _ _ _ _ _ _ _ _ _ _ _ _ _ _]
            tunnel: w1102 -> [_ _ _ _ _ _ _ _ _ _ _ _ _ _ _ _ w1802 _ w1845 w1874 w1910 w1936 w1969 _ _ _ _ w2070 w2115 w2153 w2182 _ _ _ _ _ _ _ _ _ _ _ _ _ _ _ _ _ _ _ _ _ _ _ _ _ _ _ _ _ _ _ _ _ _ _ _ _ _ _ _]
            tunnel: [_ _ _ _ _ _ _ _ _ _ _ _ _ _ _ _ _ _ _ w1878 w1912 w1939 w1972 _ _ _ _ TRUE w2118 w2155 _ _ _ _ _ _ _ _ _ _ _ _ _ _ _ _ _ _ _ _ _ _ _ _ _ _ _ _ _ _ _ _ _ _ _ _ _ _ _ _ _] -> w1101
            tunnel: w1100 -> [_ _ _ _ _ _ _ _ _ _ _ _ _ _ _ _ w1801 _ _ w1877 w1916 w1941 w1970 _ _ _ _ w2078 w2123 w2152 w2185 _ _ _ _ _ _ _ _ _ _ _ _ _ _ _ _ _ _ _ _ _ _ _ _ _ _ _ _ _ _ _ _ _ _ _ _ _ _ _ _]
            tunnel: w1099 -> [_ _ _ _ _ _ _ _ _ _ _ _ _ _ _ _ w1800 _ _ w1876 w1915 w1940 w1971 _ _ _ _ w2077 w2122 w2151 w2184 _ _ _ _ _ _ _ _ _ _ _ _ _ _ _ _ _ _ _ _ _ _ _ _ _ _ _ _ _ _ _ _ _ _ _ _ _ _ _ _]
            tunnel: [_ _ _ _ _ _ _ _ _ _ _ _ _ _ _ _ w1801 _ w1848 w1877 w1916 w1941 w1970 _ _ _ _ w2078 w2123 w2152 w2185 _ _ _ _ _ _ _ _ _ _ _ _ _ _ _ _ _ _ _ _ _ _ _ _ _ _ _ _ _ _ _ _ _ _ _ _ _ _ _ _] -> w1098
            tunnel: [_ _ _ _ _ _ _ _ _ _ _ _ _ _ _ _ w1800 _ w1847 w1876 w1915 w1940 w1971 _ _ _ _ w2077 w2122 w2151 w2184 _ _ _ _ _ _ _ _ _ _ _ _ _ _ _ _ _ _ _ _ _ _ _ _ _ _ _ _ _ _ _ _ _ _ _ _ _ _ _ _] -> w1097
            tunnel: [_ _ _ _ _ _ _ _ _ _ _ _ _ _ _ _ w1803 w1826 w1846 w1875 w1911 w1937 w1968 _ _ _ _ w2071 w2116 w2154 w2183 _ _ _ _ _ _ _ _ _ _ _ _ _ _ _ _ _ _ _ _ _ _ _ _ _ _ _ _ _ _ _ _ _ _ _ _ _ _ _ _] -> w1096
            tunnel: [_ _ _ _ _ _ _ _ _ _ _ _ _ _ _ _ w1802 w1827 w1845 w1874 w1910 w1936 w1969 _ _ _ _ w2070 w2115 w2153 w2182 _ _ _ _ _ _ _ _ _ _ _ _ _ _ _ _ _ _ _ _ _ _ _ _ _ _ _ _ _ _ _ _ _ _ _ _ _ _ _ _] -> w1095
            tunnel: [_ _ _ _ _ _ _ _ _ _ _ _ _ _ _ _ _ _ _ _ w1909 _ _ _ _ _ _ _ w2120 _ _ _ _ _ _ _ _ _ _ _ _ _ _ _ _ _ _ _ _ _ _ _ _ _ _ _ _ _ _ _ _ _ _ _ _ _ _ _ _ _ _] -> w1092
            tunnel: [_ _ _ _ _ _ _ _ _ _ _ _ _ _ _ _ _ _ _ _ w1908 _ _ _ _ _ _ _ w2121 _ _ _ _ _ _ _ _ _ _ _ _ _ _ _ _ _ _ _ _ _ _ _ _ _ _ _ _ _ _ _ _ _ _ _ _ _ _ _ _ _ _] -> w1094
            tunnel: w1089 -> [_ _ _ _ _ _ _ _ _ _ _ _ _ _ _ _ _ _ _ w1873 w1907 w1938 w1967 _ _ _ _ w2073 w2117 w2156 _ _ _ _ _ _ _ _ _ _ _ _ _ _ _ _ _ _ _ _ _ _ _ _ _ _ _ _ _ _ _ _ _ _ _ _ _ _ _ _ _]
            tunnel: [_ _ _ _ _ _ _ _ _ _ _ _ _ _ _ _ _ _ _ w1873 w1907 w1938 w1967 _ _ _ _ w2073 w2119 w2156 _ _ _ _ _ _ _ _ _ _ _ _ _ _ _ _ _ _ _ _ _ _ _ _ _ _ _ _ _ _ _ _ _ _ _ _ _ _ _ _ _] -> w1088
            frame "Start1", Default {
            }
            frame "Start2" {
            }
            frame "Start3" {
            }
            frame "saveSettings1" {
              n594 = call "myRIO_BRig_RT_dataExp_Audio_freq__L.vi"() -> ("output_Audio_freq__L"=w1280:i32)  [unwired: 11 in]
              n595 = call "myRIO_BRig_RT_dataExp_Audio_freq__R.vi"() -> ("output_Audio_freq__R"=w1279:i32)  [unwired: 11 in]
              n596 = call "myRIO_BRig_RT_dataExp_Audio_amp__L.vi"() -> ("output_Audio_amp__L"=w1278:i32)  [unwired: 11 in]
              n597 = call "myRIO_BRig_RT_dataExp_Audio_amp__R.vi"() -> ("output_Audio_amp__R"=w1276:i32)  [unwired: 11 in]
              n598 = call "myRIO_BRig_RT_dataExp_TPB_min__L.vi"() -> ("output_TPB_min__L"=w1288:i32)  [unwired: 11 in]
              n599 = call "myRIO_BRig_RT_dataExp_TPB_min__R.vi"() -> ("output_TPB_min__R"=w1286:i32)  [unwired: 11 in]
              n600 = call "myRIO_BRig_RT_dataExp_TPB_max__L.vi"() -> ("output_TPB_max__L"=w1284:i32)  [unwired: 11 in]
              n601 = call "myRIO_BRig_RT_dataExp_TPB_max__R.vi"() -> ("output_TPB_max__R"=w1282:i32)  [unwired: 11 in]
              n602 = call "myRIO_BRig_RT_dataExp_ItrialUntilReward.vi"() -> ("output_I_trialUntilReward"=w1301:i32)  [unwired: 11 in]
              n603 = call "myRIO_BRig_RT_dataExp_IblockUntilReward.vi"() -> ("output_I_blockUntilReward"=w1297:i32)  [unwired: 11 in]
              n604 = call "myRIO_BRig_RT_dataExp_CueCycles.vi"() -> ("output_CueCycles"=w1296:i32)  [unwired: 11 in]
              n605 = call "myRIO_BRig_RT_dataExp_ENL_min.vi"() -> ("output_ENL_min"=w1294:i32)  [unwired: 11 in]
              n606 = call "myRIO_BRig_RT_dataExp_ENL_max.vi"() -> ("output_ENL_max"=w1292:i32)  [unwired: 11 in]
              n607 = call "myRIO_BRig_RT_dataExp_ENL_penalty.vi"() -> ("output_ENL_penalty"=w1290:i32)  [unwired: 11 in]
              n608 = local read "Audio_Freq__L"() -> (w1254:u8)
              n609 = local read "Audio_Freq__R"() -> (w1252:u8)
              n610 = local read "Audio_Amp__L"() -> (w1277:u16)
              n611 = local read "TpB_Min_L"() -> (w1287:u16)
              n612 = local read "TpB_Min_R"() -> (w1285:u16)
              n613 = local read "TpB_Max_L"() -> (w1283:u16)
              n614 = local read "TpB_Max_R"() -> (w1281:u16)
              n615 = local read "Audio_Amp__R"() -> (w1275:u16)
              n616 = local read "TrialUntilReward"() -> (w1300:bool)
              n617 = local read "CueCycles"() -> (w1295:u16)
              n618 = local read "Tcycle_ENL_min"() -> (w1293:u16)
              n619 = local read "Tcycle_ENL_max"() -> (w1291:u16)
              n620 = local read "Tcycle_ENLPenalty"() -> (w1289:u16)
              n621 = To Unsigned Word Integer(number=w1252) -> (unsigned 16bit integer=w1251:u16)
              n622 = To Unsigned Word Integer(number=w1254) -> (unsigned 16bit integer=w1253:u16)
              n623 = Boolean To (0,1)(Boolean=w1300) -> (0, 1=w1299:i16)
              n624 = To Unsigned Word Integer(number=w1299) -> (unsigned 16bit integer=w1298:u16)
              n625 = local read "BUR_min"() -> (w1269:u16)
              n626 = local read "BUR_max"() -> (w1270:u16)
              n627 = Not Equal To 0?(x=w1269) -> (x != 0?=w1268:bool)
              n628 = Not Equal To 0?(x=w1270) -> (x != 0?=w1267:bool)
              n629 = And(x=w1268, y=w1267) -> (x .and. y?=w1266:bool)
              n630 = Boolean To (0,1)(Boolean=w1266) -> (0, 1=w1271:i16)
              n631 = To Unsigned Word Integer(number=w1271) -> (unsigned 16bit integer=w1265:u16)
              n632 = Replace Array Subset(array=w1303, new element #1=w1298, index #1=w1301, new element #2=w1265, index #2=w1297, new element #3=w1295, index #3=w1296, new element #4=w1293, index #4=w1294, new element #5=w1291, index #5=w1292, new element #6=w1289, index #6=w1290, new element #7=w1287, index #7=w1288, new element #8=w1285, index #8=w1286, new element #9=w1283, index #9=w1284, new element #10=w1281, index #10=w1282, new element #11=w1253, index #11=w1280, new element #12=w1251, index #12=w1279, new element #13=w1277, index #13=w1278, new element #14=w1275, index #14=w1276) -> (w1302:u16[])
            }
            frame "saveSettings2" {
              n633 = call "myRIO_BRig_RT_dataExp_Tcycle_RewardPost.vi"() -> ("output_Tcycle_RewardPost"=w1340:i32)  [unwired: 11 in]
              n634 = call "myRIO_BRig_RT_dataExp_Tcycle_Wrong.vi"() -> ("output_Tcycle_Wrong"=w1338:i32)  [unwired: 11 in]
              n635 = call "myRIO_BRig_RT_dataExp_Tcycle_Timeout.vi"() -> ("output_Tcycle_Timeout"=w1336:i32)  [unwired: 11 in]
              n636 = call "myRIO_BRig_RT_dataExp_Tcycle_Cue_min.vi"() -> ("output_Tcycle_Cue_min"=w1334:i32)  [unwired: 11 in]
              n637 = call "myRIO_BRig_RT_dataExp_Tcycle_Cue_max.vi"() -> ("output_Tcycle_Cue_max"=w1333:i32)  [unwired: 11 in]
              n638 = call "myRIO_BRig_RT_dataExp_Tcycle_CuePenalty.vi"() -> ("output_Tcycle_CuePenalty"=w1332:i32)  [unwired: 11 in]
              n639 = call "myRIO_BRig_RT_dataExp_SolenoidProbability_L.vi"() -> ("output_SolenoidProbability_L"=w1312:i32)  [unwired: 11 in]
              n640 = call "myRIO_BRig_RT_dataExp_SolenoidProbability_R.vi"() -> ("output_SolenoidProbability_R"=w1311:i32)  [unwired: 11 in]
              n641 = call "myRIO_BRig_RT_dataExp_nBlock.vi"() -> ("output_nBlock"=w1349:i32)  [unwired: 11 in]
              n642 = call "myRIO_BRig_RT_dataExp_nTrial.vi"() -> ("output_nTrial"=w1348:i32)  [unwired: 11 in]
              n643 = call "myRIO_BRig_RT_dataExp_runTime_seconds.vi"() -> ("output_RunTime_minutes"=w1347:i32)  [unwired: 11 in]
              n644 = call "myRIO_BRig_RT_dataExp_Tcycle_Selection.vi"() -> ("output_Tcycle_Selection"=w1346:i32)  [unwired: 11 in]
              n645 = call "myRIO_BRig_RT_dataExp_Tcycle_Reward__L.vi"() -> ("output_Tcycle_Reward__L"=w1344:i32)  [unwired: 11 in]
              n646 = call "myRIO_BRig_RT_dataExp_Tcycle_Reward__R.vi"() -> ("output_Tcycle_Reward__R"=w1342:i32)  [unwired: 11 in]
              n647 = local read "Tcycle_RewardPost"() -> (w1339:u16)
              n648 = local read "Tcycle_Wrong"() -> (w1337:u16)
              n649 = local read "Tcycle_Timeout"() -> (w1335:u16)
              n650 = local read "Tcycle_CuePenalty"() -> (w1325:u16)
              n651 = local read "Tcycle_Cue_max"() -> (w1313:u16)
              n652 = local read "Tcycle_Cue_min"() -> (w1314:u16)
              n653 = local read "Tcycle_Selection"() -> (w1345:u16)
              n654 = local read "Tcycle_Reward_L"() -> (w1343:u16)
              n655 = local read "Tcycle_Reward_R"() -> (w1341:u16)
              n656 = local read "SolenoidProbability_R"() -> (w1309:u16)
              n657 = local read "SolenoidProbability_L"() -> (w1310:u16)
              n658 = Replace Array Subset(array=w1351, new element #1=u16 0, index #1=w1349, new element #2=u16 0, index #2=w1348, new element #3=u16 0, index #3=w1347, new element #4=w1345, index #4=w1346, new element #5=w1343, index #5=w1344, new element #6=w1341, index #6=w1342, new element #7=w1339, index #7=w1340, new element #8=w1337, index #8=w1338, new element #9=w1335, index #9=w1336, new element #10=w1314, index #10=w1334, new element #11=w1313, index #11=w1333, new element #12=w1325, index #12=w1332, new element #13=w1310, index #13=w1312, new element #14=w1309, index #14=w1311) -> (w1350:u16[])
            }
            frame "saveSettings3" {
              w1361 = 100.0 ("y")
              n659 = call "myRIO_BRig_RT_dataExp_laser_Freq.vi"() -> ("output_laser_Freq"=w1394:i32)  [unwired: 11 in]
              n660 = call "myRIO_BRig_RT_dataExp_laser_Tpeak.vi"() -> ("output_laser_Tpeak"=w1389:i32)  [unwired: 11 in]
              n661 = call "myRIO_BRig_RT_dataExp_laser_Tshutter.vi"() -> ("output_laser_Tshutter"=w1384:i32)  [unwired: 11 in]
              n662 = call "myRIO_BRig_RT_dataExp_laser_f_millisec2count.vi"() -> ("output_laser_f_millisec2count"=w1379:i32)  [unwired: 11 in]
              n663 = call "myRIO_BRig_RT_dataExp_laser_Power_min.vi"() -> ("output_laser_Power_min"=w1374:i32)  [unwired: 11 in]
              n664 = call "myRIO_BRig_RT_dataExp_laser_Power_max.vi"() -> ("output_laser_Power_max"=w1367:i32)  [unwired: 11 in]
              n665 = call "myRIO_BRig_RT_dataExp_laser_Power_step.vi"() -> ("output_laser_Power_step"=w1366:i32)  [unwired: 11 in]
              n666 = call "myRIO_BRig_RT_dataExp_laser_duration.vi"() -> ("output_laser_duration"=w1369:i32)  [unwired: 11 in]
              n667 = call "myRIO_BRig_RT_dataExp_BUR_min.vi"() -> ("output_BUR_min"=w1416:i32)  [unwired: 11 in]
              n668 = call "myRIO_BRig_RT_dataExp_BUR_max.vi"() -> ("output_BUR_max"=w1414:i32)  [unwired: 11 in]
              n669 = call "myRIO_BRig_RT_dataExp_Audio_sp__L.vi"() -> ("output_Audio_sp__L"=w1411:i32)  [unwired: 11 in]
              n670 = call "myRIO_BRig_RT_dataExp_Audio_sp__R.vi"() -> ("output_Audio_sp__R"=w1410:i32)  [unwired: 11 in]
              n671 = local read "laser_Tshutter"() -> (w1381:dbl)
              n672 = local read "f_millisec2count"() -> (w1376:dbl)
              n673 = local read "laser_Tpeak"() -> (w1386:dbl)
              n674 = local read "laser_power_min"() -> (w1371:dbl)
              n675 = local read "laser_power_max"() -> (w1360:dbl)
              n676 = local read "laser_power_step"() -> (w1359:dbl)
              n677 = local read "laser_Freq"() -> (w1393:dbl)
              n678 = local read "sp_LeftSpout"() -> (w1409:u16)
              n679 = local read "BUR_max"() -> (w1413:u16)
              n680 = local read "sp_RightSpout"() -> (w1408:u16)
              n681 = local read "BUR_min"() -> (w1415:u16)
              n682 = Multiply(x=w1393, y=w1361) -> (x*y=w1392:dbl)
              n683 = Multiply(x=w1386, y=w1361) -> (x*y=w1388:dbl)
              n684 = Multiply(x=w1381, y=w1361) -> (x*y=w1383:dbl)
              n685 = Multiply(x=w1376, y=w1361) -> (x*y=w1378:dbl)
              n686 = Multiply(x=w1371, y=w1361) -> (x*y=w1373:dbl)
              n687 = Multiply(x=w1360, y=w1361) -> (x*y=w1365:dbl)
              n688 = Multiply(x=w1359, y=w1361) -> (x*y=w1363:dbl)
              n689 = Round To Nearest(number=w1392) -> (nearest integer value=w1391:dbl)
              n690 = Round To Nearest(number=w1388) -> (nearest integer value=w1387:dbl)
              n691 = Round To Nearest(number=w1383) -> (nearest integer value=w1382:dbl)
              n692 = Round To Nearest(number=w1378) -> (nearest integer value=w1377:dbl)
              n693 = Round To Nearest(number=w1373) -> (nearest integer value=w1372:dbl)
              n694 = Round To Nearest(number=w1365) -> (nearest integer value=w1364:dbl)
              n695 = Round To Nearest(number=w1363) -> (nearest integer value=w1362:dbl)
              n696 = To Unsigned Word Integer(number=w1391) -> (unsigned 16bit integer=w1390:u16)
              n697 = To Unsigned Word Integer(number=w1387) -> (unsigned 16bit integer=w1385:u16)
              n698 = To Unsigned Word Integer(number=w1382) -> (unsigned 16bit integer=w1380:u16)
              n699 = To Unsigned Word Integer(number=w1377) -> (unsigned 16bit integer=w1375:u16)
              n700 = To Unsigned Word Integer(number=w1372) -> (unsigned 16bit integer=w1370:u16)
              n701 = To Unsigned Word Integer(number=w1364) -> (unsigned 16bit integer=w1358:u16)
              n702 = To Unsigned Word Integer(number=w1362) -> (unsigned 16bit integer=w1357:u16)
              n703 = local read "laser_duration"() -> (w1368:u16)
              n704 = call "myRIO_BRig_RT_dataCurrent_LaserPulse_duration.vi"() -> ("output_LaserPulse_duration"=w1395:i32)  [unwired: 11 in]
              n705 = Replace Array Subset(array=w1417, new element #1=w1415, index #1=w1416, new element #2=w1413, index #2=w1414, new element #3=w1409, index #3=w1411, new element #4=w1408, index #4=w1410, new element #5=w1390, index #5=w1394, new element #6=w1385, index #6=w1389, new element #7=w1380, index #7=w1384, new element #8=w1375, index #8=w1379, new element #9=w1370, index #9=w1374, new element #10=w1358, index #10=w1367, new element #11=w1357, index #11=w1366, new element #12=w1368, index #12=w1369) -> (w1412:u16[])
              n706 = Replace Array Subset(array=w1397, new element=w1368, index=w1395) -> (w1396:u16[])
            }
            frame "saveSettings4_LC_ENL" {
              # "delayOpt"
              # "Count"
              # "Tdelay"
              # "Probability"
              # "OnOff"
              # "Block"
              # "ENL1 All"
              # "delayOpt"
              # "Count"
              # "Tdelay"
              # "Probability"
              # "OnOff"
              # "Block"
              # "ENL1 First"
              n707 = call "myRIO_BRig_RT_dataLC_ENL1_All_Block.vi"() -> ("output_ENL1_All_Block"=w1440:i32)  [unwired: 11 in]
              n708 = call "myRIO_BRig_RT_dataLC_ENL1_All_OnOff.vi"() -> ("output_ENL1_All_OnOff"=w1429:i32)  [unwired: 11 in]
              n709 = call "myRIO_BRig_RT_dataLC_ENL1_All_Probability.vi"() -> ("output_ENL1_All_Probability"=w1428:i32)  [unwired: 11 in]
              n710 = call "myRIO_BRig_RT_dataLC_ENL1_All_Tdelay.vi"() -> ("output_ENL1_All_Tdelay"=w1427:i32)  [unwired: 11 in]
              n711 = call "myRIO_BRig_RT_dataLC_ENL1_All_Count.vi"() -> ("output_ENL1_All_Count"=w1426:i32)  [unwired: 11 in]
              n712 = call "myRIO_BRig_RT_dataLC_ENL1_All_delayOpt.vi"() -> ("output_ENL1_All_delayOpt"=w1425:i32)  [unwired: 11 in]
              n713 = call "myRIO_BRig_RT_dataLC_ENL1_First_Block.vi"() -> ("output_ENL1_First_Block"=w1466:i32)  [unwired: 11 in]
              n714 = call "myRIO_BRig_RT_dataLC_ENL1_First_OnOff.vi"() -> ("output_ENL1_First_OnOff"=w1464:i32)  [unwired: 11 in]
              n715 = call "myRIO_BRig_RT_dataLC_ENL1_First_Probability.vi"() -> ("output_ENL1_First_Probability"=w1460:i32)  [unwired: 11 in]
              n716 = call "myRIO_BRig_RT_dataLC_ENL1_First_Tdelay.vi"() -> ("output_ENL1_First_Tdelay"=w1458:i32)  [unwired: 11 in]
              n717 = call "myRIO_BRig_RT_dataLC_ENL1_First_Count.vi"() -> ("output_ENL1_First_Count"=w1456:i32)  [unwired: 11 in]
              n718 = call "myRIO_BRig_RT_dataLC_ENL1_First_delayOpt.vi"() -> ("output_ENL1_First_delayOpt"=w1442:i32)  [unwired: 11 in]
              n719 = local read "LC_ENL1_First_delayOpt"() -> (w1443:bool)
              n720 = local read "LC_ENL1_First_Count"() -> (w1455:u16)
              n721 = local read "LC_ENL1_First_Probability"() -> (w1459:u16)
              n722 = local read "LC_ENL1_First_Block"() -> (w1465:u16)
              n723 = local read "LC_ENL1_First_Tdelay"() -> (w1457:u16)
              n724 = local read "LC_ENL1_First_OnOff"() -> (w1463:bool)
              n725 = local read "LC_ENL1_All_OnOff"() -> (w1436:bool)
              n726 = local read "LC_ENL1_All_Probability"() -> (w1434:u16)
              n727 = local read "LC_ENL1_All_delayOpt"() -> (w1431:bool)
              n728 = local read "LC_ENL1_All_Tdelay"() -> (w1433:u16)
              n729 = local read "LC_ENL1_All_Block"() -> (w1437:u16)
              n730 = local read "LC_ENL1_All_Count"() -> (w1432:u16)
              n731 = Boolean To (0,1)(Boolean=w1443) -> (0, 1=w1444:i16)
              n732 = Boolean To (0,1)(Boolean=w1463) -> (0, 1=w1462:i16)
              n733 = Boolean To (0,1)(Boolean=w1436) -> (0, 1=w1439:i16)
              n734 = To Unsigned Word Integer(number=w1444) -> (unsigned 16bit integer=w1441:u16)
              n735 = To Unsigned Word Integer(number=w1462) -> (unsigned 16bit integer=w1461:u16)
              n736 = Boolean To (0,1)(Boolean=w1431) -> (0, 1=w1438:i16)
              n737 = To Unsigned Word Integer(number=w1439) -> (unsigned 16bit integer=w1435:u16)
              n738 = To Unsigned Word Integer(number=w1438) -> (unsigned 16bit integer=w1430:u16)
              n739 = Replace Array Subset(array=w1467, new element #1=w1465, index #1=w1466, new element #2=w1461, index #2=w1464, new element #3=w1459, index #3=w1460, new element #4=w1457, index #4=w1458, new element #5=w1455, index #5=w1456, new element #6=w1441, index #6=w1442, new element #7=w1437, index #7=w1440, new element #8=w1435, index #8=w1429, new element #9=w1434, index #9=w1428, new element #10=w1433, index #10=w1427, new element #11=w1432, index #11=w1426, new element #12=w1430, index #12=w1425) -> (w1468:u16[])
            }
            frame "saveSettings5_LC_Cue" {
              # "delayOpt"
              # "Count"
              # "Tdelay"
              # "Probability"
              # "OnOff"
              # "Block"
              # "Cue1 All"
              # "delayOpt"
              # "Count"
              # "Tdelay"
              # "Probability"
              # "OnOff"
              # "Block"
              # "Cue1 First"
              n740 = call "myRIO_BRig_RT_dataLC_Cue1_First_delayOpt.vi"() -> ("output_Cue1_First_delayOpt"=w1495:i32)  [unwired: 11 in]
              n741 = call "myRIO_BRig_RT_dataLC_Cue1_First_Block.vi"() -> ("output_Cue1_First_Block"=w1518:i32)  [unwired: 11 in]
              n742 = call "myRIO_BRig_RT_dataLC_Cue1_First_OnOff.vi"() -> ("output_Cue1_First_OnOff"=w1516:i32)  [unwired: 11 in]
              n743 = call "myRIO_BRig_RT_dataLC_Cue1_First_Probability.vi"() -> ("output_Cue1_First_Probability"=w1512:i32)  [unwired: 11 in]
              n744 = call "myRIO_BRig_RT_dataLC_Cue1_First_Tdelay.vi"() -> ("output_Cue1_First_Tdelay"=w1510:i32)  [unwired: 11 in]
              n745 = call "myRIO_BRig_RT_dataLC_Cue1_First_Count.vi"() -> ("output_Cue1_First_Count"=w1508:i32)  [unwired: 11 in]
              n746 = call "myRIO_BRig_RT_dataLC_Cue1_All_Block.vi"() -> ("output_Cue1_All_Block"=w1492:i32)  [unwired: 11 in]
              n747 = call "myRIO_BRig_RT_dataLC_Cue1_All_OnOff.vi"() -> ("output_Cue1_All_OnOff"=w1491:i32)  [unwired: 11 in]
              n748 = call "myRIO_BRig_RT_dataLC_Cue1_All_Probability.vi"() -> ("output_Cue1_All_Probability"=w1490:i32)  [unwired: 11 in]
              n749 = call "myRIO_BRig_RT_dataLC_Cue1_All_Tdelay.vi"() -> ("output_Cue1_All_Tdelay"=w1489:i32)  [unwired: 11 in]
              n750 = call "myRIO_BRig_RT_dataLC_Cue1_All_Count.vi"() -> ("output_Cue1_All_Count"=w1488:i32)  [unwired: 11 in]
              n751 = call "myRIO_BRig_RT_dataLC_Cue1_All_delayOpt.vi"() -> ("output_Cue1_All_delayOpt"=w1487:i32)  [unwired: 11 in]
              n752 = local read "LC_Cue1_First_delayOpt"() -> (w1494:bool)
              n753 = local read "LC_Cue1_First_Count"() -> (w1507:u16)
              n754 = local read "LC_Cue1_First_Probability"() -> (w1511:u16)
              n755 = local read "LC_Cue1_First_Block"() -> (w1517:u16)
              n756 = local read "LC_Cue1_First_Tdelay"() -> (w1509:u16)
              n757 = local read "LC_Cue1_First_OnOff"() -> (w1515:bool)
              n758 = local read "LC_Cue1_All_OnOff"() -> (w1483:bool)
              n759 = local read "LC_Cue1_All_delayOpt"() -> (w1484:bool)
              n760 = local read "LC_Cue1_All_Probability"() -> (w1480:u16)
              n761 = local read "LC_Cue1_All_Tdelay"() -> (w1479:u16)
              n762 = local read "LC_Cue1_All_Count"() -> (w1478:u16)
              n763 = local read "LC_Cue1_All_Block"() -> (w1482:u16)
              n764 = Boolean To (0,1)(Boolean=w1494) -> (0, 1=w1496:i16)
              n765 = Boolean To (0,1)(Boolean=w1515) -> (0, 1=w1514:i16)
              n766 = Boolean To (0,1)(Boolean=w1483) -> (0, 1=w1486:i16)
              n767 = To Unsigned Word Integer(number=w1496) -> (unsigned 16bit integer=w1493:u16)
              n768 = To Unsigned Word Integer(number=w1514) -> (unsigned 16bit integer=w1513:u16)
              n769 = To Unsigned Word Integer(number=w1486) -> (unsigned 16bit integer=w1481:u16)
              n770 = Boolean To (0,1)(Boolean=w1484) -> (0, 1=w1485:i16)
              n771 = To Unsigned Word Integer(number=w1485) -> (unsigned 16bit integer=w1477:u16)
              n772 = Replace Array Subset(array=w1519, new element #1=w1517, index #1=w1518, new element #2=w1513, index #2=w1516, new element #3=w1511, index #3=w1512, new element #4=w1509, index #4=w1510, new element #5=w1507, index #5=w1508, new element #6=w1493, index #6=w1495, new element #7=w1482, index #7=w1492, new element #8=w1481, index #8=w1491, new element #9=w1480, index #9=w1490, new element #10=w1479, index #10=w1489, new element #11=w1478, index #11=w1488, new element #12=w1477, index #12=w1487) -> (w1520:u16[])
            }
            frame "saveSettings6_LC_Other" {
              # "Trial"
              # "Tdelay"
              # "Probability"
              # "OnOff"
              # "Block"
              # "Wrong"
              # "Trial"
              # "Tdelay"
              # "Probability"
              # "OnOff"
              # "Block"
              # "Reward"
              n773 = call "myRIO_BRig_RT_dataLC_Wrong_Block.vi"() -> ("output_Wrong_Block"=w1550:i32)  [unwired: 11 in]
              n774 = call "myRIO_BRig_RT_dataLC_Wrong_OnOff.vi"() -> ("output_Wrong_OnOff"=w1549:i32)  [unwired: 11 in]
              n775 = call "myRIO_BRig_RT_dataLC_Wrong_Probability.vi"() -> ("output_Wrong_Probability"=w1548:i32)  [unwired: 11 in]
              n776 = call "myRIO_BRig_RT_dataLC_Wrong_Tdelay.vi"() -> ("output_Wrong_Tdelay"=w1547:i32)  [unwired: 11 in]
              n777 = call "myRIO_BRig_RT_dataLC_Wrong_Trial.vi"() -> ("output_Wrong_Trial"=w1546:i32)  [unwired: 11 in]
              n778 = call "myRIO_BRig_RT_dataLC_Reward_Block.vi"() -> ("output_Reward_Block"=w1562:i32)  [unwired: 11 in]
              n779 = call "myRIO_BRig_RT_dataLC_Reward_OnOff.vi"() -> ("output_Reward_OnOff"=w1560:i32)  [unwired: 11 in]
              n780 = call "myRIO_BRig_RT_dataLC_Reward_Probability.vi"() -> ("output_Reward_Probability"=w1556:i32)  [unwired: 11 in]
              n781 = call "myRIO_BRig_RT_dataLC_Reward_Tdelay.vi"() -> ("output_Reward_Tdelay"=w1554:i32)  [unwired: 11 in]
              n782 = call "myRIO_BRig_RT_dataLC_Reward_Trial.vi"() -> ("output_Reward_Trial"=w1552:i32)  [unwired: 11 in]
              n783 = local read "LC_Wrong_OnOff"() -> (w1544:bool)
              n784 = local read "LC_Wrong_Probability"() -> (w1541:u16)
              n785 = local read "LC_Wrong_Block"() -> (w1543:u16)
              n786 = local read "LC_Wrong_Tdelay"() -> (w1540:u16)
              n787 = local read "LC_Wrong_Trial"() -> (w1539:u16)
              n788 = local read "LC_Reward_Probability"() -> (w1555:u16)
              n789 = local read "LC_Reward_Block"() -> (w1561:u16)
              n790 = local read "LC_Reward_Tdelay"() -> (w1553:u16)
              n791 = local read "LC_Reward_OnOff"() -> (w1559:bool)
              n792 = local read "LC_Reward_Trial"() -> (w1551:u16)
              n793 = Boolean To (0,1)(Boolean=w1544) -> (0, 1=w1545:i16)
              n794 = Boolean To (0,1)(Boolean=w1559) -> (0, 1=w1558:i16)
              n795 = To Unsigned Word Integer(number=w1545) -> (unsigned 16bit integer=w1542:u16)
              n796 = To Unsigned Word Integer(number=w1558) -> (unsigned 16bit integer=w1557:u16)
              n797 = Replace Array Subset(array=w1563, new element #1=w1561, index #1=w1562, new element #2=w1557, index #2=w1560, new element #3=w1555, index #3=w1556, new element #4=w1553, index #4=w1554, new element #5=w1551, index #5=w1552, new element #6=w1543, index #6=w1550, new element #7=w1542, index #7=w1549, new element #8=w1541, index #8=w1548, new element #9=w1540, index #9=w1547, new element #10=w1539, index #10=w1546) -> (w1564:u16[])
            }
            frame "setSettings_Audio" {
              # "amp_L"
              # "amp_R"
              # "freq_L"
              # "freq_R"
              n798 = call "myRIO_BRig_RT_dataExp_Audio_amp__L.vi"() -> ("output_Audio_amp__L"=w1589:i32)  [unwired: 11 in]
              n799 = call "myRIO_BRig_RT_dataExp_Audio_amp__R.vi"() -> ("output_Audio_amp__R"=w1588:i32)  [unwired: 11 in]
              n800 = call "myRIO_BRig_RT_dataExp_Audio_freq__L.vi"() -> ("output_Audio_freq__L"=w1587:i32)  [unwired: 11 in]
              n801 = call "myRIO_BRig_RT_dataExp_Audio_freq__R.vi"() -> ("output_Audio_freq__R"=w1586:i32)  [unwired: 11 in]
              n802 = Index Array(array=w1585, index #1=w1589, index #2=w1588, index #3=w1587, index #4=w1586) -> (element #1=w1584:u16, element #2=w1583:u16, element #3=w1576:u16, element #4=w1574:u16)
              n803 = To Unsigned Byte Integer(number=w1576) -> (unsigned 8bit integer=w1575:u8)
              n804 = To Unsigned Byte Integer(number=w1574) -> (unsigned 8bit integer=w1573:u8)
            }
            frame "setSettings_Laser" {
              (unwired) u32 0 ("tDelay_laser_rew")
              # "Wrong tDelay"
              # "Reward tDelay"
              n805 = call "myRIO_BRig_RT_dataLC_Reward_Tdelay.vi"() -> ("output_Reward_Tdelay"=w1616:i32)  [unwired: 11 in]
              n806 = call "myRIO_BRig_RT_dataLC_Wrong_Tdelay.vi"() -> ("output_Wrong_Tdelay"=w1617:i32)  [unwired: 11 in]
              n807 = Index Array(array=w1613, index #1=w1616, index #2=w1617) -> (element #1=w1615:u16, element #2=w1614:u16)
              n808 = call "myRIO_BRig_RT__calc_Tvalley.vi"("input_peakWidth"="laser_Tpeak", "input_freq"="laser_Freq") -> ("output_Tvalley"=w1623:dbl)  [unwired: 9 in]
              n809 = To Double Precision Float(number=w1615) -> (double precision float=w1610:dbl)
              n810 = To Double Precision Float(number=w1614) -> (double precision float=w1607:dbl)
              n811 = Multiply(x="f_millisec2count", y="laser_Tpeak") -> (x*y=w1632:dbl)
              n812 = Multiply(x="f_millisec2count", y=w1623) -> (x*y=w1629:dbl)
              n813 = Multiply(x="f_millisec2count", y="laser_Tshutter") -> (x*y=w1627:dbl)
              n814 = Round Toward +Infinity(x="laser_Tshutter") -> (ceil(x): smallest int >= x=w1618:dbl)
              n815 = Multiply(x="f_millisec2count", y=w1610) -> (x*y=w1611:dbl)
              n816 = Multiply(x="f_millisec2count", y=w1607) -> (x*y=w1608:dbl)
              n817 = To Unsigned Word Integer(number="f_millisec2count") -> (unsigned 16bit integer=w1598:u16)
              n818 = Round Toward +Infinity(x=w1632) -> (ceil(x): smallest int >= x=w1633:dbl)
              n819 = Round Toward +Infinity(x=w1629) -> (ceil(x): smallest int >= x=w1630:dbl)
              n820 = Round Toward +Infinity(x=w1627) -> (ceil(x): smallest int >= x=w1622:dbl)
              n821 = Round Toward +Infinity(x=w1611) -> (ceil(x): smallest int >= x=w1612:dbl)
              n822 = Round Toward +Infinity(x=w1608) -> (ceil(x): smallest int >= x=w1609:dbl)
              n823 = To Unsigned Long Integer(number=w1633) -> (unsigned 32bit integer=w1631:u32)
              n824 = To Unsigned Long Integer(number=w1630) -> (unsigned 32bit integer=w1628:u32)
              n825 = To Unsigned Long Integer(number=w1622) -> (unsigned 32bit integer=w1626:u32)
              n826 = To Unsigned Word Integer(number=w1618) -> (unsigned 16bit integer=w1621:u16)
              n827 = To Unsigned Long Integer(number=w1612) -> (unsigned 32bit integer=w1606:u32)
              n828 = To Unsigned Long Integer(number=w1609) -> (unsigned 32bit integer=w1605:u32)
              n829 = Add(x="laser_duration", y=w1621) -> (x+y=w1602:u16)
              n830 = To Double Precision Float(number=w1602) -> (double precision float=w1601:dbl)
              n831 = Multiply(x=w1601, y="f_millisec2count") -> (x*y=w1603:dbl)
              n832 = call "myRIO_BRig_RT_dataCurrent_LaserPulse_duration.vi"() -> ("output_LaserPulse_duration"=w1634:i32)  [unwired: 11 in]
              n833 = Round Toward +Infinity(x=w1603) -> (ceil(x): smallest int >= x=w1604:dbl)
              n834 = To Unsigned Long Integer(number=w1604) -> (unsigned 32bit integer=w1600:u32)
              n835 = xnode "Read/Write Control"("FPGA VI Reference In"=w1636, "error in"=w1637, "laser_Npeak"=w1631, "laser_Nvalley"=w1628, "laser_Nshutter"=w1626, "laser_selRew_Ndelay"=w1606, "laser_selWro_NDelay"=w1605, "laser_selRew_Ntotal"=w1600, "laser_selWro_Ntotal"=w1600, "k1__counter_per_ms"=w1598) -> ("error out"=→"error out":errorcluster)  [unwired: 1 out]
              n836 = Replace Array Subset(array=w1613, new element=w1602, index=w1634) -> (w1635:u16[])
            }
            frame "initBlock" {
              n837 = call "myRIO_Brig_RT__Case_Exp_State_initBlock.vi"("input_spout"=w1680, "input_dataExp"=w1678, "input_dataCurrent"=w1679) -> ("output_spout"=w1657:enum16{"Left", "Right"}, "output_state"=w1681:T2, "output_dataExp"=w1677:u16[], "output_dataCurrent"=w1663:u16[], "output_TpB_target"=→"TpB_target":u16)  [unwired: 4 in]
              "cSpout" <- w1657
              n838 = call "myRIO_BRig_RT_dataCurrent_iBlock.vi"() -> ("output_iBlock"=w1662:i32)  [unwired: 11 in]
              n839 = Index Array(array=w1663, index=w1662) -> (element=→"iBlock":u16)
            }
            frame "initBlock2" {
              n840 = local write "nRewards_cur"(u16 0 ("nRewards_cur")) -> ()
              n841 = call "myRIO_BRig_RT__Case_Exp_State_initBlock2.vi"("input_spout"=w1689, "input_dataBlock"=w1690, "input_dataCurrent"=w1688) -> ("idxDataBlock"=w1685:i32, "output_dataBlock"=w1687:u16[][])  [unwired: 7 in]
            }
            frame "initTrial" {
              n842 = call "myRIO_Brig_RT__Case_Exp_State_initTrial.vi"("input_spout"=w1706, "input_dataExp"=w1723, "input_dataCurrent"=w1724) -> ("output_state"=w1725:T2, "output_dataExp"=w1722:u16[], "output_dataCurrent"=w1712:u16[])  [unwired: 6 in]
              n843 = call "myRIO_BRig_RT_dataCurrent_iTrial.vi"() -> ("output_iTrial"=w1711:i32)  [unwired: 11 in]
              n844 = call "myRIO_BRig_RT_dataCurrent_SolenoidReward.vi"() -> ("output_SolenoidReward"=w1705:i32)  [unwired: 11 in]
              n845 = Index Array(array=w1712, index #1=w1711, index #2=w1705) -> (element #1=→"iTrial":u16, element #2=w1704:u16)
              n846 = Not Equal To 0?(x=w1704) -> (x != 0?=→"SolenoidReward":bool)
            }
            frame "initTrial2" {
              # "trialUntilReward"
              n847 = call "myRIO_BRig_RT__Case_Exp_subState_LC__initTrial.vi"("input_dataTrial"=w1732, "input_spout"=w1741, "input_dataCurrent"=w1730, "input_dataLC"=w1729) -> ("output_LC_Wrong"=w1742:bool, "output_LC_led_Wrong"=w1734:bool, "output_LC_Reward"=w1743:bool, "output_LC_led_Reward"=w1733:bool, "output_dataTrial"=w1731:u16[][])  [unwired: 2 in]
              n848 = Equal?(x=w1741, y=enum16{"Left", "Right"}."Right") -> (x = y?=w1739:bool)
              n849 = call "myRIO_BRig_RT_dataExp_ItrialUntilReward.vi"() -> ("output_I_trialUntilReward"=w1737:i32)  [unwired: 11 in]
              n850 = Index Array(array=w1738, index=w1737) -> (element=w1736:u16)
              n851 = Not Equal To 0?(x=w1736) -> (x != 0?=w1735:bool)
              n852 = xnode "Read/Write Control"("FPGA VI Reference In"=w1756, "error in"=w1755, "SelectionState"=FALSE, "laserResponse_reward"=w1743, "laserResponse_wrong"=w1742, "laserResponse_reward_LED"=w1733, "laserResponse_wrong_LED"=w1734, "Left(F)_or_Right(T)"=w1739, "ignoreWrong"=w1735) -> ("error out"=→"error_initTrial":errorcluster)  [unwired: 1 out]
            }
            frame "initTrial3" {
              n853 = call "myRIO_BRig_RT__Case_Exp_State_initTrial_dataTrial.vi"("input_spout"=w1771, "input_dataCurrent"=w1772, "input_dataExp"=w1770, "input_dataTrial"=w1774) -> ("output_dataTrial"=w1773:u16[][], "output_laserPower"=w1767:u16)  [unwired: 6 in]
              n854 = To Double Precision Float(number=w1767) -> (double precision float=w1769:dbl)
              n855 = Divide(x=w1769, y=100.0 ("x")) -> (x/y=w1763:dbl)
              "output_PortA" <- w1763
              n856 = call "myRIO_Brig_RT__covert_Voltage_to_FPGAvalue.vi"("input_voltage"=w1763) -> ("output_PortC"=w1762:i16)  [unwired: 9 in, 1 out]
              n857 = xnode "Read/Write Control"("FPGA VI Reference In"=w1766, "error in"=w1765, "AnaOut_0"=w1762) -> ("error out"=→"error out 4":errorcluster)  [unwired: 1 out]
            }
            frame "initTrial4" {
              n858 = call "myRIO_BRig_RT_dataCurrent_idxDataTrial.vi"() -> ("output_idxDataTrial"=w1797:i32)  [unwired: 11 in]
              n859 = call "myRIO_BRig_RT_dataTrial_activeRecording.vi"() -> ("output_activeRecording"=w1794:i32)  [unwired: 11 in]
              n860 = Index Array(array=w1799, index=w1797) -> (element=w1796:u16)
              n861 = Boolean To (0,1)(Boolean="Recording") -> (0, 1=w1793:i16)
              n862 = To Long Integer(number=w1796) -> (32bit integer=w1795:i32)
              n863 = To Unsigned Word Integer(number=w1793) -> (unsigned 16bit integer=w1792:u16)
              n864 = Replace Array Subset(array=w1798, new element=w1792, index (row)=w1795, index (col)=w1794) -> (w1791:u16[][])
              n865 = local write "Recording_p2"("Recording") -> ()
            }
            frame "initTrial_LC_ENL1" {
              n866 = call "myRIO_BRig_RT__Case_Exp_State_initTrial_LC_ENL1__v2.vi"("input_dataTrial"=w1823, "input_spout"=w1828, "input_dataBlock"=w1821, "input_dataLC"=w1829, "input_dataCurrent"=w1825) -> ("output_LC__ENL1"=w1827:bool, "output_LC_led__ENL1"=w1826:bool, "output_dataTrial"=w1822:u16[][], "output_dataCurrent"=w1824:u16[])  [unwired: 3 in]
            }
            frame "initTrial_LC_Cue1" {
              n867 = local write "Recording_p2"(FALSE ("Recording_p2")) -> ()
              n868 = call "myRIO_BRig_RT__Case_Exp_State_initTrial_LC_Cue1__v2.vi"("input_dataTrial"=w1851, "input_spout"=w1854, "input_dataBlock"=w1849, "input_dataLC"=w1855, "input_dataCurrent"=w1853) -> ("output_LC__Cue1"=w1847:bool, "output_LC_led__Cue1"=w1848:bool, "output_dataTrial"=w1850:u16[][], "output_dataCurrent"=w1852:u16[])  [unwired: 3 in]
            }
            frame "ENL1_pre" {
              # "ENL1_n"
              # "Tcycle"
              # "counter"
              n869 = call "myRIO_BRig_RT_dataCurrent_Tcycle_generic.vi"() -> ("output_Tcycle_generic"=w1901:i32)  [unwired: 11 in]
              n870 = call "myRIO_BRig_RT_dataCurrent_count_generic.vi"() -> ("output_count_generic"=w1903:i32)  [unwired: 11 in]
              n871 = call "myRIO_BRig_RT_dataCurrent_ENL.vi"() -> ("output_ENL"=w1900:i32)  [unwired: 11 in]
              n872 = call "myRIO_BRig_RT_dataCurrent_ENL1_n.vi"() -> ("output_ENL1_n"=w1872:i32)  [unwired: 11 in]
              n873 = Index Array(array=w1894, index #1=w1900, index #2=w1872) -> (element #1=w1899:u16, element #2=w1871:u16)
              n874 = Increment(x=w1871) -> (x+1=w1870:u16)
              n875 = Replace Array Subset(array=w1894, new element #1=u16 0 ("new element/subarray"), index #1=w1903, new element #2=w1899, index #2=w1901, new element #3=w1870, index #3=w1872) -> (w1898:u16[])
              n876 = Select(t=myRIO_BRig_RT__Case_Exp_stateList."ENL1Penalty_pre" ("Enum"), s=w1882, f=myRIO_BRig_RT__Case_Exp_stateList."ENL1" ("Enum")) -> (s? t:f=w1879:T2)
            }
            frame "ENL1" {
              n877 = call "myRIO_BRig_RT__Case_Exp_State_ENL1__v2.vi"("input_LC"=w1910, "I_lick"=w1914, "input_LC_led"=w1911, "input_laserOccurred"=w1906, "input_state"=w1920, "input_dataCurrent"=w1919) -> ("output_trigger_laser_led"=w1909:bool, "output_state"=w1917:T2, "output_dataCurrent"=w1918:u16[], "output_trigger_laser"=w1908:bool)  [unwired: 2 in]
              n878 = Or(x=w1909, y=w1906) -> (x .or. y?=w1912:bool)
            }
            frame "ENL1Penalty_pre" {
              # "Tcycle"
              # "counter"
              n879 = call "myRIO_BRig_RT_dataCurrent_Tcycle_generic.vi"() -> ("output_Tcycle_generic"=w1960:i32)  [unwired: 11 in]
              n880 = call "myRIO_BRig_RT_dataCurrent_count_generic.vi"() -> ("output_count_generic"=w1962:i32)  [unwired: 11 in]
              n881 = call "myRIO_BRig_RT_dataExp_ENL_penalty.vi"() -> ("output_ENL_penalty"=w1955:i32)  [unwired: 11 in]
              n882 = Index Array(array=w1956, index=w1955) -> (element=w1959:u16)
              n883 = Replace Array Subset(array=w1957, new element #1=u16 0 ("new element/subarray"), index #1=w1962, new element #2=w1959, index #2=w1960) -> (w1958:u16[])
            }
            frame "ENL1Penalty" {
              n884 = call "myRIO_BRig_RT__Case_Exp_State_ENL1Penalty.vi"("input_state"=w1985, "input_dataCurrent"=w1989) -> ("output_state"=w1986:T2, "output_dataCurrent"=w1988:u16[])  [unwired: 8 in]
            }
            frame "ENL2_pre" {
            }
            frame "ENL2" {
            }
            frame "ENL2Penalty_pre" {
            }
            frame "ENL2Penalty" {
            }
            frame "Cue1_pre" {
              # "Cue1_n"
              # "Tcycle_Cue1"
              # "0 = L, 1 = R, 2 = both"
              # "sp_R"
              # "sp_L"
              # "Tcycle"
              # "counter"
              n885 = Equal?(x=w2100, y=enum16{"Left", "Right"}."Left") -> (x = y?=w2099:bool)
              n886 = call "myRIO_BRig_RT_dataExp_Audio_sp__L.vi"() -> ("output_Audio_sp__L"=w2098:i32)  [unwired: 11 in]
              n887 = call "myRIO_BRig_RT_dataExp_Audio_sp__R.vi"() -> ("output_Audio_sp__R"=w2097:i32)  [unwired: 11 in]
              n888 = call "myRIO_BRig_RT_dataCurrent_Tcycle_generic.vi"() -> ("output_Tcycle_generic"=w2110:i32)  [unwired: 11 in]
              n889 = call "myRIO_BRig_RT_dataCurrent_count_generic.vi"() -> ("output_count_generic"=w2112:i32)  [unwired: 11 in]
              n890 = Select(t=w2098, s=w2099, f=w2097) -> (s? t:f=w2096:i32)
              n891 = call "myRIO_BRig_RT_dataCurrent_Cue1_n.vi"() -> ("output_Cue1_n"=w2074:i32)  [unwired: 11 in]
              n892 = call "myRIO_BRig_RT_dataCurrent_Tcycle_cue.vi"() -> ("output_Tcycle_cue"=w2083:i32)  [unwired: 11 in]
              n893 = Index Array(array=w2102, index=w2096) -> (element=w2094:u16)
              n894 = Index Array(array=w2084, index #1=w2083, index #2=w2074) -> (element #1=w2085:u16, element #2=w2076:u16)
              n895 = Increment(x=w2076) -> (x+1=w2075:u16)
              n896 = Not Equal To 0?(x=w2094) -> (x != 0?=w2092:bool)
              n897 = Not Equal?(x=w2094, y=u16 1) -> (x != y?=w2093:bool)
              n898 = Replace Array Subset(array=w2084, new element #1=u16 0 ("new element/subarray"), index #1=w2112, new element #2=w2085, index #2=w2110, new element #3=w2075, index #3=w2074) -> (w2109:u16[])
              n899 = Select(t=myRIO_BRig_RT__Case_Exp_stateList."Cue1Penalty_pre" ("Enum"), s=w2080, f=myRIO_BRig_RT__Case_Exp_stateList."Cue1" ("Enum")) -> (s? t:f=w2081:T2)
            }
            frame "Cue1" {
              n900 = call "myRIO_BRig_RT__Case_Exp_State_Cue1__v2.vi"("input_LC"=w2122, "I_lick"=w2125, "input_LC_led"=w2123, "input_laserOccurred"=w2117, "input_state"=w2127, "input_dataCurrent"=w2145) -> ("output_trigger_laser_led"=w2120:bool, "output_state"=w2126:T2, "output_dataCurrent"=w2144:u16[], "output_trigger_laser"=w2121:bool)  [unwired: 2 in]
              n901 = Or(x=w2120, y=w2117) -> (x .or. y?=w2119:bool)
              n902 = Equal?(x=myRIO_BRig_RT__Case_Exp_stateList."Selection_pre", y=w2126) -> (x = y?=w2130:bool)
              n903 = xnode "Read/Write Control"("FPGA VI Reference In"=w2129, "error in"=w2128, "SelectionState"=w2130) -> ()  [unwired: 2 out]
            }
            frame "Cue1Penalty_pre" {
              # "Tcycle"
              # "counter"
              n904 = call "myRIO_BRig_RT_dataCurrent_Tcycle_generic.vi"() -> ("output_Tcycle_generic"=w2176:i32)  [unwired: 11 in]
              n905 = call "myRIO_BRig_RT_dataCurrent_count_generic.vi"() -> ("output_count_generic"=w2178:i32)  [unwired: 11 in]
              n906 = call "myRIO_BRig_RT_dataExp_Tcycle_CuePenalty.vi"() -> ("output_Tcycle_CuePenalty"=w2175:i32)  [unwired: 11 in]
              n907 = Index Array(array=w2170, index=w2175) -> (element=w2174:u16)
              n908 = Replace Array Subset(array=w2172, new element #1=u16 0 ("new element/subarray"), index #1=w2178, new element #2=w2174, index #2=w2176) -> (w2171:u16[])
            }
            frame "Cue1Penalty" {
              # "reset laserOccurred"
              n909 = call "myRIO_BRig_RT__Case_Exp_State_Cue1Penalty.vi"("input_state"=w2202, "input_dataCurrent"=w2203) -> ("output_state"=w2200:T2, "output_dataCurrent"=w2201:u16[])  [unwired: 8 in]
            }
            frame "Cue2_pre" {
              n910 = call "myRIO_BRig_RT__Case_Exp_subState_LC__Cue2.vi"("input_spout"=w2220, "input_dataCurrent"=w2221, "input_dataLC"=w2219) -> ()  [unwired: 6 in, 2 out]
            }
            frame "Cue2" {
            }
            frame "Cue2Penalty_pre" {
            }
            frame "Cue2Penalty" {
            }
            frame "Selection_pre" {
              # "Tcycle"
              # "counter"
              n911 = xnode "Read/Write Control"("FPGA VI Reference In"=w2292, "error in"=w2293) -> ("error out"=→"error_Selection_pre":errorcluster, "SelectReward"=w2285:bool, "SelectWrong"=w2287:bool)  [unwired: 1 out]
              n912 = call "myRIO_BRig_RT_dataCurrent_Tcycle_generic.vi"() -> ("output_Tcycle_generic"=w2314:i32)  [unwired: 11 in]
              n913 = call "myRIO_BRig_RT_dataCurrent_count_generic.vi"() -> ("output_count_generic"=w2316:i32)  [unwired: 11 in]
              n914 = call "myRIO_BRig_RT_dataExp_Tcycle_Selection.vi"() -> ("output_Tcycle_Selection"=w2313:i32)  [unwired: 11 in]
              n915 = Index Array(array=w2310, index=w2313) -> (element=w2312:u16)
              n916 = Replace Array Subset(array=w2308, new element #1=u16 0 ("new element/subarray"), index #1=w2316, new element #2=w2312, index #2=w2314) -> (w2311:u16[])
              n917 = Or(x=w2285, y=w2287) -> (x .or. y?=w2286:bool)
              n918 = Select(t=myRIO_BRig_RT__Case_Exp_stateList."SelectReward_pre" ("Enum"), s=w2285, f=myRIO_BRig_RT__Case_Exp_stateList."SelectWrong_pre" ("Enum")) -> (s? t:f=w2291:T2)
              n919 = Select(t=w2291, s=w2286, f=myRIO_BRig_RT__Case_Exp_stateList."Selection" ("Enum")) -> (s? t:f=w2288:T2)
            }
            frame "Selection" {
              # "counter\nSelection"
              # "increment"
              # "get Tcycle"
              # "get count"
              n920 = xnode "Read/Write Control"("FPGA VI Reference In"=w2341, "error in"=w2340) -> ("error out"=→"error_Selection":errorcluster, "SelectReward"=w2337:bool, "SelectWrong"=w2338:bool)  [unwired: 1 out]
              n921 = call "myRIO_BRig_RT_dataCurrent_Tcycle_generic.vi"() -> ("output_Tcycle_generic"=w2334:i32)  [unwired: 11 in]
              n922 = call "myRIO_BRig_RT_dataCurrent_count_generic.vi"() -> ("output_count_generic"=w2327:i32)  [unwired: 11 in]
              n923 = Index Array(array=w2335, index #1=w2334, index #2=w2327) -> (element #1=w2326:u16, element #2=w2333:u16)
              n924 = call "myRIO_BRig_RT__increment_u16.vi"() -> ("output_increment__u16"=w2332:u16)  [unwired: 11 in]
              n925 = Add(x=w2333, y=w2332) -> (x+y=w2328:u16)
              n926 = Greater?(x=w2326, y=w2328) -> (0:w2320:bool)
              n927 = Select(t=w2331, s=w2320, f=myRIO_BRig_RT__Case_Exp_stateList."SelectTimeout_pre" ("Enum")) -> (s? t:f=w2321:T2)
              n928 = Select(t=w2328, s=w2320, f=w2326) -> (s? t:f=w2324:u16)
              n929 = call "myRIO_BRig_RT_dataCurrent_count_selection.vi"() -> ("output_count_generic"=w2325:i32)  [unwired: 11 in]
              n930 = Select(t=myRIO_BRig_RT__Case_Exp_stateList."SelectReward_pre" ("Enum"), s=w2337, f=myRIO_BRig_RT__Case_Exp_stateList."SelectWrong_pre" ("Enum")) -> (s? t:f=w2336:T2)
              n931 = Replace Array Subset(array=w2335, new element #1=w2324, index #1=w2327, new element #2=w2324, index #2=w2325) -> (w2330:u16[])
              n932 = Or(x=w2337, y=w2338) -> (x .or. y?=w2319:bool)
              n933 = Select(t=w2336, s=w2319, f=w2321) -> (s? t:f=w2339:T2)
            }
            frame "SelectReward_pre" {
              # "iState"
              # "Tcycle\nReward"
              # "nRewTrials"
              # "Tcycle\nGeneric"
              # "counter"
              n934 = call "myRIO_BRig_RT_dataCurrent_nRewTrials.vi"() -> ("output_nRewTrials"=w2373:i32)  [unwired: 11 in]
              n935 = Equal?(x=w2382, y=enum16{"Left", "Right"}."Left") -> (x = y?=w2383:bool)
              n936 = Index Array(array=w2374, index=w2373) -> (element=w2372:u16)
              n937 = call "myRIO_BRig_RT_dataExp_Tcycle_Reward__L.vi"() -> ("output_Tcycle_Reward__L"=w2386:i32)  [unwired: 11 in]
              n938 = call "myRIO_BRig_RT_dataExp_Tcycle_Reward__R.vi"() -> ("output_Tcycle_Reward__R"=w2387:i32)  [unwired: 11 in]
              n939 = Increment(x=w2372) -> (x+1=w2371:u16)
              n940 = Select(t=w2386, s=w2383, f=w2387) -> (s? t:f=w2385:i32)
              n941 = call "myRIO_BRig_RT__Case_Exp_subState_LC__Reward.vi"("input_spout"=w2382, "input_dataCurrent"=w2374, "input_dataLC"=w2381) -> ()  [unwired: 6 in, 2 out]
              n942 = call "myRIO_BRig_RT_dataCurrent_count_generic.vi"() -> ("output_count_generic"=w2376:i32)  [unwired: 11 in]
              n943 = call "myRIO_BRig_RT_dataCurrent_Tcycle_generic.vi"() -> ("output_Tcycle_generic"=w2377:i32)  [unwired: 11 in]
              n944 = Index Array(array=w2388, index=w2385) -> (element=w2378:u16)
              n945 = call "myRIO_BRig_RT_dataCurrent_iState.vi"() -> ("output_iState"=w2366:i32)  [unwired: 11 in]
              n946 = Replace Array Subset(array=w2374, new element #1=w2371, index #1=w2373, new element #2=u16 0 ("new element/subarray"), index #2=w2376, new element #3=w2378, index #3=w2377, new element #4=u16 1 ("new element/subarray"), index #4=w2366) -> (w2389:u16[])
            }
            frame "SelectReward" {
              n947 = call "myRIO_BRig_RT__Case_Exp_State_Reward.vi"("input_dataCurrent"=w2410, "input_state"=w2407, "input_spout"=w2405) -> ("output_dataCurrent"=w2409:u16[], "output_state"=w2408:T2, "output__L"=w2403:bool, "output__R"=w2404:bool)  [unwired: 9 in]
            }
            frame "SelectRewardPost_pre" {
              # "nRewards"
              # "nRewTrials"
              # "Tcycle"
              # "counter"
              n948 = call "myRIO_BRig_RT_dataBlock_nRewards__L.vi"() -> ("output_nRewards__L"=w2426:i32)  [unwired: 11 in]
              n949 = call "myRIO_BRig_RT_dataBlock_nRewards__R.vi"() -> ("output_nRewards__R"=w2425:i32)  [unwired: 11 in]
              n950 = call "myRIO_BRig_RT_dataCurrent_Tcycle_generic.vi"() -> ("output_Tcycle_generic"=w2445:i32)  [unwired: 11 in]
              n951 = call "myRIO_BRig_RT_dataCurrent_count_generic.vi"() -> ("output_count_generic"=w2447:i32)  [unwired: 11 in]
              n952 = case shown="\"Left\", Default" w2419 {
                tunnel: w2431 -> [w2452 w2456]
                tunnel: [w2451 w2456] -> w2430
                tunnel: [w2453 w2454] -> w2429
                tunnel: w2428 -> [w2453 w2455]
                frame "Left", Default {
                  n953 = Increment(x=w2452) -> (x+1=w2451:u16)
                }
                frame "Right" {
                  n954 = Increment(x=w2455) -> (x+1=w2454:u16)
                }
              }
              "nRewards_Left" <- w2430
              "nRewards_Right" <- w2429
              n955 = Equal?(x=w2419, y=enum16{"Left", "Right"}."Left") -> (x = y?=w2418:bool)
              n956 = Select(t=w2426, s=w2418, f=w2425) -> (s? t:f=w2424:i32)
              n957 = call "myRIO_BRig_RT_dataExp_Tcycle_RewardPost.vi"() -> ("output_Tcycle_RewardPost"=w2441:i32)  [unwired: 11 in]
              n958 = call "myRIO_BRig_RT_dataCurrent_nRewTrials.vi"() -> ("output_nRewTrials"=w2427:i32)  [unwired: 11 in]
              n959 = Index Array(array=w2442, index=w2441) -> (element=w2444:u16)
              n960 = Index Array(array=w2421, index=w2427) -> (element=w2416:u16)
              n961 = Replace Array Subset(array=w2421, new element #1=u16 0 ("new element/subarray"), index #1=w2447, new element #2=w2444, index #2=w2445) -> (w2443:u16[])
              n962 = Replace Array Subset(array=w2423, new element=w2416, index (row)=w2417, index (col)=w2424) -> (w2422:u16[][])
              n963 = local write "nRewards_cur"(w2416) -> ()
            }
            frame "SelectRewardPost" {
              n964 = call "myRIO_BRig_RT__Case_Exp_State_RewardPost.vi"("input_state"=w2471, "input_dataCurrent"=w2474) -> ("output_state"=w2472:T2, "output_dataCurrent"=w2473:u16[])  [unwired: 8 in]
            }
            frame "SelectWrong_pre" {
              # "iState"
              # "Tcycle"
              # "counter"
              n965 = call "myRIO_BRig_RT_dataCurrent_Tcycle_generic.vi"() -> ("output_Tcycle_generic"=w2499:i32)  [unwired: 11 in]
              n966 = call "myRIO_BRig_RT_dataCurrent_count_generic.vi"() -> ("output_count_generic"=w2501:i32)  [unwired: 11 in]
              n967 = call "myRIO_BRig_RT_dataExp_Tcycle_Wrong.vi"() -> ("output_Tcycle_Wrong"=w2497:i32)  [unwired: 11 in]
              n968 = call "myRIO_BRig_RT__Case_Exp_subState_LC__Wrong.vi"("input_spout"=w2493, "input_dataCurrent"=w2494, "input_dataLC"=w2491) -> ()  [unwired: 6 in, 2 out]
              n969 = Index Array(array=w2495, index=w2497) -> (element=w2498:u16)
              n970 = call "myRIO_BRig_RT_dataCurrent_iState.vi"() -> ("output_iState"=w2485:i32)  [unwired: 11 in]
              n971 = Replace Array Subset(array=w2494, new element #1=u16 0 ("new element/subarray"), index #1=w2501, new element #2=w2498, index #2=w2499, new element #3=u16 2 ("new element/subarray"), index #3=w2485) -> (w2496:u16[])
            }
            frame "SelectWrong" {
              n972 = call "myRIO_BRig_RT__Case_Exp_State_Wrong.vi"("input_state"=w2515, "input_dataCurrent"=w2524) -> ("output_state"=w2512:T2, "output_dataCurrent"=w2523:u16[])  [unwired: 8 in]
              n973 = Not Equal?(x=w2515, y=w2512) -> (x != y?=w2514:bool)
              n974 = Select(t=myRIO_BRig_RT__Case_Exp_stateList."SelectWrong_post" ("Enum"), s=w2514, f=w2512) -> (s? t:f=w2511:T2)
            }
            frame "SelectWrong_post" {
            }
            frame "SelectTimeout_pre" {
              # "iState"
              # "Tcycle"
              # "counter"
              n975 = xnode "Read/Write Control"("FPGA VI Reference In"=w2551, "error in"=w2550, "SelectionState"=FALSE) -> ("error out"=→"error out 3":errorcluster)  [unwired: 1 out]
              n976 = call "myRIO_BRig_RT_dataCurrent_Tcycle_generic.vi"() -> ("output_Tcycle_generic"=w2573:i32)  [unwired: 11 in]
              n977 = call "myRIO_BRig_RT_dataCurrent_count_generic.vi"() -> ("output_count_generic"=w2571:i32)  [unwired: 11 in]
              n978 = call "myRIO_BRig_RT_dataExp_Tcycle_Timeout.vi"() -> ("output_Tcycle_Timeout"=w2575:i32)  [unwired: 11 in]
              n979 = call "myRIO_BRig_RT__Case_Exp_subState_LC__Timeout.vi"("input_spout"=w2566, "input_dataCurrent"=w2567, "input_dataLC"=w2565) -> ()  [unwired: 6 in, 2 out]
              n980 = Index Array(array=w2569, index=w2575) -> (element=w2574:u16)
              n981 = call "myRIO_BRig_RT_dataCurrent_iState.vi"() -> ("output_iState"=w2559:i32)  [unwired: 11 in]
              n982 = Replace Array Subset(array=w2567, new element #1=u16 0 ("new element/subarray"), index #1=w2571, new element #2=w2574, index #2=w2573, new element #3=u16 3 ("new element/subarray"), index #3=w2559) -> (w2570:u16[])
            }
            frame "SelectTimeout" {
              n983 = call "myRIO_BRig_RT__Case_Exp_State_Timeout.vi"("input_dataLC"=w2594, "input_LC"=w2595, "input_state"=w2585, "input_dataCurrent"=w2600) -> ("output_state"=w2586:T2, "output_dataCurrent"=w2599:u16[])  [unwired: 5 in, 1 out]
              n984 = Not Equal?(x=w2585, y=w2586) -> (x != y?=w2589:bool)
              n985 = Select(t=myRIO_BRig_RT__Case_Exp_stateList."SelectTimeout_post" ("Enum"), s=w2589, f=w2586) -> (s? t:f=w2587:T2)
            }
            frame "SelectTimeout_post" {
            }
            frame "endTrial1" {
              # "Update dataBlock"
              n986 = call "myRIO_BRig_RT__Case_Exp_State_endTrial1.vi"("input_spout"=w2633, "input_dataBlock"=w2632, "input_dataCurrent"=w2630) -> ("output_dataBlock"=w2631:u16[][], "output_dataCurrent"=w2629:u16[])  [unwired: 7 in]
            }
            frame "endTrial2" {
              # "update dataTrial"
              n987 = call "myRIO_BRig_RT__Case_Exp_State_endTrial2.vi"("input_spout"=w2652, "input_dataTrial"=w2656, "input_dataCurrent"=w2654) -> ("output_dataTrial"=w2655:u16[][], "output_dataCurrent"=w2653:u16[])  [unwired: 7 in]
            }
            frame "endTrial3" {
              w2682 = myRIO_BRig_RT__Case_Exp_stateList."endBlock" ("Enum")
              # "nRewTrials"
              # "iTrial"
              # "I_blockUntilReward"
              # "TPB"
              # "end block?"
              n988 = local read "STOP_endTrial"() -> (w2680:bool)
              n989 = local read "STOP_abort"() -> (w2679:bool)
              n990 = xnode "Read/Write Control"("FPGA VI Reference In"=w2668, "error in"=w2667, "SelectionState"=FALSE) -> ("error out"=→"error out 2":errorcluster)  [unwired: 1 out]
              n991 = local read "START"() -> (w2677:bool)
              n992 = call "myRIO_BRig_RT_dataExp_IblockUntilReward.vi"() -> ("output_I_blockUntilReward"=w2689:i32)  [unwired: 11 in]
              n993 = Index Array(array=w2673, index=w2689) -> (element=w2669:u16)
              n994 = Not(x=w2677) -> (.not. x?=w2678:bool)
              n995 = Not Equal To 0?(x=w2669) -> (x != 0?=w2687:bool)
              n996 = Compound Arithmetic op=OR(w2680, w2678, w2679) -> (w2681:bool)
              n997 = call "myRIO_BRig_RT_dataCurrent_nRewTrials.vi"() -> ("output_nRewTrials"=w2685:i32)  [unwired: 11 in]
              n998 = call "myRIO_BRig_RT_dataCurrent_iTrial.vi"() -> ("output_iTrial"=w2686:i32)  [unwired: 11 in]
              n999 = Select(t=w2685, s=w2687, f=w2686) -> (s? t:f=w2684:i32)
              n1000 = call "myRIO_BRig_RT_dataCurrent_TpB.vi"() -> ("output_TpB"=w2688:i32)  [unwired: 11 in]
              n1001 = Index Array(array=w2674, index #1=w2688, index #2=w2684) -> (element #1=w2675:u16, element #2=w2676:u16)
              n1002 = Less Or Equal?(x=w2675, y=w2676) -> (x <= y?=w2672:bool)
              n1003 = Select(t=w2682, s=w2672, f=myRIO_BRig_RT__Case_Exp_stateList."empty_endTrial1" ("Enum")) -> (s? t:f=w2683:T2)
              n1004 = Select(t=w2682, s=w2681, f=w2683) -> (s? t:f=w2670:T2)
            }
            frame "endBlock" {
              # "R"
              # "L"
              # "idxDataBlock"
              n1005 = Equal?(x=w2713, y=enum16{"Left", "Right"}."Left") -> (x = y?=w2712:bool)
              n1006 = call "myRIO_BRig_RT_dataCurrent_idxDataBlockL.vi"() -> ("output_idxDataBlock__L"=w2716:i32)  [unwired: 11 in]
              n1007 = call "myRIO_BRig_RT_dataCurrent_idxDataBlockR.vi"() -> ("output_idxDataBlock__R"=w2715:i32)  [unwired: 11 in]
              n1008 = Increment(x=w2707) -> (x+1=w2706:i32)
              n1009 = Select(t=w2716, s=w2712, f=w2715) -> (s? t:f=w2710:i32)
              n1010 = To Unsigned Word Integer(number=w2706) -> (unsigned 16bit integer=w2708:u16)
              n1011 = local read "START"() -> (w2736:bool)
              n1012 = local read "STOP_endBlock"() -> (w2731:bool)
              n1013 = local read "STOP_endTrial"() -> (w2734:bool)
              n1014 = local read "STOP_abort"() -> (w2733:bool)
              n1015 = Replace Array Subset(array=w2711, new element=w2708, index=w2710) -> (w2709:u16[])
              n1016 = Not(x=w2736) -> (.not. x?=w2735:bool)
              n1017 = Compound Arithmetic op=OR(w2735, w2731, w2734, w2733) -> (w2732:bool)
              n1018 = Select(t=myRIO_BRig_RT__Case_Exp_stateList."endExp" ("Enum"), s=w2732, f=myRIO_BRig_RT__Case_Exp_stateList."empty_endBlock1" ("Enum")) -> (s? t:f=w2740:T2)
            }
            frame "endExp" {
            }
            frame "commConnect" {
              n1019 = call "myRIO_BRig_RT_comm_webdav_connect.vi"("input_password"="Host Password", "input_username"="Host UserName") -> ("output_Iconnected"=w2761:bool, "output_hSession"=w2779:T6)  [unwired: 7 in, 1 out]
              "Connected To Host?" <- w2761
              n1020 = case shown="False" w2761 {
                frame False {
                  n1021 = One Button Dialog(message="Connection Failed!\nData not being saved!") -> ()  [unwired: 1 in, 1 out]
                }
                frame True {
                }
              }
            }
            frame "commUpload_pre" {
              n1022 = Select(t=myRIO_BRig_RT__Case_Exp_stateList."commUpload_dataBlock" ("Enum"), s=w2786, f=myRIO_BRig_RT__Case_Exp_stateList."endTrial3") -> (s? t:f=w2784:T2)
            }
            frame "commUpload_dataBlock" {
              n1023 = call "myRIO_BRig_RT_comm_webdav_uploadFile__data.vi"("input_fileName_prefix"=w2807, "input_fileName"="dataBlock" ("input_filename"), "input_hSession"=w2809) -> ()  [unwired: 8 in, 1 out]
            }
            frame "commUpload_dataCurrent" {
              n1024 = call "myRIO_BRig_RT_comm_webdav_uploadFile__data.vi"("input_fileName_prefix"=w2828, "input_fileName"="dataCurrent" ("input_filename"), "input_hSession"=w2830) -> ()  [unwired: 8 in, 1 out]
            }
            frame "commUpload_dataExp" {
              n1025 = call "myRIO_BRig_RT_comm_webdav_uploadFile__data.vi"("input_fileName_prefix"=w2849, "input_fileName"="dataExp" ("input_filename"), "input_hSession"=w2851) -> ()  [unwired: 8 in, 1 out]
            }
            frame "commUpload_dataLC" {
              n1026 = call "myRIO_BRig_RT_comm_webdav_uploadFile__data.vi"("input_fileName_prefix"=w2870, "input_fileName"="dataLC" ("input_filename"), "input_hSession"=w2872) -> ()  [unwired: 8 in, 1 out]
            }
            frame "commUpload_dataTrial" {
              n1027 = call "myRIO_BRig_RT_comm_webdav_uploadFile__data.vi"("input_fileName_prefix"=w2894, "input_fileName"="dataTrial" ("input_filename"), "input_hSession"=w2896) -> ()  [unwired: 8 in, 1 out]
            }
            frame "saveData_dataBlock" {
              # "idxDataBlockR"
              # "idxDataBlockL"
              n1028 = call "myRIO_BRig_RT_dataCurrent_idxDataBlockL.vi"() -> ("output_idxDataBlock__L"=w2920:i32)  [unwired: 11 in]
              n1029 = call "myRIO_BRig_RT_dataCurrent_idxDataBlockR.vi"() -> ("output_idxDataBlock__R"=w2921:i32)  [unwired: 11 in]
              n1030 = Index Array(array=w2922, index #1=w2920, index #2=w2921) -> (element #1=w2919:u16, element #2=w2918:u16)
              n1031 = Greater?(x=w2919, y=w2918) -> (0:w2917:bool)
              n1032 = Select(t=w2919, s=w2917, f=w2918) -> (s? t:f=w2915:u16)
              n1033 = Increment(x=w2915) -> (x+1=w2914:u16)
              n1034 = To Long Integer(number=w2914) -> (32bit integer=w2913:i32)
              n1035 = Array Subset(array=w2916, length (row)=w2913) -> (w2912:u16[][])  [unwired: 3 in]
              n1036 = call "myRIO_BRig_RT_comm_webdav_saveArrayToFile__2D_u16.vi"("Array"=w2912, "input_filename"="dataBlock") -> ()  [unwired: 10 in]
            }
            frame "saveData_dataCurrent" {
              n1037 = call "myRIO_BRig_RT_comm_webdav_saveArrayToFile__1D_u16.vi"("Array"=w2941, "input_filename"="dataCurrent") -> ()  [unwired: 10 in]
            }
            frame "saveData_dataExp" {
              # "runTime"
              n1038 = Get Date/Time In Seconds() -> (seconds since 1Jan1904=w2969:timestamp)
              n1039 = To Double Precision Float(number=w2969) -> (double precision float=w2968:dbl)
              n1040 = call "myRIO_BRig_RT_dataExp_runTime_seconds.vi"() -> ("output_RunTime_minutes"=w2967:i32)  [unwired: 11 in]
              n1041 = Subtract(x=w2968, y=w2966) -> (x-y=w2963:dbl)
              n1042 = To Unsigned Word Integer(number=w2963) -> (unsigned 16bit integer=w2962:u16)
              n1043 = Replace Array Subset(array=w2961, new element=w2962, index=w2967) -> (w2964:u16[])
              n1044 = call "myRIO_BRig_RT_comm_webdav_saveArrayToFile__1D_u16.vi"("Array"=w2964, "input_filename"="dataExp") -> ()  [unwired: 10 in]
            }
            frame "saveData_dataLC" {
              n1045 = call "myRIO_BRig_RT_comm_webdav_saveArrayToFile__1D_u16.vi"("Array"=w2988, "input_filename"="dataLC") -> ()  [unwired: 10 in]
            }
            frame "saveData_dataTrial" {
              # "idxTrial"
              n1046 = call "myRIO_BRig_RT_dataCurrent_idxDataTrial.vi"() -> ("output_idxDataTrial"=w3013:i32)  [unwired: 11 in]
              n1047 = Index Array(array=w3014, index=w3013) -> (element=w3010:u16)
              n1048 = Increment(x=w3010) -> (x+1=w3009:u16)
              n1049 = To Long Integer(number=w3009) -> (32bit integer=w3008:i32)
              n1050 = Array Subset(array=w3011, length (row)=w3008) -> (w3012:u16[][])  [unwired: 3 in]
              n1051 = call "myRIO_BRig_RT_comm_webdav_saveArrayToFile__2D_u16.vi"("Array"=w3012, "input_filename"="dataTrial") -> ()  [unwired: 10 in]
            }
            frame "empty_endBlock1" {
            }
            frame "empty_endBlock2" {
            }
            frame "empty_endTrial1" {
            }
            frame "empty_endTrial2" {
            }
            frame "empty_endTrial3" {
            }
            frame "empty_endTrial4" {
            }
            frame "empty_endTrial5" {
            }
          }
          n1052 = case shown="True" w1162 {
            tunnel: w1158 -> [w1185 w1193]
            tunnel: w1161 -> [_ w1189]
            tunnel: w1160 -> [_ w1188]
            tunnel: w1159 -> [_ w1187]
            tunnel: w1128 -> [_ w1186]
            tunnel: [w1185 w1192] -> w1157
            tunnel: w1156 -> [w1184 w1191]
            tunnel: [w1184 w1190] -> w1155
            frame False {
            }
            frame True {
              n1053 = call "myRIO_BRig_RT__Case_Exp__recordLick.vi"("intput_state__trialEnd"=w1186, "intput_state__trialStart"=w1187, "input_lick__R"=w1188, "input_lick__L"=w1189, "input_dataCurrent"=w1191, "input_dataLick"=w1193) -> ("output_dataCurrent"=w1190:u16[], "output_dataLick"=w1192:u16[][])  [unwired: 4 in]
            }
          }
          n1054 = Or(x=w1130, y=w1131) -> (x .or. y?=w1117:bool)
          n1055 = Or(x=w1134, y=w1114) -> (x .or. y?=w1103:bool)
          n1056 = Or(x=w1113, y=w1135) -> (x .or. y?=w1129:bool)
          n1057 = Or(x=w1133, y=w1132) -> (x .or. y?=w1118:bool)
          n1058 = Or(x=w1163, y="STOP_abort") -> (x .or. y?=w1165:bool)
          n1059 = Or(x=w1092, y=w1093) -> (x .or. y?=w1090:bool)
          n1060 = Or(x=w1094, y=w1093) -> (x .or. y?=w1091:bool)
          n1061 = xnode "Read/Write Control"("FPGA VI Reference In"=w1105, "error in"=w1104, "A1_SR"=w1118, "A3_SL"=w1117, "A6_Act"="Recording_p2", "audioTrigger_L"=w1103, "audioAmp_L"=w1144, "audioFreq_L_kHz"=w1112, "audioTrigger_R"=w1129, "audioAmp_R"=w1145, "audioFreq_R_kHz"=w1146, "laserledMTrig"=w1090, "laserMTrig"=w1091) -> ("FPGA VI Reference Out"=w1154:refnum<k20>, "error out"=w1153:errorcluster)
          n1062 = node-c288() -> ()  [unwired: 1 in, 1 out]
          "cState" <- w1159
        }
        n1063 = node-c288(w1048) -> ()  [unwired: 1 out]
        n1064 = flat-sequence {
          tunnel: w1044 -> [w1082]
          tunnel: w1043 -> [w1081]
          tunnel: [w1080] -> w1036
          tunnel: [w1079] -> w1035
          tunnel: [w1085] -> w1037
          tunnel: [w1086] -> w1042
          tunnel: w1036 -> [w1086]
          tunnel: w1035 -> [w1085]
          frame #0 {
            w1076 = u8 0
            w1077 = u16 0 ("AudioLeft_phase_inc")
            w1078 = FALSE
            n1065 = xnode "Read/Write Control"("FPGA VI Reference In"=w1082, "error in"=w1081, "Counts_Reset"=TRUE, "audioTrigger_L"=w1078, "audioFreq_L_kHz"=w1076, "audioAmp_L"=w1077, "audioTrigger_R"=w1078, "audioFreq_R_kHz"=w1076, "audioAmp_R"=w1077, "A3_SL"=w1078, "A1_SR"=w1078, "A6_Act"=w1078) -> ("FPGA VI Reference Out"=w1080:refnum<k20>, "error out"=w1079:errorcluster)
          }
          frame #1 {
            w1084 = FALSE ("START")
            n1066 = local write "START"(w1084) -> ()
            n1067 = local write "STOP_endTrial"(w1084) -> ()
            n1068 = local write "STOP_endBlock"(w1084) -> ()
          }
        }
        n1069 = stacked-sequence {
          tunnel: w1020 -> [w1056 _]
          tunnel: w1018 -> [w1057 _]
          tunnel: w1017 -> [_ w1062]
          tunnel: w1016 -> [_ w1061]
          tunnel: w1015 -> [_ w1060]
          tunnel: w1014 -> [w1050 _]
          frame #0 {
            n1070 = call "myRIO_BRig_RT_dataCurrent_idxDataLick.vi"() -> ("output_idxDataLick"=w1051:i32)  [unwired: 11 in]
            n1071 = Index Array(array=w1050, index=w1051) -> (element=w1053:u16)
            n1072 = Increment(x=w1053) -> (x+1=w1054:u16)
            n1073 = call "myRIO_BRig_RT_comm_webdav_saveArrayToFile__1D_u16.vi"("Array"=w1057, "input_filename"="dataMTrig") -> ()  [unwired: 10 in]
            n1074 = To Long Integer(number=w1054) -> (32bit integer=w1052:i32)
            n1075 = Array Subset(array=w1056, length (row)=w1052) -> (w1055:u16[][])  [unwired: 3 in]
            n1076 = call "myRIO_BRig_RT_comm_webdav_saveArrayToFile__2D_u16.vi"("Array"=w1055, "input_filename"="dataLick") -> ()  [unwired: 10 in]
          }
          frame #1 {
            n1077 = case shown="True" w1062 {
              tunnel: w1061 -> [_ w1064]
              tunnel: w1060 -> [_ w1063]
              frame False {
              }
              frame True {
                n1078 = stacked-sequence {
                  tunnel: w1064 -> [w1066 w1073 w1075]
                  tunnel: w1063 -> [w1067 w1072 _]
                  frame #0 {
                    n1079 = call "myRIO_BRig_RT_comm_webdav_uploadFile__announce.vi"("input_addText"=TRUE, "input_fileName_prefix"=w1067, "intput_fileName"="curExp_end", "intput_hSession"=w1066) -> ("output_Isuccess"=w1065:bool)  [unwired: 6 in, 1 out]
                    n1080 = case shown="True" w1065 {
                      frame False {
                        n1081 = One Button Dialog(message="!!! Warning !!! Your data is located at C:\\BehaviorRig\\commTransfer") -> ()  [unwired: 1 in, 1 out]
                      }
                      frame True {
                        n1082 = Wait (ms)(milliseconds to wait=u32 20) -> ()  [unwired: 1 out]
                      }
                    }
                  }
                  frame #1 {
                    n1083 = call "myRIO_BRig_RT__endExp_sendData.vi"("input_fileName_prefix"=w1072, "input_hSession"=w1073) -> ()  [unwired: 8 in, 2 out]
                  }
                  frame #2 {
                    n1084 = local write "Connected To Host?"(FALSE ("Connected To Host?")) -> ()
                    n1085 = call <vilib>:"Close Session.vi"("session handle"=w1075) -> ()  [unwired: 14 in, 1 out]
                  }
                }
              }
            }
          }
        }
      }
    }
    n1086 = local read "STOP_abort"() -> (w30:bool)
  }
  n1087 = xnode "Read/Write Control"("FPGA VI Reference In"=w8, "error in"=w7, "FPGA_Stop"=TRUE) -> ("FPGA VI Reference Out"=w13:refnum<k20>, "error out"=w14:errorcluster)
  n1088 = xnode "Close FPGA VI Reference"("FPGA VI Reference In"=w13, "error in"=w14) -> ("error out"=w12:errorcluster)
  n1089 = call <vilib>:"Reset myRIO.vi"("error in (no error)"=w12) -> ()  [unwired: 10 in, 1 out]
